vi "newlane2.vi"(11 "predict":bool=TRUE) -> ()   [LabVIEW 2012]
uses:
  G_NAV.vi
  G_VEH.vi
  G_PATH.vi
  G_SEN.vi
  <vilib>/Analysis/Matrix/Numeric/Conversions/Array To Matrix - RA2.vi
  <vilib>/Analysis/7linalg.llb/Real SVD Decomposition.vi
  <vilib>/Analysis/NI_AALPro.lvlib
  <vilib>/Analysis/Matrix/NI_Matrix.lvlib
panel:
  out "M6006":T1={"GPSTime"=22892800.0, "attitude[2]"=-0.6123908162117004, "lcc[0]"=-970.4720458984375, "lcc[1]"=200.52362060546875, "heading_GPS"=-0.610690712928772} {"GPSTime" format="%#_6f"}
  out "x-y":dbl[](array[numeric])
  out "min value 2":dbl
  out "min value":dbl
  out "Waveform Chart":dbl(graph)
  out "cost":dbl
  out "output array":dbl[][](array[numeric])
  out "rd0 2":dbl
  out "RXY":dbl[](array[numeric])=[73.97207949000635, 12.402968176654849, 69.25942811748455]
  out "map_track":dbl[][](array[numeric])=[[-0.6687401515638595, -3.551350516814976], [-1.1601880006125764, -3.4580278333550782], [-1.6512488590649952, -3.3629580799680854], [-2.1418835557610314, -3.265964418362822], [-2.6320529195405924, -3.1668700102479344], [-3.12171777924361, -3.0654980173321356], [-3.6108389637099756, -2.961671601324125], [-4.250355012057505, -2.8217269001890974], [-4.733554194697693, -2.693195492254268]]
  out "k 2":i32
  out "j 2":i32
  out "i 2":i32
  out "mapidx":i32[](array[numeric])
  out "ymin":dbl=-6.0
  out "ymax":dbl=12.0
  out "reverse":bool
  out "track":dbl[][](array[numeric])=[[-0.6687401515638595, -3.551350516814976], [-1.1601880006125764, -3.4580278333550782], [-1.6512488590649952, -3.3629580799680854], [-2.1418835557610314, -3.265964418362822], [-2.6320529195405924, -3.1668700102479344], [-3.12171777924361, -3.0654980173321356], [-3.6108389637099756, -2.961671601324125], [-4.250355012057505, -2.8217269001890974], [-4.733554194697693, -2.693195492254268], [-5.215089885143842, -2.558342659026822], [-5.693483406062963, -2.4115492889016945], [-6.167256080122039, -2.24719627027381], [-6.634929229988109, -2.059664491538052], [-7.095024178328142, -1.8433348410893422], [-7.546062247809149, -1.5925882073226139], [-7.98656476109811, -1.301805478632852], [-8.415053040862054, -0.9653675434148765], [-8.830048409767974, -0.5776552900636165], [-9.230072190482858, -0.133049606974057], [-9.61364570567371, 0.3740686174589265], [-9.97929027800753, 0.949318494840405], [-10.386059580111024, 1.7242186788508236], [-10.53357405922493, 2.2019628347040774], [-10.66851200140239, 2.6835902739278463], [-10.772007434080049, 3.1749262819640283], [-10.825194384694537, 3.6817961442544633], [-10.809206880682517, 4.210025146240928], [-10.705178949480636, 4.765438573365376], [-10.494244618525542, 5.353861711069529], [-10.157537915253862, 5.981119844795286], [-9.676192867102248, 6.653038259984428], [-8.946295802610212, 7.461572105302583], [-8.539313408094966, 7.752602995705581], [-8.110420661696207, 8.015244834208291], [-7.660232732059987, 8.25029468946181], [-7.189364787832295, 8.458549630117131], [-6.698431997659123, 8.640806724825243], [-6.188049530186491, 8.797863042237132], [-5.658832554060375, 8.930515651003796], [-5.11139623792681, 9.039561619776274], [-4.546355750431802, 9.12579801720561], [-3.9643262602213256, 9.190021911942688], [-3.3659229359414162, 9.233030372638604], [-2.7517609462380523, 9.25562046794435], [-2.122455459757251, 9.258589266510917], [-1.4786216451450183, 9.242733836989292], [-0.8208746710473604, 9.208851248030518], [-0.1498297061102689, 9.157738568285591], [0.5338980810202378, 9.090192866405497], [1.229693521698167, 9.007011211041284], [1.9369414472775146, 8.908990670843883], [2.6550266891122614, 8.796928314464337], [3.383334078556428, 8.671621210553642], [4.121248446963983, 8.53386642776284], [4.868154625688948, 8.384461034742866], [5.623437446085289, 8.224202100144819], [6.386481739507029, 8.053886692619635], [7.156672337308164, 7.874311880818305], [7.838146127104554, 7.70968069378327], [8.321781606815595, 7.582803343212244], [8.805290536895978, 7.45544776805299], [9.287663918083021, 7.323801011645703], [9.76789275111402, 7.18405011733063], [10.244968036726283, 7.032382128447967], [10.717880775657084, 6.864984088337955], [11.18562196864372, 6.678043040340844], [11.647182616423507, 6.4677460277968315], [12.101553719733744, 6.230280094046104], [12.547726279311707, 5.961832282428966], [12.984691295894704, 5.658589636285609], [13.411439770220039, 5.3167391989562285], [13.939637565704926, 4.818324597988705], [14.177469695018669, 4.377621822306417], [14.370305638929839, 3.9092831916317614], [14.522185803389362, 3.415790251277338], [14.637150594348116, 2.8996245465557346], [14.719240417757044, 2.363267622779441], [14.77249567956704, 1.8092010252611073], [14.800956785728996, 1.2399062993133256], [14.808664142193827, 0.6578649902486369], [14.799658154912459, 0.06555864337958095], [14.777979229835777, -0.5345311959811911]]
  out "xyhc":T2={"c_idx"=71, "xc"=-91.48037348905598, "yc"=-434.27857700428615, "hc"=-0.4484199308552679, "xc_path"=12.43286899562552}
  in  "usewpt":bool=TRUE
  out "left":dbl
  out "right":dbl
  out "lane left":dbl
  out "lane right":dbl
  out "maxradius":dbl=0.125
  out "Numeric":i32
  out "abrd0":dbl[][](array[numeric])
  out "center":dbl
  out "lane shift":dbl
  out "mylane":i16
  out "min lane length":dbl=0.125
  out "lineseed2":dbl[][](array[numeric])
  out "lineseed1":dbl[][](array[numeric])
  out "lineseed0":dbl[][](array[numeric])
  out "lineseedorigin":dbl[](array[numeric])
  out "den":dbl
  out "xx":dbl[](array[numeric])
  out "t2x":dbl
  out "xt":dbl[](array[numeric])
  out "rdi":dbl[](array[numeric])
  out "cta":dbl
  out "fitting?":bool
  out "mode":dbl
  out "rd0":dbl
  out "b":dbl
  out "a":dbl
  out "y":dbl[](array[numeric])
  out "x":dbl[](array[numeric])
  out "i":i32
  out "j":i32
  out "k":i32
  out "line":dbl[][](array[numeric])
  out "time[sec]":dbl
  out "count":cluster{dbl[][]}[](array[cluster])
  out "idxall":cluster{i32[]}[](array[cluster])
  out "yseed":dbl[](array[numeric])
  out "min lane width":dbl=0.125
  out "lane_resol":dbl=0.125
  out "T_threshold":dbl=0.125
  out "T_threshold 2":dbl=0.125
  out "xseed":dbl[](array[numeric])=[5.0, 10.0, 15.0, 20.0, 25.0, 30.0, 35.0]
  out "D_threshold":dbl=0.125
  out "data":dbl[][](array[numeric])
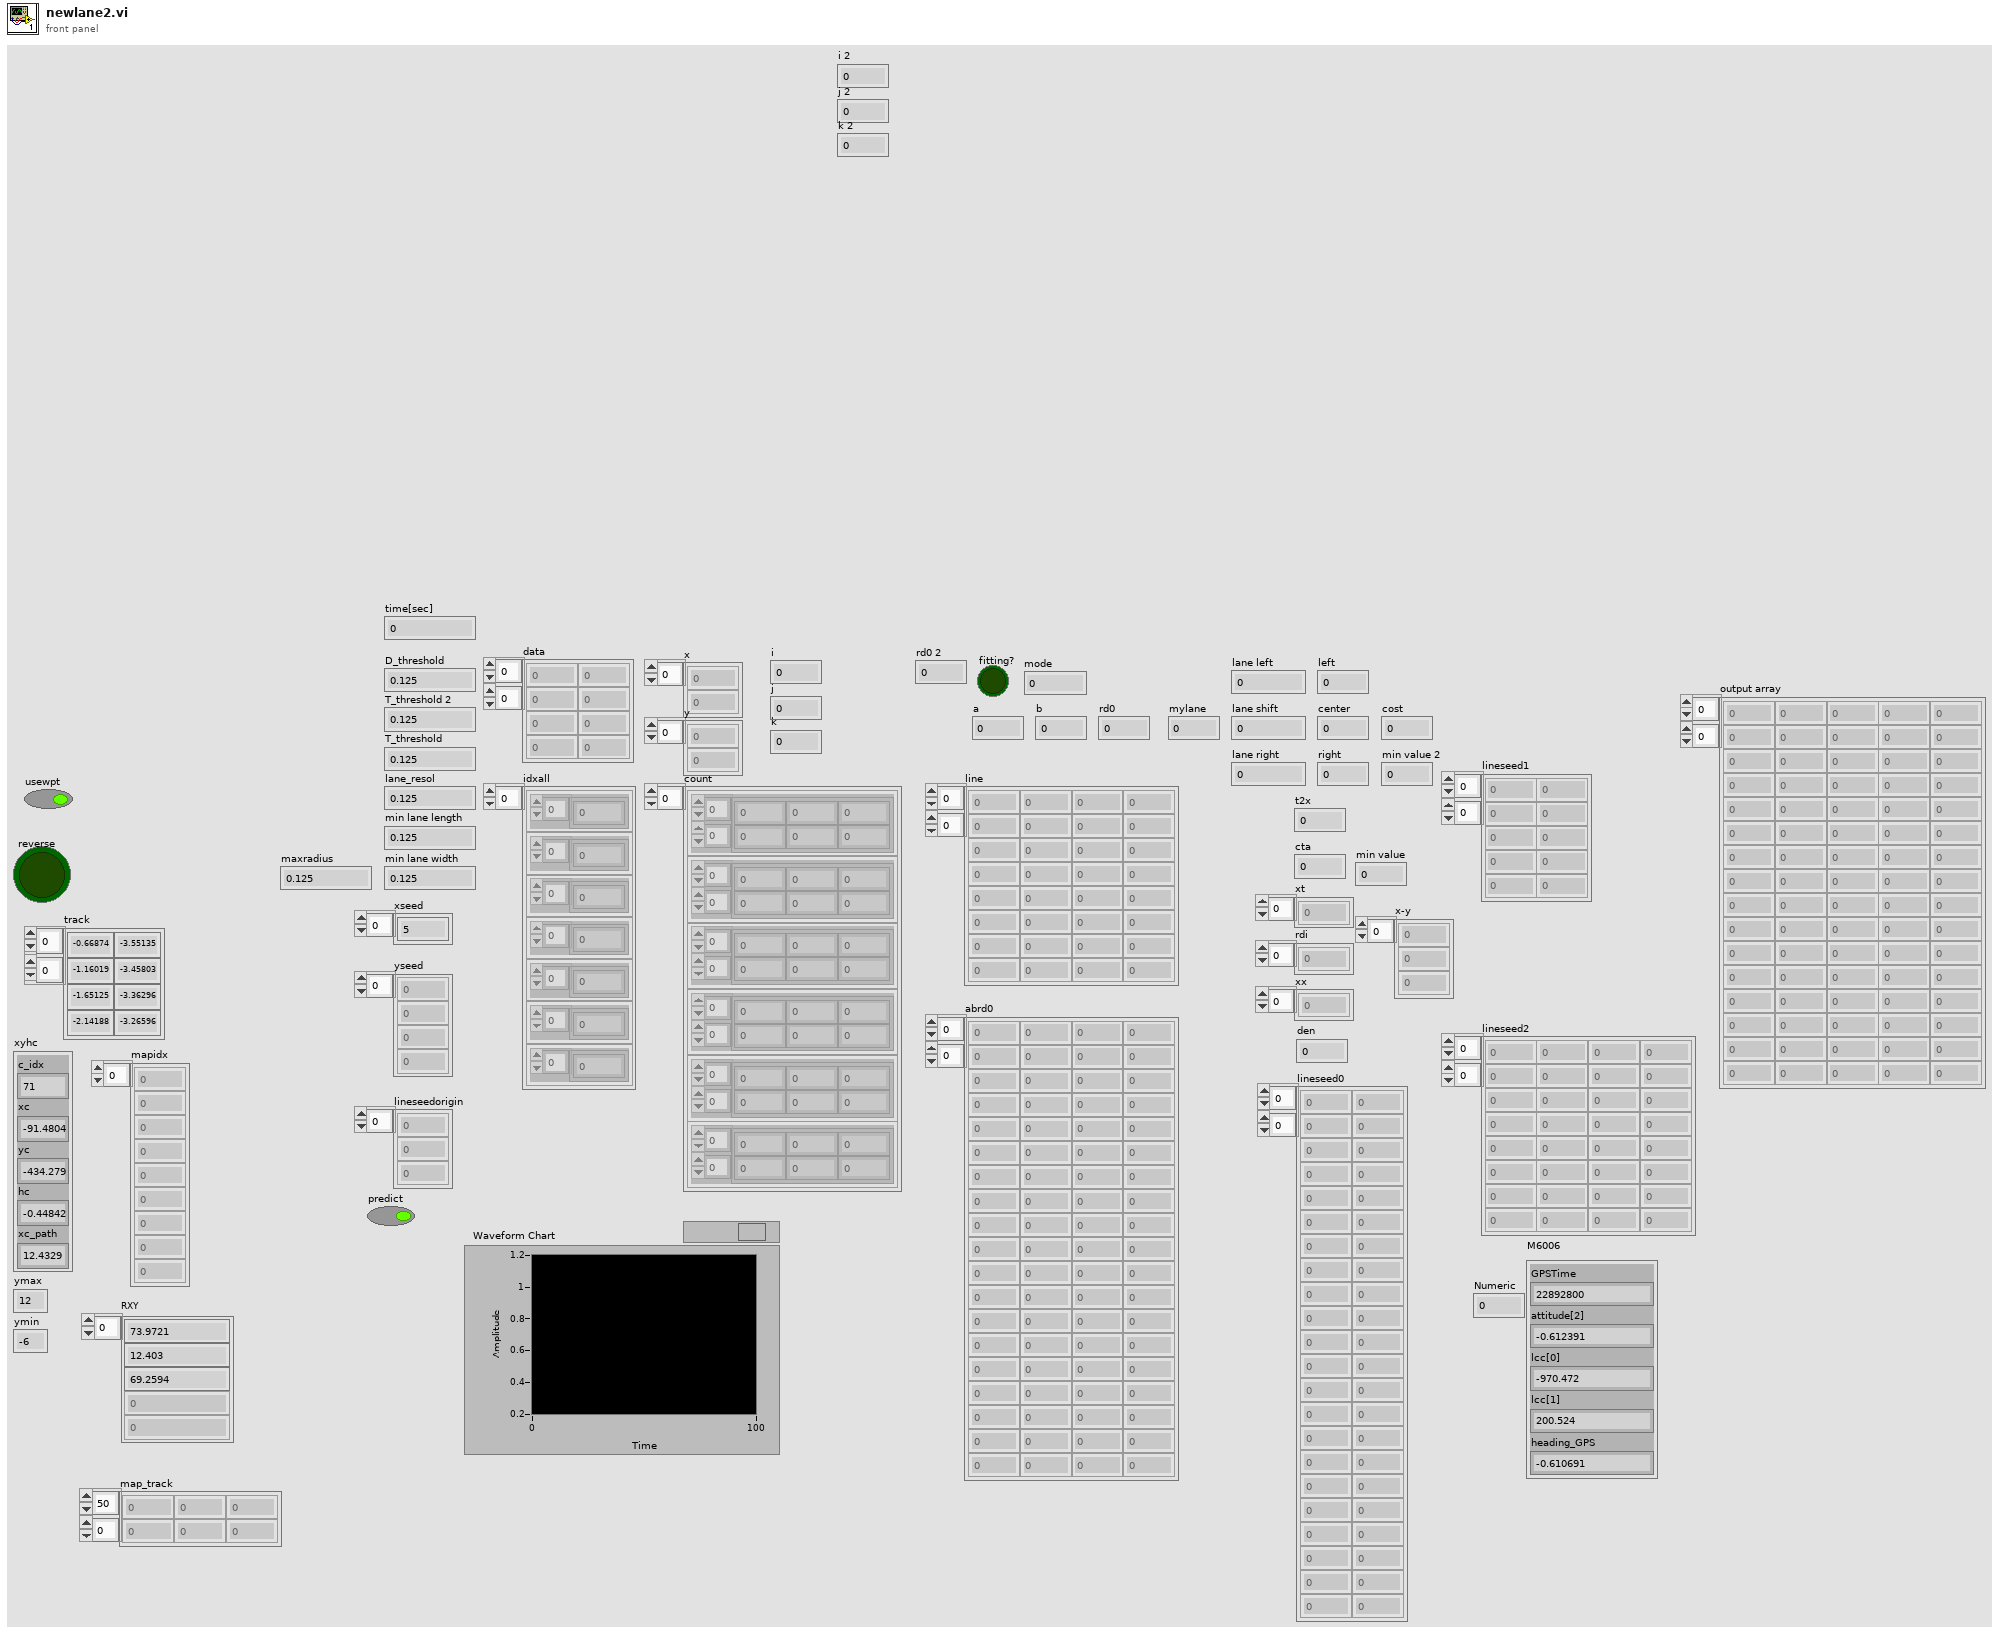
[diagram p1: front panel]
types:
  T1 = cluster{"GPSTime":dbl, "attitude[2]":dbl, "lcc[0]":dbl, "lcc[1]":dbl, "heading_GPS":dbl}
  T2 = cluster{"c_idx":i32, "xc":dbl, "yc":dbl, "hc":dbl, "xc_path":dbl}
  T3 = cluster{"idx":i32, "x":dbl, "y":dbl, "h":dbl, "x_path":dbl}
  T4 = cluster{"Steer_input":dbl, "Steer_output":dbl, "VS_des":dbl, "VS_can":dbl, "heading":dbl, "auto":bool, "run":bool, "x":dbl, "y":dbl}
  T5 = typedef "NI_Matrix.lvlib/RealMatrix.ctl" = dbl[][]
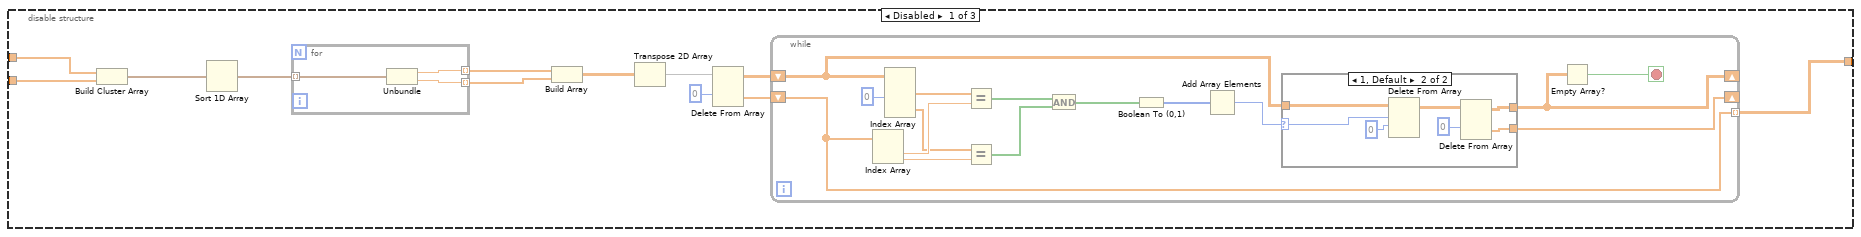
[diagram p5: hidden frame]
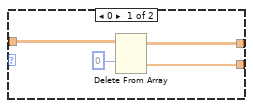
[diagram p6: hidden frame]
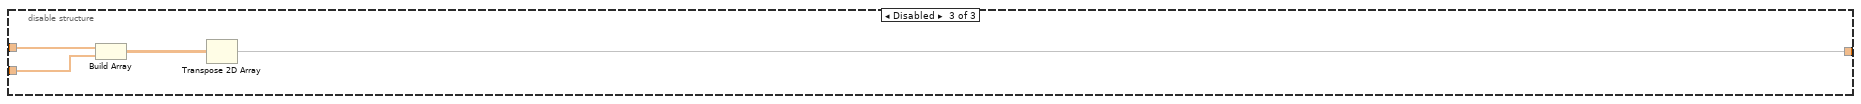
[diagram p8: hidden frame]
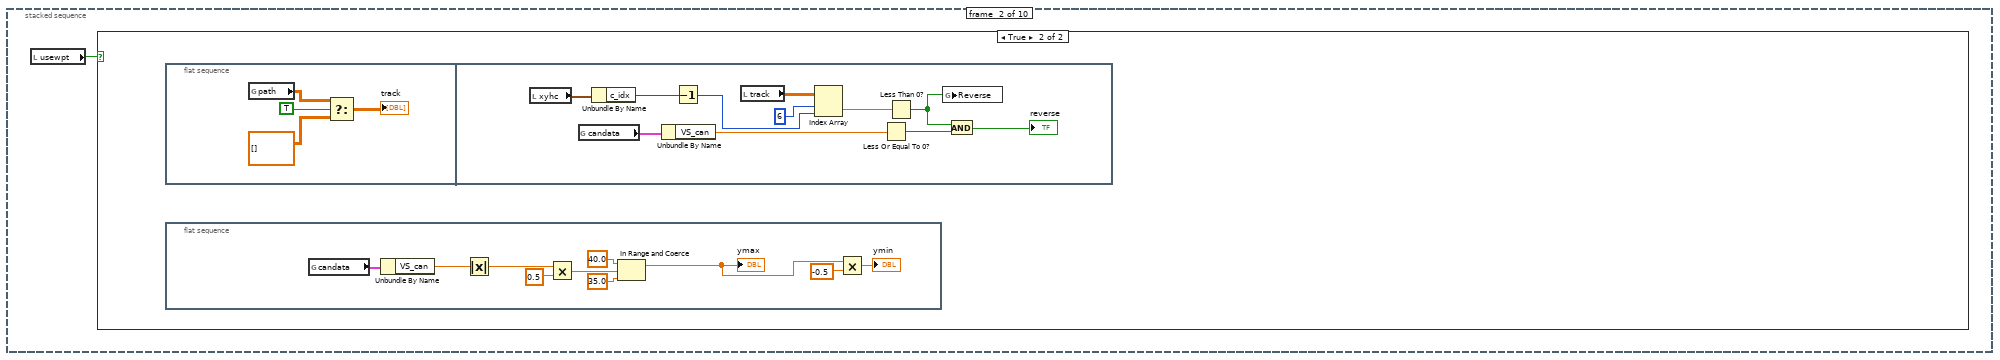
[diagram p11: hidden frame]
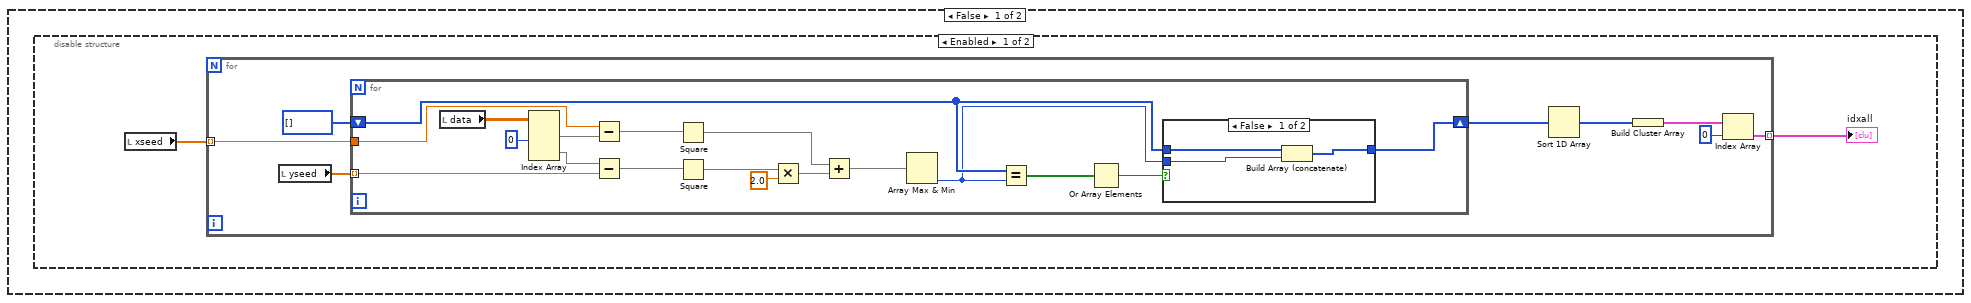
[diagram p12: hidden frame]
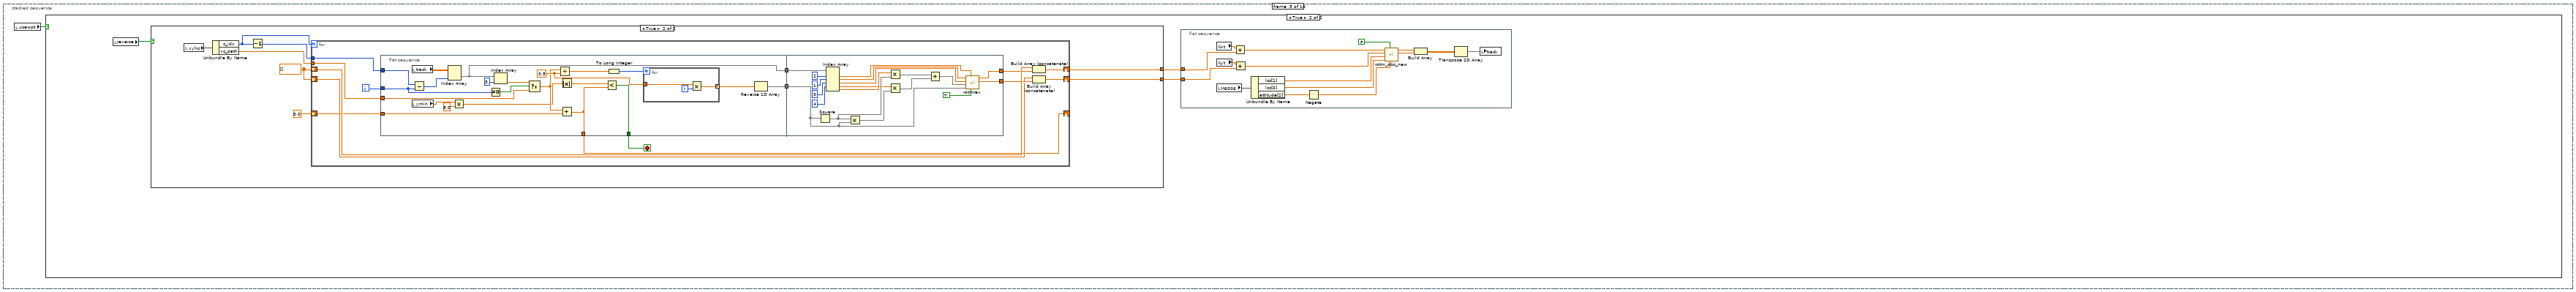
[diagram p15: hidden frame]
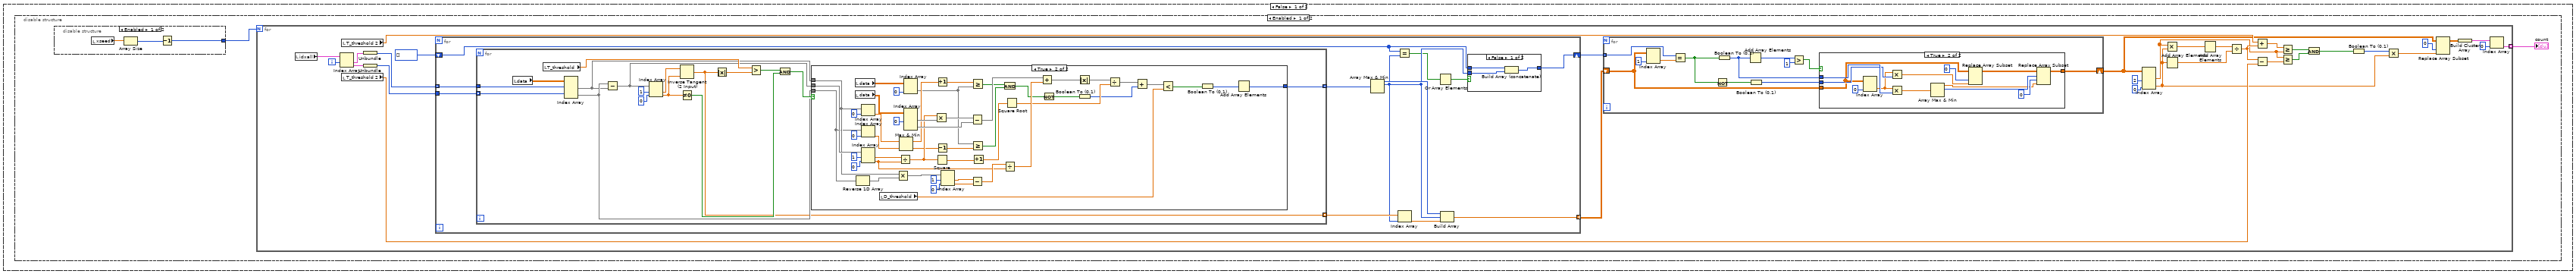
[diagram p16: hidden frame]
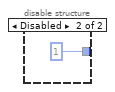
[diagram p20: hidden frame]
diagram:
  n1 = flat-sequence {
    tunnel: [w4] -> w2
    tunnel: [w11] -> w3
    tunnel: w2 -> [w11]
    tunnel: w3 -> [w57]
    tunnel: [w58] -> w1
    tunnel: w1 -> [w2451]
    frame #0 {
      n2 = Tick Count (ms)() -> (millisecond timer value=w4:u32)
    }
    frame #1 {
      n3 = global read "G_VEH.vi" "xyhc"() -> (w7:T3)
      n4 = global read "G_PATH.vi" "lane_init"() -> (w6:bool)
      n5 = global read "G_NAV.vi" "M6006"() -> (→"M6006":T1)
      n6 = Select(t=w7, s=TRUE ("B_track"), f=T2 {"c_idx"=0, "xc"=0.0, "yc"=0.0, "hc"=0.0, "xc_path"=0.0}) -> (s? t:f=→"xyhc":T2)
      n7 = case shown="False" w6 {
        frame False {
          n8 = flat-sequence {
            frame #0 {
              n9 = Multiply(x=5.0 ("D_threshold"), y=3.141592653589793) -> (x*y=w23:dbl)
              n10 = Multiply(x=15.0 ("D_threshold"), y=3.141592653589793) -> (x*y=w17:dbl)
              n11 = Divide(x=w17, y=180.0) -> (x/y=→"T_threshold":dbl)
              n12 = Divide(x=w23, y=180.0) -> (x/y=→"T_threshold 2":dbl)
              "D_threshold" <- 0.125 ("D_threshold")
              "lane_resol" <- 0.25 ("D_threshold")
              "min lane width" <- 2.5 ("D_threshold")
              "min lane length" <- 3.5 ("min lane length")
              "maxradius" <- 75.0 ("maxradius")
            }
            frame #1 {
              w31 = dbl[] [5.0, 10.0, 15.0, 20.0, 25.0, 30.0, 35.0]  # xseed
              w36 = 10.0
              w39 = 10.0
              n13 = local read "D_threshold"() -> (w33:dbl)
              n14 = Negate(x=w39) -> (-x=w38:dbl)
              n15 = Negate(x=w36) -> (-x=w37:dbl)
              n16 = Multiply(x=w33, y=4.0) -> (x*y=w41:dbl)
              n17 = Multiply(x=w33, y=1.0) -> (x*y=w35:dbl)
              n18 = Array Subset(array=w31, index=0, length=5) -> (→"xseed":dbl[])
              n19 = while {
                tunnel: w41 -> [w56]
                tunnel: [w50] -> w40 mode=indexing
                tunnel: w39 -> [w51]
                tunnel: w38 -> [w52]
                i -> [w55]
                stop <- w53 stop-if-true
                n20 = Multiply(x=w56, y=w55) -> (x*y=w54:dbl)
                n21 = Add(x=w52, y=w54) -> (x+y=w50:dbl)
                n22 = Less Or Equal?(x=w51, y=w50) -> (x <= y?=w53:bool)
              }
              "yseed" <- w40
              n23 = while {
                tunnel: w35 -> [w49]
                tunnel: [w43] -> w32 mode=indexing
                tunnel: w36 -> [w44]
                tunnel: w37 -> [w45]
                i -> [w48]
                stop <- w46 stop-if-true
                n24 = Multiply(x=w49, y=w48) -> (x*y=w47:dbl)
                n25 = Add(x=w45, y=w47) -> (x+y=w43:dbl)
                n26 = Less Or Equal?(x=w44, y=w43) -> (x <= y?=w46:bool)
              }
              "lineseedorigin" <- w32
            }
          }
          n27 = global write "G_PATH.vi" "lane_init"(TRUE ("lane_init")) -> ()
        }
        frame True {
        }
      }
    }
    frame #2 {
      n28 = stacked-sequence {
        tunnel: [w60 _ _ _ _ _ _ _ _ _] -> w58
        tunnel: w57 -> [w59 _ _ _ _ _ _ _ _ _]
        frame #0 {
          n29 = flat-sequence {
            tunnel: [w164] -> w60
            tunnel: w59 -> [w163]
            frame #0 {
              n30 = disable-structure shown="Enabled" {
                frame Enabled {
                  n31 = local read "M6006"() -> (w66:T1)
                  n32 = Unbundle By Name(w66) -> ("lcc[1]"=w83:dbl, "lcc[0]"=w82:dbl, "attitude[2]"=w81:dbl)
                  n33 = global read "G_SEN.vi" "sensor_lane_log"() -> (w77:dbl[][])
                  n34 = Negate(x=w81) -> (-x=w80:dbl)
                  n35 = Index Array(array=w77, index (col) #1=0 ("disabled index (col)")) -> (element #1=w79:dbl[], element #2=w78:dbl[])  [unwired: 3 in]
                  n36 = call "rotm_obs_new.vi"("angle[rad]"=w80, "y0"=w82, "x0"=w83, "y"=w78, "x"=w79) -> ("rot*(y-y0) 2"=w63:dbl[], "rot*(x-x0)"=w65:dbl[])  [unwired: 3 in, 2 out]
                  n37 = disable-structure shown="Enabled" {
                    disable-tunnel: w65 -> [w90 w94]
                    disable-tunnel: [w88 w94] -> w64
                    disable-tunnel: w63 -> [w87 w93]
                    disable-tunnel: [w85 w93] -> w62
                    frame Enabled {
                      n38 = global read "G_SEN.vi" "sensor_obs"() -> (w92:dbl[][])
                      n39 = Index Array(array=w92, index (col) #1=0 ("disabled index (col)")) -> (element #1=w89:dbl[], element #2=w86:dbl[])  [unwired: 3 in]
                      n40 = Build Array (concatenate)(w90, w89) -> (w88:dbl[])
                      n41 = Build Array (concatenate)(w87, w86) -> (w85:dbl[])
                    }
                    frame Disabled {
                    }
                  }
                  n42 = Multiply(x=w64, y=10.0) -> (x*y=w75:dbl[])
                  n43 = Multiply(x=w62, y=10.0) -> (x*y=w70:dbl[])
                  n44 = Round To Nearest(number=w75) -> (nearest integer value=w74:dbl[])
                  n45 = Round To Nearest(number=w70) -> (nearest integer value=w71:dbl[])
                  n46 = Multiply(x=w71, y=0.1) -> (x*y=w68:dbl[])
                  n47 = Multiply(x=w74, y=-0.1) -> (x*y=w67:dbl[])
                  n48 = disable-structure shown="Enabled" {
                    disable-tunnel: [w95 w138 w159] -> w61
                    disable-tunnel: w68 -> [w105 w137 w162]
                    disable-tunnel: w67 -> [w104 w136 w161]
                    frame Disabled {
                      n49 = Build Cluster Array(w105, w104) -> (w106:cluster{dbl, dbl}[])
                      n50 = Sort 1D Array(array=w106) -> (sorted array=w103:cluster{dbl, dbl}[])
                      n51 = for {
                        tunnel: w103 -> [w135] mode=indexing
                        tunnel: [w134] -> w102 mode=indexing
                        tunnel: [w133] -> w101 mode=indexing
                        n52 = Unbundle(w135) -> (w134:dbl, w133:dbl)
                      }
                      n53 = Build Array(w102, w101) -> (w100:dbl[][])
                      n54 = Transpose 2D Array(2D array=w100) -> (transposed array=w99:dbl[][])
                      n55 = Delete From Array(array=w99, index (row)=0) -> (deleted portion=w98:dbl[], array with subset deleted=w97:dbl[][])  [unwired: 2 in]
                      n56 = while {
                        shift-right: [w109] -> _
                        shift-left: w98 -> [w108]
                        shift-right: [w111] -> _
                        shift-left: w97 -> [w112]
                        tunnel: [w108] -> w95 mode=indexing
                        stop <- w110 stop-if-true
                        n57 = Index Array(array=w108) -> (element #1=w119:dbl, element #2=w117:dbl)  [unwired: 2 in]
                        n58 = Index Array(array=w112, index (col) #1=0 ("disabled index (col)")) -> (element #1=w120:dbl[], element #2=w118:dbl[])  [unwired: 3 in]
                        n59 = Equal?(x=w120, y=w119) -> (x = y?=w116:bool[])
                        n60 = Equal?(x=w118, y=w117) -> (x = y?=w115:bool[])
                        n61 = And(x=w116, y=w115) -> (x .and. y?=w114:bool[])
                        n62 = Boolean To (0,1)(Boolean=w114) -> (0, 1=w113:i16[])
                        n63 = Add Array Elements(numeric array=w113) -> (sum=w107:i16)
                        n64 = case shown="1, Default" w107 {
                          selector: w107 -> [_ w131]
                          tunnel: w112 -> [w125 w132]
                          tunnel: [w124 w129] -> w111
                          tunnel: [w123 w128] -> w109
                          frame 0 {
                            n65 = Delete From Array(array=w125, index (row)=0) -> (deleted portion=w123:dbl[], array with subset deleted=w124:dbl[][])  [unwired: 2 in]
                          }
                          frame 1, Default {
                            n66 = Delete From Array(array=w132, length=w131, index (row)=0) -> (array with subset deleted=w130:dbl[][])  [unwired: 1 in, 1 out]
                            n67 = Delete From Array(array=w130, index (row)=0) -> (deleted portion=w128:dbl[], array with subset deleted=w129:dbl[][])  [unwired: 2 in]
                          }
                        }
                        n68 = Empty Array?(array=w111) -> (empty?=w110:bool)
                      }
                    }
                    frame Enabled {
                      n69 = Build Cluster Array(w137, w136) -> (w142:cluster{dbl, dbl}[])
                      n70 = Sort 1D Array(array=w142) -> (sorted array=w141:cluster{dbl, dbl}[])
                      n71 = for {
                        tunnel: w141 -> [w154] mode=indexing
                        shift-right: [w150] -> _
                        shift-left: dbl[] [-1e+18, -1e+18] -> [w149]
                        shift-right: [w152] -> w138
                        shift-left: dbl[][] [] -> [w153]
                        stop <- w143 stop-if-true
                        n72 = Unbundle(w154) -> (w147:dbl, w148:dbl)
                        n73 = Build Array(w147, w148) -> (w150:dbl[])
                        n74 = Greater?(x=w147, y=40.0) -> (0:w143:bool)
                        n75 = Equal?(x=w150, y=w149) -> (x = y?=w151:bool[])
                        n76 = And Array Elements(Boolean array=w151) -> (logical AND=w144:bool)
                        n77 = Or(x=w143, y=w144) -> (x .or. y?=w145:bool)
                        n78 = case shown="False" w145 {
                          tunnel: w153 -> [w157 w158]
                          tunnel: w150 -> [w156 _]
                          tunnel: [w155 w158] -> w152
                          frame False {
                            n79 = Build Array (concatenate)(w157, w156) -> (w155:dbl[][])
                          }
                          frame True {
                          }
                        }
                      }
                    }
                    frame Disabled {
                      n80 = Build Array(w162, w161) -> (w160:dbl[][])
                      n81 = Transpose 2D Array(2D array=w160) -> (transposed array=w159:dbl[][])
                    }
                  }
                  "data" <- w61
                }
                frame Disabled {
                }
              }
            }
            frame #1 {
              n82 = disable-structure shown="Enabled" {
                disable-tunnel: [w165 w166] -> w164
                disable-tunnel: w163 -> [_ w166]
                frame Enabled {
                  n83 = Tick Count (ms)() -> (millisecond timer value=w165:u32)
                }
                frame Disabled {
                }
              }
            }
          }
        }
        frame #1 {
          n84 = local read "usewpt"() -> (w167:bool)
          n85 = case shown="True" w167 {
            frame False {
              n86 = disable-structure shown="Enabled" {
                frame Enabled {
                  n87 = local read "xseed"() -> (w169:dbl[])
                  n88 = for {
                    tunnel: w169 -> [w176] mode=indexing
                    tunnel: [w170] -> w168 mode=indexing
                    n89 = local read "yseed"() -> (w177:dbl[])
                    n90 = for {
                      tunnel: w177 -> [w192] mode=indexing
                      tunnel: w176 -> [w179]
                      shift-right: [w184] -> w174
                      shift-left: i32[] [] -> [w185]
                      n91 = local read "data"() -> (w195:dbl[][])
                      n92 = Index Array(array=w195, index (col) #1=0 ("disabled index (col)")) -> (element #1=w178:dbl[], element #2=w193:dbl[])  [unwired: 3 in]
                      n93 = Subtract(x=w179, y=w178) -> (x-y=w191:dbl[])
                      n94 = Subtract(x=w193, y=w192) -> (x-y=w190:dbl[])
                      n95 = Square(x=w191) -> (x^2=w189:dbl[])
                      n96 = Square(x=w190) -> (x^2=w182:dbl[])
                      n97 = Multiply(x=w182, y=2.0) -> (x*y=w180:dbl[])
                      n98 = Add(x=w189, y=w180) -> (x+y=w188:dbl[])
                      n99 = Array Max & Min(array=w188) -> (min index (indices)=w183:i32)  [unwired: 3 out]
                      n100 = Equal?(x=w185, y=w183) -> (x = y?=w187:bool[])
                      n101 = Or Array Elements(Boolean array=w187) -> (logical OR=w186:bool)
                      n102 = case shown="False" w186 {
                        tunnel: w185 -> [w198 w199]
                        tunnel: w183 -> [w197 _]
                        tunnel: [w196 w199] -> w184
                        frame False {
                          n103 = Build Array (concatenate)(w198, w197) -> (w196:i32[])
                        }
                        frame True {
                        }
                      }
                    }
                    n104 = Sort 1D Array(array=w174) -> (sorted array=w173:i32[])
                    n105 = Build Cluster Array(w173) -> (w172:cluster{i32[]}[])
                    n106 = Index Array(array=w172, index=0) -> (element=w170:cluster{i32[]})
                  }
                  "idxall" <- w168
                }
                frame Disabled {
                }
              }
            }
            frame True {
              n107 = flat-sequence {
                frame #0 {
                  n108 = global read "G_PATH.vi" "path"() -> (w210:dbl[][])
                  n109 = Select(t=w210, s=TRUE ("B_track"), f=dbl[][] []) -> (s? t:f=→"track":dbl[][])
                }
                frame #1 {
                  n110 = local read "xyhc"() -> (w223:T2)
                  n111 = global read "G_VEH.vi" "candata"() -> (w217:T4)
                  n112 = Unbundle By Name(w223) -> ("c_idx"=w221:i32)
                  n113 = Unbundle By Name(w217) -> ("VS_can"=w218:dbl)
                  n114 = Decrement(x=w221) -> (x-1=w222:i32)
                  n115 = local read "track"() -> (w224:dbl[][])
                  n116 = Index Array(array=w224, index (row)=6, index (col)=w222) -> (element=w219:dbl)
                  n117 = Less Or Equal To 0?(x=w218) -> (x <= 0?=w215:bool)
                  n118 = Less Than 0?(x=w219) -> (x < 0?=w216:bool)
                  n119 = global write "G_VEH.vi" "Reverse"(w216) -> ()
                  n120 = And(x=w216, y=w215) -> (x .and. y?=→"reverse":bool)
                }
              }
              n121 = flat-sequence {
                frame #0 {
                  n122 = global read "G_VEH.vi" "candata"() -> (w203:T4)
                  n123 = Unbundle By Name(w203) -> ("VS_can"=w206:dbl)
                  n124 = Absolute Value(x=w206) -> (abs(x)=w207:dbl)
                  n125 = Multiply(x=w207, y=0.5 ("vgain")) -> (x*y=w208:dbl)
                  n126 = In Range and Coerce(upper limit=40.0, x=w208, lower limit=35.0 ("y")) -> (coerced(x)=w200:dbl)  [unwired: 1 out]
                  "ymax" <- w200
                  n127 = Multiply(x=w200, y=-0.5) -> (x*y=→"ymin":dbl)
                }
              }
            }
          }
        }
        frame #2 {
          n128 = local read "usewpt"() -> (w225:bool)
          n129 = case shown="True" w225 {
            frame False {
              n130 = disable-structure shown="Enabled" {
                frame Enabled {
                  n131 = disable-structure shown="Enabled" {
                    disable-tunnel: [w368 1] -> w227
                    frame Enabled {
                      n132 = local read "xseed"() -> (w370:dbl[])
                      n133 = Array Size(array=w370) -> (size(s)=w369:i32)
                      n134 = Decrement(x=w369) -> (x-1=w368:i32)
                    }
                    frame Disabled {
                    }
                  }
                  n135 = for {
                    N: w227 -> [_]
                    tunnel: [w234] -> w226 mode=indexing
                    i -> [w258]
                    n136 = local read "idxall"() -> (w259:cluster{i32[]}[])
                    n137 = Index Array(array=w259, index #1=w258) -> (element #1=w257:cluster{i32[]}, element #2=w255:cluster{i32[]})  [unwired: 1 in]
                    n138 = local read "T_threshold 2"() -> (w245:dbl)
                    n139 = local read "T_threshold 2"() -> (w243:dbl)
                    n140 = Unbundle(w257) -> (w256:i32[])
                    n141 = Unbundle(w255) -> (w254:i32[])
                    n142 = for {
                      tunnel: w256 -> [w296] mode=indexing
                      tunnel: w254 -> [w297]
                      shift-right: [w291] -> w252
                      shift-left: i32[] [] -> [w290]
                      tunnel: [w286] -> w251 mode=indexing
                      n143 = for {
                        tunnel: w297 -> [w316] mode=indexing
                        tunnel: w296 -> [w317]
                        tunnel: [w303] -> w295 mode=indexing
                        tunnel: [w302] -> w294 mode=indexing
                        n144 = local read "data"() -> (w318:dbl[][])
                        n145 = local read "T_threshold"() -> (w312:dbl)
                        n146 = Index Array(array=w318, index (row) #1=w317, index (row) #2=w316) -> (element #1=w304:dbl[], element #2=w305:dbl[])  [unwired: 2 in]
                        n147 = Subtract(x=w305, y=w304) -> (x-y=w306:dbl[])
                        n148 = Index Array(array=w306, index #1=1 ("index"), index #2=0 ("index")) -> (element #1=w313:dbl, element #2=w310:dbl)
                        n149 = Inverse Tangent (2 Input)(1:w310, 2:w313) -> (0:w302:dbl)
                        n150 = Not Equal To 0?(x=w310) -> (x != 0?=w308:bool)
                        n151 = Absolute Value(x=w302) -> (abs(x)=w311:dbl)
                        n152 = Greater?(x=w312, y=w311) -> (0:w309:bool)
                        n153 = And(x=w309, y=w308) -> (x .and. y?=w307:bool)
                        n154 = case shown="True" w307 {
                          tunnel: w306 -> [_ w365]
                          tunnel: w305 -> [_ w339]
                          tunnel: w304 -> [_ w342]
                          tunnel: [_ w325] -> w303
                          frame False {
                          }
                          frame True {
                            n155 = local read "data"() -> (w333:dbl[][])
                            n156 = local read "data"() -> (w355:dbl[][])
                            n157 = Reverse 1D Array(array=w339) -> (reversed array=w363:dbl[])
                            n158 = Index Array(array=w342, index=0) -> (element=w338:dbl)
                            n159 = Index Array(array=w339, index=0) -> (element=w337:dbl)
                            n160 = Index Array(array=w365, index #1=1 ("index"), index #2=0 ("index")) -> (element #1=w364:dbl, element #2=w356:dbl)
                            n161 = local read "D_threshold"() -> (w329:dbl)
                            n162 = Multiply(x=w342, y=w363) -> (x*y=w361:dbl[])
                            n163 = Divide(x=w364, y=w356) -> (x/y=w347:dbl)
                            n164 = Max & Min(x=w338, y=w337) -> (max(x,y)=w336:dbl, min(x,y)=w335:dbl)
                            n165 = Index Array(array=w333, index (col)=0 ("disabled index (col)")) -> (element=w323:dbl[])  [unwired: 1 in]
                            n166 = Index Array(array=w355, index (col) #1=0 ("disabled index (col)")) -> (element #1=w353:dbl[], element #2=w351:dbl[])  [unwired: 3 in]
                            n167 = Multiply(x=w347, y=w353) -> (x*y=w352:dbl[])
                            n168 = Square(x=w347) -> (x^2=w346:dbl)
                            n169 = Increment(x=w336) -> (x+1=w324:dbl)
                            n170 = Decrement(x=w335) -> (x-1=w322:dbl)
                            n171 = Index Array(array=w361, index #1=1 ("index"), index #2=0 ("index")) -> (element #1=w360:dbl, element #2=w359:dbl)
                            n172 = Subtract(x=w352, y=w351) -> (x-y=w350:dbl[])
                            n173 = Subtract(x=w360, y=w359) -> (x-y=w357:dbl)
                            n174 = Greater Or Equal?(x=w324, y=w323) -> (x >= y?=w320:bool[])
                            n175 = Greater Or Equal?(x=w323, y=w322) -> (x >= y?=w321:bool[])
                            n176 = Increment(x=w346) -> (x+1=w345:dbl)
                            n177 = And(x=w320, y=w321) -> (x .and. y?=w319:bool[])
                            n178 = Divide(x=w357, y=w356) -> (x/y=w349:dbl)
                            n179 = Square Root(x=w345) -> (sqrt(x)=w343:dbl)
                            n180 = Add(x=w350, y=w349) -> (x+y=w348:dbl[])
                            n181 = Not(x=w319) -> (.not. x?=w332:bool[])
                            n182 = Absolute Value(x=w348) -> (abs(x)=w344:dbl[])
                            n183 = Boolean To (0,1)(Boolean=w332) -> (0, 1=w330:i16[])
                            n184 = Divide(x=w344, y=w343) -> (x/y=w331:dbl[])
                            n185 = Add(x=w331, y=w330) -> (x+y=w328:dbl[])
                            n186 = Less?(x=w328, y=w329) -> (x < y?=w327:bool[])
                            n187 = Boolean To (0,1)(Boolean=w327) -> (0, 1=w326:i16[])
                            n188 = Add Array Elements(numeric array=w326) -> (sum=w325:i16)
                          }
                        }
                      }
                      n189 = Array Max & Min(array=w295) -> (max value=w293:i16, max index (indices)=w289:i32)  [unwired: 2 out]
                      n190 = Equal?(x=w290, y=w289) -> (x = y?=w288:bool[])
                      n191 = Index Array(array=w294, index=w289) -> (element=w292:dbl)
                      n192 = Or Array Elements(Boolean array=w288) -> (logical OR=w287:bool)
                      n193 = Build Array(w293, w289, w292) -> (w286:dbl[])
                      n194 = case shown="False" w287 {
                        tunnel: w289 -> [w300 _]
                        tunnel: [w299 w301] -> w291
                        tunnel: w290 -> [w298 w301]
                        frame False {
                          n195 = Build Array (concatenate)(w298, w300) -> (w299:i32[])
                        }
                        frame True {
                        }
                      }
                    }
                    n196 = for {
                      tunnel: w252 -> [w270] mode=indexing
                      shift-right: [w260] -> w242
                      shift-left: w251 -> [w265]
                      n197 = Index Array(array=w265, index (col)=1 ("disabled index (col)")) -> (element=w269:dbl[])  [unwired: 1 in]
                      n198 = Equal?(x=w270, y=w269) -> (x = y?=w263:bool[])
                      n199 = Not(x=w263) -> (.not. x?=w262:bool[])
                      n200 = Boolean To (0,1)(Boolean=w263) -> (0, 1=w264:i16[])
                      n201 = Add Array Elements(numeric array=w264) -> (sum=w268:i16)
                      n202 = Boolean To (0,1)(Boolean=w262) -> (0, 1=w261:i16[])
                      n203 = Greater?(x=w268, y=i16 1) -> (0:w266:bool)
                      n204 = case shown="True" w266 {
                        tunnel: w265 -> [w272 w280]
                        tunnel: w264 -> [_ w284]
                        tunnel: w261 -> [_ w282]
                        tunnel: [w272 w273] -> w260
                        frame False {
                        }
                        frame True {
                          n205 = Index Array(array=w280, index (col)=0 ("disabled index (col)")) -> (element=w281:dbl[])  [unwired: 1 in]
                          n206 = Multiply(x=w281, y=w282) -> (x*y=w278:dbl[])
                          n207 = Multiply(x=w281, y=w284) -> (x*y=w283:dbl[])
                          n208 = Array Max & Min(array=w283) -> (max value=w274:dbl, max index (indices)=w275:i32)  [unwired: 2 out]
                          n209 = Replace Array Subset(array=w280, new element=w278, index (col)=0 ("disabled index (col)")) -> (w277:dbl[][])  [unwired: 1 in]
                          n210 = Replace Array Subset(array=w277, new element=w274, index (row)=w275, index (col)=0 ("disabled index (col)")) -> (w273:dbl[][])
                        }
                      }
                    }
                    n211 = Index Array(array=w242, index (col) #1=2 ("disabled index (col)"), index (col) #2=0 ("disabled index (col)")) -> (element #1=w232:dbl[], element #2=w240:dbl[])  [unwired: 2 in]
                    n212 = Multiply(x=w232, y=w240) -> (x*y=w248:dbl[])
                    n213 = Add Array Elements(numeric array=w240) -> (sum=w246:dbl)
                    n214 = Add Array Elements(numeric array=w248) -> (sum=w247:dbl)
                    n215 = Divide(x=w247, y=w246) -> (x/y=w244:dbl)
                    n216 = Add(x=w245, y=w244) -> (x+y=w233:dbl)
                    n217 = Subtract(x=w244, y=w243) -> (x-y=w231:dbl)
                    n218 = Greater Or Equal?(x=w233, y=w232) -> (x >= y?=w230:bool[])
                    n219 = Greater Or Equal?(x=w232, y=w231) -> (x >= y?=w229:bool[])
                    n220 = And(x=w230, y=w229) -> (x .and. y?=w228:bool[])
                    n221 = Boolean To (0,1)(Boolean=w228) -> (0, 1=w239:i16[])
                    n222 = Multiply(x=w239, y=w240) -> (x*y=w238:dbl[])
                    n223 = Replace Array Subset(array=w242, new element=w238, index (col)=0 ("disabled index (col)")) -> (w235:dbl[][])  [unwired: 1 in]
                    n224 = Build Cluster Array(w235) -> (w237:cluster{dbl[][]}[])
                    n225 = Index Array(array=w237, index=0) -> (element=w234:cluster{dbl[][]})
                  }
                  "count" <- w226
                }
                frame Disabled {
                }
              }
            }
            frame True {
              n226 = local read "reverse"() -> (w374:bool)
              n227 = case shown="True" w374 {
                tunnel: [w395 w471] -> w372
                tunnel: [w394 w470] -> w373
                frame False {
                  w397 = dbl[] [] ("x")
                  n228 = local read "track"() -> (w392:dbl[][])
                  n229 = local read "xyhc"() -> (w391:T2)
                  n230 = Unbundle By Name(w391) -> ("c_idx"=w403:i32, "xc_path"=w398:dbl)
                  n231 = Array Size(array=w392) -> (size(s)=w402:i32[])
                  n232 = Decrement(x=w403) -> (x-1=w399:i32)
                  n233 = Index Array(array=w402, index=1) -> (element=w400:i32)
                  n234 = Subtract(x=w400, y=w399) -> (x-y=w396:i32)
                  n235 = for {
                    N: w396 -> [_]
                    tunnel: w399 -> [w417]
                    shift-right: [0.0 ("xc_path")] -> _
                    shift-left: w398 -> [w415]
                    shift-right: [w410] -> w395
                    shift-left: w397 -> [w411]
                    shift-right: [w407] -> w394
                    shift-left: w397 -> [w408]
                    shift-right: [w405] -> _
                    shift-left: 0.0 -> [w406]
                    i -> [w418]
                    stop <- w404 stop-if-true
                    n236 = flat-sequence {
                      tunnel: w418 -> [w442]
                      tunnel: w417 -> [w441]
                      tunnel: w415 -> [w435]
                      tunnel: [w433] -> w414
                      tunnel: [w432] -> w413
                      tunnel: w406 -> [w430]
                      tunnel: [w429] -> w405
                      tunnel: [w428] -> w404
                      tunnel: w414 -> [w458]
                      tunnel: w413 -> [w459]
                      tunnel: [w450] -> w412
                      tunnel: [w449] -> w409
                      frame #0 {
                        w434 = 0.5 ("y")
                        n237 = local read "ymax"() -> (w426:dbl)
                        n238 = local read "track"() -> (w427:dbl[][])
                        n239 = Add(x=w441, y=w442) -> (x+y=w440:i32)
                        n240 = global read "G_PATH.vi" "Mission"() -> (w419:i32)
                        n241 = Index Array(array=w427, index (col)=w440) -> (element=w432:dbl[])  [unwired: 1 in]
                        n242 = Multiply(x=5.0 ("f"), y=w426) -> (x*y=w421:dbl)
                        n243 = Equal?(x=w419, y=3) -> (x = y?=w424:bool)
                        n244 = Index Array(array=w432, index=3) -> (element=w438:dbl)
                        n245 = Subtract(x=w438, y=w435) -> (x-y=w431:dbl)
                        n246 = Select(t=100.0 ("x"), s=w424, f=w421) -> (s? t:f=w420:dbl)
                        n247 = Divide(x=w431, y=w434) -> (x/y=w437:dbl)
                        n248 = Add(x=w431, y=w430) -> (x+y=w429:dbl)
                        n249 = Less?(x=w420, y=w429) -> (x < y?=w428:bool)
                        n250 = To Long Integer(number=w437) -> (32bit integer=w436:i32)
                        n251 = for {
                          N: w436 -> [_]
                          tunnel: w435 -> [w443]
                          tunnel: w434 -> [w446]
                          tunnel: [w445] -> w433 mode=indexing
                          i -> [w447]
                          n252 = Multiply(x=w446, y=w447) -> (x*y=w444:dbl)
                          n253 = Add(x=w444, y=w443) -> (x+y=w445:dbl)
                        }
                      }
                      frame #1 {
                        n254 = Square(x=w458) -> (x^2=w464:dbl[])
                        n255 = Index Array(array=w459, index #1=2 ("index"), index #2=1 ("index"), index #3=0 ("index"), index #4=4 ("index")) -> (element #1=w453:dbl, element #2=w452:dbl, element #3=w451:dbl, element #4=w463:dbl, element #5=w465:dbl)  [unwired: 1 in]
                        n256 = Multiply(x=w464, y=w458) -> (x*y=w462:dbl[])
                        n257 = Multiply(x=w465, y=w464) -> (x*y=w461:dbl[])
                        n258 = Multiply(x=w463, y=w462) -> (x*y=w460:dbl[])
                        n259 = Add(x=w461, y=w460) -> (x+y=w457:dbl[])
                        n260 = call "rotmrev.vi"("reverse"=TRUE, "angle[rad]"=w453, "x"=w458, "y"=w457, "x0"=w451, "y0"=w452) -> ("y"=w449:dbl[], "x"=w450:dbl[])  [unwired: 4 in]
                      }
                    }
                    n261 = Build Array (concatenate)(w408, w409) -> (w407:dbl[])
                    n262 = Build Array (concatenate)(w411, w412) -> (w410:dbl[])
                  }
                }
                frame True {
                  w472 = dbl[] [] ("x")
                  n263 = local read "xyhc"() -> (w467:T2)
                  n264 = Unbundle By Name(w467) -> ("c_idx"=w469:i32, "xc_path"=w473:dbl)
                  n265 = Decrement(x=w469) -> (x-1=w474:i32)
                  n266 = for {
                    N: w469 -> [_]
                    tunnel: w474 -> [w487]
                    shift-right: [w481] -> w471
                    shift-left: w472 -> [w482]
                    shift-right: [w478] -> w470
                    shift-left: w472 -> [w479]
                    tunnel: w473 -> [w486]
                    shift-right: [w476] -> _
                    shift-left: 0.0 -> [w477]
                    i -> [w488]
                    stop <- w475 stop-if-true
                    n267 = flat-sequence {
                      tunnel: w488 -> [w503]
                      tunnel: w487 -> [w510]
                      tunnel: w486 -> [w500]
                      tunnel: [w498] -> w485
                      tunnel: [w504] -> w484
                      tunnel: w477 -> [w496]
                      tunnel: [w495] -> w476
                      tunnel: [w494] -> w475
                      tunnel: w485 -> [w524]
                      tunnel: w484 -> [w525]
                      tunnel: [w516] -> w483
                      tunnel: [w515] -> w480
                      frame #0 {
                        w505 = 0.5 ("y")
                        n268 = local read "track"() -> (w493:dbl[][])
                        n269 = local read "ymin"() -> (w491:dbl)
                        n270 = Subtract(x=w510, y=w503) -> (x-y=w509:i32)
                        n271 = Index Array(array=w493, index (col)=w509) -> (element=w504:dbl[])  [unwired: 1 in]
                        n272 = Multiply(x=w491, y=5.0) -> (x*y=w490:dbl)
                        n273 = Not Equal To 0?(x=w503) -> (x != 0?=w502:bool)
                        n274 = Index Array(array=w504, index=3) -> (element=w501:dbl)
                        n275 = Select(t=w501, s=w502, f=w500) -> (s? t:f=w497:dbl)
                        n276 = Divide(x=w497, y=w505) -> (x/y=w507:dbl)
                        n277 = Absolute Value(x=w490) -> (abs(x)=w492:dbl)
                        n278 = Add(x=w497, y=w496) -> (x+y=w495:dbl)
                        n279 = Less?(x=w492, y=w495) -> (x < y?=w494:bool)
                        n280 = To Long Integer(number=w507) -> (32bit integer=w506:i32)
                        n281 = for {
                          N: w506 -> [_]
                          tunnel: w505 -> [w512]
                          tunnel: [w511] -> w499 mode=indexing
                          i -> [w513]
                          n282 = Multiply(x=w512, y=w513) -> (x*y=w511:dbl)
                        }
                        n283 = Reverse 1D Array(array=w499) -> (reversed array=w498:dbl[])
                      }
                      frame #1 {
                        n284 = Square(x=w524) -> (x^2=w530:dbl[])
                        n285 = Index Array(array=w525, index #1=2 ("index"), index #2=1 ("index"), index #3=0 ("index"), index #4=4 ("index")) -> (element #1=w519:dbl, element #2=w518:dbl, element #3=w517:dbl, element #4=w529:dbl, element #5=w531:dbl)  [unwired: 1 in]
                        n286 = Multiply(x=w530, y=w524) -> (x*y=w528:dbl[])
                        n287 = Multiply(x=w531, y=w530) -> (x*y=w527:dbl[])
                        n288 = Multiply(x=w529, y=w528) -> (x*y=w526:dbl[])
                        n289 = Add(x=w527, y=w526) -> (x+y=w523:dbl[])
                        n290 = call "rotmrev.vi"("reverse"=TRUE, "angle[rad]"=w519, "x"=w524, "y"=w523, "x0"=w517, "y0"=w518) -> ("y"=w515:dbl[], "x"=w516:dbl[])  [unwired: 4 in]
                      }
                    }
                    n291 = Build Array (concatenate)(w482, w483) -> (w481:dbl[])
                    n292 = Build Array (concatenate)(w479, w480) -> (w478:dbl[])
                  }
                }
              }
              n293 = flat-sequence {
                tunnel: w372 -> [w379]
                tunnel: w373 -> [w376]
                frame #0 {
                  n294 = global read "G_PATH.vi" "xt"() -> (w380:dbl)
                  n295 = global read "G_PATH.vi" "yt"() -> (w377:dbl)
                  n296 = local read "M6006"() -> (w382:T1)
                  n297 = Add(x=w380, y=w379) -> (x+y=w378:dbl[])
                  n298 = Add(x=w377, y=w376) -> (x+y=w375:dbl[])
                  n299 = Unbundle By Name(w382) -> ("lcc[1]"=w386:dbl, "lcc[0]"=w385:dbl, "attitude[2]"=w381:dbl)
                  n300 = Negate(x=w381) -> (-x=w383:dbl)
                  n301 = call "rotm_obs_new.vi"("angle[rad]"=w383, "reverse"=FALSE, "y0"=w385, "x0"=w386, "y"=w375, "x"=w378) -> ("rot*(y-y0) 2"=w389:dbl[], "rot*(x-x0)"=w388:dbl[])  [unwired: 2 in, 2 out]
                  n302 = Build Array(w388, w389) -> (w387:dbl[][])
                  n303 = Transpose 2D Array(2D array=w387) -> (transposed array=w390:dbl[][])
                  n304 = local write "track"(w390) -> ()
                }
              }
            }
          }
        }
        frame #3 {
          n305 = local read "usewpt"() -> (w533:bool)
          n306 = case shown="True" w533 {
            frame False {
              n307 = disable-structure shown="Enabled" {
                frame Enabled {
                  n308 = flat-sequence {
                    frame #0 {
                      "line" <- dbl[][] []
                    }
                    frame #1 {
                      n309 = local read "count"() -> (w541:cluster{dbl[][]}[])
                      n310 = for {
                        tunnel: w541 -> [w607] mode=indexing
                        shift-right: [w604] -> w539
                        shift-left: dbl[][] [] -> [w603]
                        i -> [w605]
                        n311 = Unbundle(w607) -> (w606:dbl[][])
                        n312 = for {
                          tunnel: w606 -> [w617] mode=indexing
                          tunnel: w605 -> [w613]
                          shift-right: [w609] -> w604
                          shift-left: w603 -> [w608]
                          i -> [w612]
                          n313 = Index Array(array=w617, index #1=0 ("index")) -> (element #1=w614:dbl, element #2=w611:dbl)  [unwired: 1 in]
                          n314 = Not Equal To 0?(x=w614) -> (x != 0?=w615:bool)
                          n315 = To Long Integer(number=w611) -> (32bit integer=w610:i32)
                          n316 = case shown="True" w615 {
                            tunnel: w614 -> [_ w633]
                            tunnel: w613 -> [_ w630]
                            tunnel: w612 -> [_ w627]
                            tunnel: w610 -> [_ w623]
                            tunnel: [w618 w620] -> w609
                            tunnel: w608 -> [w618 w619]
                            frame False {
                            }
                            frame True {
                              n317 = local read "idxall"() -> (w631:cluster{i32[]}[])
                              n318 = Index Array(array=w631, index #1=w630) -> (element #1=w629:cluster{i32[]}, element #2=w625:cluster{i32[]})  [unwired: 1 in]
                              n319 = Unbundle(w629) -> (w628:i32[])
                              n320 = Unbundle(w625) -> (w624:i32[])
                              n321 = Index Array(array=w628, index=w627) -> (element=w626:i32)
                              n322 = Index Array(array=w624, index=w623) -> (element=w622:i32)
                              n323 = Build Array(w633, 0.0 ("element"), w626, w622) -> (w621:dbl[])
                              n324 = Build Array (concatenate)(w619, w621) -> (w620:dbl[][])
                            }
                          }
                        }
                      }
                      n325 = Array Size(array=w539) -> (size(s)=w538:i32[])
                      n326 = Index Array(array=w538, index=0) -> (element=w536:i32)
                      n327 = for {
                        N: w536 -> [_]
                        shift-right: [w546] -> w535
                        shift-left: w539 -> [w545]
                        i -> [w544]
                        n328 = Index Array(array=w545, index (row)=w544, index (col)=0) -> (element=w542:dbl)
                        n329 = Greater Than 0?(x=w542) -> (x > 0?=w547:bool)
                        n330 = case shown="True" w547 {
                          tunnel: w545 -> [w548 w552]
                          tunnel: w544 -> [_ w550]
                          tunnel: [w548 w549] -> w546
                          frame False {
                          }
                          frame True {
                            n331 = while {
                              shift-right: [w556] -> w549
                              shift-left: w552 -> [w555]
                              shift-right: [w559] -> _
                              shift-left: 3 -> [w560]
                              tunnel: w550 -> [w554]
                              stop <- w562 continue-if-true
                              n332 = Index Array(array=w555, index (row)=w554) -> (element=w553:dbl[])  [unwired: 1 in]
                              n333 = Index Array(array=w555, index (col)=2 ("disabled index (col)")) -> (element=w564:dbl[])  [unwired: 1 in]
                              n334 = Index Array(array=w553, index #1=w560, index #2=0 ("index")) -> (element #1=w565:dbl, element #2=w557:dbl)
                              n335 = Equal?(x=w565, y=w564) -> (x = y?=w561:bool[])
                              n336 = Or Array Elements(Boolean array=w561) -> (logical OR=w563:bool)
                              n337 = case shown="True" w563 {
                                tunnel: [_ TRUE] -> w562
                                tunnel: w561 -> [_ w593]
                                tunnel: w560 -> [w568 w591]
                                tunnel: [3 w573] -> w559
                                tunnel: w555 -> [w571 w577]
                                tunnel: w554 -> [w570 w588]
                                tunnel: w557 -> [_ w584]
                                tunnel: [w567 w579] -> w556
                                frame False {
                                n338 = Replace Array Subset(array=w571, new element=w568, index (row)=w570, index (col)=1 ("disabled index (col)")) -> (w567:dbl[][])
                                }
                                frame True {
                                n339 = Boolean To (0,1)(Boolean=w593) -> (0, 1=w592:i16[])
                                n340 = Increment(x=w591) -> (x+1=w573:i32)
                                n341 = Array Max & Min(array=w592) -> (max index (indices)=w582:i32)  [unwired: 3 out]
                                n342 = Index Array(array=w577, index (row)=w582) -> (element=w578:dbl[])  [unwired: 1 in]
                                n343 = Array Size(array=w578) -> (size(s)=w575:i32)
                                n344 = Index Array(array=w578, index #1=3 ("index"), index #2=0 ("index")) -> (element #1=w589:dbl, element #2=w585:dbl)
                                n345 = Less Or Equal?(x=w575, y=w573) -> (x <= y?=w574:bool)
                                n346 = Add(x=w585, y=w584) -> (x+y=w583:dbl)
                                n347 = case shown="True" w574 {
                                tunnel: w577 -> [w595 w600]
                                tunnel: [w595 w601] -> w576
                                tunnel: w573 -> [_ w602]
                                frame False {
                                }
                                frame True {
                                n348 = Index Array(array=w600, index (col)=1 ("disabled index (col)")) -> (element=w598:dbl[])  [unwired: 1 in]
                                n349 = Multiply(x=w598, y=0) -> (x*y=w596:dbl[])
                                n350 = Insert Into Array(array=w600, index (col)=w602, new element=w596) -> (w601:dbl[][])  [unwired: 1 in]
                                }
                                }
                                n351 = Replace Array Subset(array=w576, new element #1=w589, index (row) #1=w588, index (col) #1=w573, new element #2=w583, index (row) #2=w588, index (col) #2=0 ("disabled index (col)"), new element #3=0.0 ("new element/subarray"), index (row) #3=w582, index (col) #3=0 ("disabled index (col)")) -> (w579:dbl[][])
                                }
                              }
                            }
                          }
                        }
                      }
                      n352 = local write "line"(w535) -> ()
                    }
                  }
                }
                frame Disabled {
                }
              }
            }
            frame True {
              n353 = flat-sequence {
                frame #0 {
                  n354 = local read "track"() -> (w658:dbl[][])
                  n355 = Index Array(array=w658, index (col)=0 ("disabled index (col)")) -> (element=w681:dbl[])  [unwired: 1 in]
                  n356 = Index Array(array=w658, index (col)=1 ("disabled index (col)")) -> (element=w670:dbl[])  [unwired: 1 in]
                  n357 = Rotate 1D Array(1:w681, 2:1 ("n")) -> (0:w680:dbl[])
                  n358 = Rotate 1D Array(1:w670, 2:1 ("n")) -> (0:w671:dbl[])
                  n359 = Subtract(x=w681, y=w680) -> (x-y=w679:dbl[])
                  n360 = Subtract(x=w670, y=w671) -> (x-y=w672:dbl[])
                  n361 = Replace Array Subset(array=w679, new element=0.0 ("new element/subarray"), index=0) -> (w676:dbl[])
                  n362 = Replace Array Subset(array=w672, new element=0.0 ("new element/subarray"), index=0) -> (w675:dbl[])
                  n363 = Square(x=w676) -> (x^2=w667:dbl[])
                  n364 = Square(x=w675) -> (x^2=w666:dbl[])
                  n365 = Add(x=w667, y=w666) -> (x+y=w665:dbl[])
                  n366 = Square Root(x=w665) -> (sqrt(x)=w664:dbl[])
                  n367 = for {
                    tunnel: w664 -> [w688] mode=indexing
                    shift-right: [w686] -> _
                    shift-left: 0.0 -> [w687]
                    tunnel: [w686] -> w662 mode=indexing
                    n368 = Add(x=w687, y=w688) -> (x+y=w686:dbl)
                  }
                  n369 = local read "ymax"() -> (w657:dbl)
                  n370 = Threshold 1D Array(2:w657, 3:w662) -> (0:w661:dbl)  [unwired: 1 in]
                  n371 = Round Toward +Infinity(x=w661) -> (ceil(x): smallest int >= x=w660:dbl)
                  n372 = To Long Integer(number=w660) -> (32bit integer=w684:i32)
                  n373 = Array Subset(array=w658, index (row)=0 ("index"), length (row)=w684) -> (→"map_track":dbl[][])  [unwired: 2 in]
                }
                frame #1 {
                  w704 = 3 ("disabled index (col)")
                  n374 = local read "map_track"() -> (w696:dbl[][])
                  n375 = Array Size(array=w696) -> (size(s)=w694:i32[])
                  n376 = Index Array(array=w694) -> (element=w693:i32)  [unwired: 1 in]
                  n377 = Multiply(x=w693, y=0.8) -> (x*y=w691:dbl)
                  n378 = Round Toward +Infinity(x=w691) -> (ceil(x): smallest int >= x=w690:dbl)
                  n379 = Array Subset(array=w696, length (row)=w690) -> (w695:dbl[][])  [unwired: 3 in]
                  n380 = Empty Array?(array=w695) -> (empty?=w698:bool)
                  n381 = Index Array(array=w695, index (col) #1=0 ("disabled index (col)")) -> (element #1=w713:dbl[], element #2=w712:dbl[])  [unwired: 3 in]
                  n382 = Square(x=w713) -> (x^2=w711:dbl[])
                  n383 = Square(x=w712) -> (x^2=w710:dbl[])
                  n384 = Multiply(x=w712, y=0.0) -> (x*y=w715:dbl[])
                  n385 = Multiply(x=-2.0, y=w713) -> (x*y=w718:dbl[])
                  n386 = Add(x=w711, y=w710) -> (x+y=w709:dbl[])
                  n387 = Increment(x=w715) -> (x+1=w714:dbl[])
                  n388 = Multiply(x=w712, y=-2.0) -> (x*y=w717:dbl[])
                  n389 = Build Array(w718, w717, w714, w709) -> (w708:dbl[][])
                  n390 = Transpose 2D Array(2D array=w708) -> (transposed array=w707:dbl[][])
                  n391 = call-poly <vilib>:"Array To Matrix.vi"("Real 2D Array"=w707) -> ("Real Matrix"=w706:T5)
                  n392 = call-poly <vilib>:"SVD Decomposition.vi"("A"=w706) -> ("Matrix V"=w705:T5)  [unwired: 6 in, 4 out]
                  n393 = Index Array(array=w705, index (col) #1=w704, index (row) #2=w704, index (col) #2=w704) -> (element #1=w703:dbl[], element #2=w702:dbl)  [unwired: 1 in]
                  n394 = Divide(x=w703, y=w702) -> (x/y=w701:dbl[])
                  n395 = Not A Number/Path/Refnum?(number/path/refnum=w701) -> (NaN/Path/Refnum?=w700:bool[])
                  n396 = Or Array Elements(Boolean array=w700) -> (logical OR=w699:bool)
                  n397 = Or(x=w698, y=w699) -> (x .or. y?=w697:bool)
                  n398 = case shown="False" w697 {
                    tunnel: [w731 w742] -> w722
                    tunnel: w701 -> [w727 _]
                    frame False {
                      n399 = Index Array(array=w727, index #1=0 ("index"), index #4=0 ("index")) -> (element #1=w740:dbl, element #2=w739:dbl, element #3=w732:dbl, element #4=w729:dbl, element #5=w728:dbl)  [unwired: 3 in]
                      n400 = Square(x=w740) -> (x^2=w738:dbl)
                      n401 = Square(x=w739) -> (x^2=w737:dbl)
                      n402 = Add(x=w738, y=w737) -> (x+y=w733:dbl)
                      n403 = Subtract(x=w733, y=w732) -> (x-y=w735:dbl)
                      n404 = Absolute Value(x=w735) -> (abs(x)=w736:dbl)
                      n405 = Square Root(x=w736) -> (sqrt(x)=w734:dbl)
                      n406 = Build Array(w734, w729, w728) -> (w731:dbl[])
                    }
                    frame True {
                      w744 = 0.0 ("element")
                      n407 = Build Array(inf, w744, w744) -> (w742:dbl[])
                    }
                  }
                  n408 = Index Array(array=w722, index=0) -> (element=w725:dbl)
                  n409 = Greater?(x=w725, y=10000.0) -> (0:w723:bool)
                  n410 = case shown="True" w723 {
                    tunnel: [w745 w751] -> w689
                    tunnel: w722 -> [w745 w754]
                    frame False {
                    }
                    frame True {
                      w746 = 0.0 ("element")
                      n411 = Index Array(array=w754, index=0) -> (element=w752:dbl)
                      n412 = local read "map_track"() -> (w758:dbl[][])
                      n413 = Index Array(array=w758, index (col)=0 ("disabled index (col)")) -> (element=w756:dbl[])  [unwired: 1 in]
                      n414 = Add Array Elements(numeric array=w756) -> (sum=w755:dbl)
                      n415 = Array Size(array=w756) -> (size(s)=w750:i32)
                      n416 = Divide(x=w755, y=w750) -> (x/y=w748:dbl)
                      n417 = Not Equal To 0?(x=w750) -> (x != 0?=w749:bool)
                      n418 = Select(t=w748, s=w749, f=w746) -> (s? t:f=w747:dbl)
                      n419 = Build Array(w752, w747, w746) -> (w751:dbl[])
                    }
                  }
                  "RXY" <- w689
                  n420 = global write "G_PATH.vi" "RXY"(w689) -> ()
                }
              }
              n421 = local read "track"() -> (w647:dbl[][])
              n422 = Array Size(array=w647) -> (size(s)=w652:i32[])
              n423 = Index Array(array=w652, index=0) -> (element=w650:i32)
              n424 = Decrement(x=w650) -> (x-1=w649:i32)
              n425 = Array Subset(array=w647, index (row)=0 ("index"), length (row)=w649) -> (w645:dbl[][])  [unwired: 2 in]
              n426 = Array Subset(array=w647, index (row)=1 ("index")) -> (w646:dbl[][])  [unwired: 3 in]
              n427 = Subtract(x=w646, y=w645) -> (x-y=w644:dbl[][])
              n428 = Square(x=w644) -> (x^2=w643:dbl[][])
              n429 = Index Array(array=w643, index (col) #1=0 ("disabled index (col)")) -> (element #1=w641:dbl[], element #2=w640:dbl[])  [unwired: 3 in]
              n430 = Add(x=w641, y=w640) -> (x+y=w639:dbl[])
              n431 = Square Root(x=w639) -> (sqrt(x)=w638:dbl[])
              n432 = Build Array (concatenate)(0.0, w638) -> (w636:dbl[])
              n433 = for {
                tunnel: w636 -> [w761] mode=indexing
                shift-right: [w759] -> _
                shift-left: 0.0 -> [w760]
                tunnel: [w759] -> w634 mode=indexing
                n434 = Add(x=w761, y=w760) -> (x+y=w759:dbl)
              }
              n435 = local read "xseed"() -> (w656:dbl[])
              n436 = for {
                tunnel: w656 -> [w771] mode=indexing
                shift-right: [w765] -> w654
                shift-left: i32[] [] -> [w764]
                tunnel: w634 -> [w763]
                n437 = Subtract(x=w771, y=w763) -> (x-y=w770:dbl[])
                n438 = Absolute Value(x=w770) -> (abs(x)=w762:dbl[])
                n439 = Array Max & Min(array=w762) -> (min value=w769:dbl, min index (indices)=w766:i32)  [unwired: 2 out]
                n440 = Less?(x=w769, y=1.0) -> (x < y?=w767:bool)
                n441 = case shown="False" w767 {
                  tunnel: w766 -> [_ w775]
                  tunnel: [w772 w774] -> w765
                  tunnel: w764 -> [w772 w773]
                  frame False {
                  }
                  frame True {
                    n442 = Build Array (concatenate)(w773, w775) -> (w774:i32[])
                  }
                }
              }
              "mapidx" <- w654
            }
          }
        }
        frame #4 {
          n443 = flat-sequence {
            frame #0 {
              w777 = dbl[] [] ("x")
              w779 = 0.0
              "mode" <- w779
              "a" <- w779
              "b" <- w779
              "rd0" <- w779
              "fitting?" <- FALSE ("fitting?")
              "x" <- w777
              "y" <- w777
              "abrd0" <- dbl[][] []
            }
            frame #1 {
              n444 = local read "usewpt"() -> (w780:bool)
              n445 = case shown="False" w780 {
                frame False {
                  n446 = disable-structure shown="Enabled" {
                    frame Enabled {
                      n447 = flat-sequence {
                        tunnel: [w784] -> w782
                        tunnel: [w783] -> w781
                        tunnel: w782 -> [w793]
                        tunnel: w781 -> [w792]
                        frame #0 {
                          n448 = local read "line"() -> (w784:dbl[][])
                          n449 = disable-structure shown="Enabled" {
                            disable-tunnel: w784 -> [w786 _]
                            disable-tunnel: [w785 i16 1 ("element")] -> w783
                            frame Enabled {
                              n450 = Index Array(array=w786, index (col)=0 ("disabled index (col)")) -> (element=w789:dbl[])  [unwired: 1 in]
                              n451 = Not Equal To 0?(x=w789) -> (x != 0?=w788:bool[])
                              n452 = Boolean To (0,1)(Boolean=w788) -> (0, 1=w787:i16[])
                              n453 = Add Array Elements(numeric array=w787) -> (sum=w785:i16)
                            }
                            frame Disabled {
                            }
                          }
                        }
                        frame #1 {
                          n454 = for {
                            N: w792 -> [_]
                            shift-right: [w794] -> _
                            shift-left: w793 -> [w796]
                            n455 = Index Array(array=w796, index (col)=0 ("disabled index (col)")) -> (element=w811:dbl[])  [unwired: 1 in]
                            n456 = Array Max & Min(array=w811) -> (max value=w804:dbl, max index (indices)=w795:i32)  [unwired: 2 out]
                            n457 = Index Array(array=w796, index (row)=w795) -> (element=w809:dbl[])  [unwired: 1 in]
                            n458 = Not Equal To 0?(x=w804) -> (x != 0?=w802:bool)
                            n459 = Replace Array Subset(array=w796, new element=0.0 ("new element/subarray"), index (row)=w795, index (col)=0 ("disabled index (col)")) -> (w794:dbl[][])
                            n460 = Index Array(array=w809, index=1) -> (element=w800:dbl)
                            n461 = Decrement(x=w800) -> (x-1=w799:dbl)
                            n462 = Array Subset(array=w809, index=2, length=w799) -> (w807:dbl[])
                            n463 = Array Size(array=w807) -> (size(s)=w806:i32)
                            n464 = Greater Or Equal?(x=w806, y=3) -> (x >= y?=w803:bool)
                            n465 = And(x=w803, y=w802) -> (x .and. y?=w801:bool)
                            n466 = case shown="True" w801 {
                              tunnel: w807 -> [_ w815]
                              frame False {
                              }
                              frame True {
                                n467 = To Long Integer(number=w815) -> (32bit integer=w814:i32[])
                                n468 = flat-sequence {
                                tunnel: w814 -> [w819]
                                tunnel: [w819] -> w813
                                tunnel: w813 -> [w830]
                                frame #0 {
                                w818 = 0.0
                                n469 = for {
                                tunnel: w819 -> [w824] mode=indexing
                                tunnel: [w821] -> w817 mode=indexing
                                tunnel: [w820] -> w816 mode=indexing
                                n470 = local read "data"() -> (w825:dbl[][])
                                n471 = Index Array(array=w825, index (row)=w824) -> (element=w823:dbl[])  [unwired: 1 in]
                                n472 = Index Array(array=w823, index #1=0 ("index")) -> (element #1=w821:dbl, element #2=w820:dbl)  [unwired: 1 in]
                                }
                                n473 = local write "a"(w818) -> ()
                                n474 = local write "b"(w818) -> ()
                                n475 = local write "rd0"(w818) -> ()
                                n476 = local write "x"(w817) -> ()
                                n477 = local write "y"(w816) -> ()
                                }
                                frame #1 {
                                n478 = Array Size(array=w830) -> (size(s)=w827:i32)
                                n479 = Subtract(x=w827, y=2) -> (x-y=w828:i32)
                                n480 = for {
                                N: w828 -> [_]
                                tunnel: w827 -> [w916]
                                tunnel: [w915] -> w826
                                i -> [w917]
                                stop <- w915 stop-if-true
                                n481 = Decrement(x=w916) -> (x-1=w920:i32)
                                n482 = Increment(x=w917) -> (x+1=w919:i32)
                                n483 = Subtract(x=w920, y=w919) -> (x-y=w918:i32)
                                n484 = for {
                                N: w918 -> [_]
                                tunnel: w919 -> [w927]
                                tunnel: w917 -> [w923]
                                tunnel: w916 -> [w922]
                                tunnel: [w921] -> w915
                                i -> [w928]
                                stop <- w921 stop-if-true
                                n485 = Add(x=w927, y=w928) -> (x+y=w924:i32)
                                n486 = Increment(x=w924) -> (x+1=w925:i32)
                                n487 = Subtract(x=w922, y=w925) -> (x-y=w926:i32)
                                n488 = for {
                                N: w926 -> [_]
                                tunnel: w925 -> [w937]
                                tunnel: w924 -> [w934]
                                tunnel: w923 -> [w933]
                                tunnel: [w929] -> w921
                                i -> [w936]
                                stop <- w929 stop-if-true
                                n489 = Add(x=w937, y=w936) -> (x+y=w935:i32)
                                n490 = flat-sequence {
                                tunnel: w935 -> [w940]
                                tunnel: w934 -> [w939]
                                tunnel: w933 -> [w938]
                                tunnel: [w941] -> w931
                                tunnel: [w982] -> w932
                                tunnel: w931 -> [w981]
                                tunnel: [w981] -> w930
                                tunnel: w932 -> [w1034]
                                tunnel: w930 -> [w1030]
                                tunnel: [w1022] -> w929
                                frame #0 {
                                "k" <- w940
                                "j" <- w939
                                "i" <- w938
                                }
                                frame #1 {
                                n491 = local read "y"() -> (w977:dbl[])
                                n492 = local read "j"() -> (w978:i32)
                                n493 = local read "k"() -> (w976:i32)
                                n494 = local read "y"() -> (w970:dbl[])
                                n495 = local read "k"() -> (w969:i32)
                                n496 = local read "i"() -> (w971:i32)
                                n497 = local read "x"() -> (w966:dbl[])
                                n498 = local read "k"() -> (w965:i32)
                                n499 = local read "y"() -> (w963:dbl[])
                                n500 = local read "i"() -> (w964:i32)
                                n501 = local read "j"() -> (w962:i32)
                                n502 = local read "x"() -> (w980:dbl[])
                                n503 = local read "i"() -> (w979:i32)
                                n504 = local read "x"() -> (w967:dbl[])
                                n505 = local read "j"() -> (w968:i32)
                                n506 = Index Array(array=w977, index #1=w978, index #2=w976) -> (element #1=w975:dbl, element #2=w974:dbl)
                                n507 = Index Array(array=w970, index #1=w969, index #2=w971) -> (element #1=w972:dbl, element #2=w973:dbl)
                                n508 = Index Array(array=w966, index=w965) -> (element=w949:dbl)
                                n509 = Index Array(array=w963, index #1=w964, index #2=w962) -> (element #1=w961:dbl, element #2=w960:dbl)
                                n510 = Index Array(array=w980, index=w979) -> (element=w955:dbl)
                                n511 = Index Array(array=w967, index=w968) -> (element=w952:dbl)
                                n512 = Subtract(x=w975, y=w974) -> (x-y=w959:dbl)
                                n513 = Subtract(x=w972, y=w973) -> (x-y=w958:dbl)
                                n514 = Subtract(x=w961, y=w960) -> (x-y=w957:dbl)
                                n515 = Multiply(x=w955, y=w959) -> (x*y=w956:dbl)
                                n516 = Multiply(x=w952, y=w958) -> (x*y=w953:dbl)
                                n517 = Multiply(x=w949, y=w957) -> (x*y=w950:dbl)
                                n518 = Compound Arithmetic op=MULTIPLY(w959, w958, w957) -> (w945:dbl)
                                n519 = Multiply(x=w955, y=w956) -> (x*y=w954:dbl)
                                n520 = Multiply(x=w952, y=w953) -> (x*y=w951:dbl)
                                n521 = Multiply(x=w949, y=w950) -> (x*y=w948:dbl)
                                n522 = Compound Arithmetic op=ADD(w956, w953, w950) -> (w941:dbl)
                                n523 = Compound Arithmetic op=ADD(w954, w951, w948) -> (w946:dbl)
                                n524 = Subtract(x=w946, y=w945) -> (x-y=w944:dbl)
                                n525 = Divide(x=w944, y=w941) -> (x/y=w943:dbl)
                                n526 = local read "a"() -> (w947:dbl)
                                n527 = Add(x=w947, y=w943) -> (x+y=w942:dbl)
                                n528 = local write "a"(w942) -> ()
                                }
                                frame #2 {
                                n529 = local read "x"() -> (w1000:dbl[])
                                n530 = local read "i"() -> (w999:i32)
                                n531 = local read "j"() -> (w1001:i32)
                                n532 = local read "y"() -> (w983:dbl[])
                                n533 = local read "i"() -> (w984:i32)
                                n534 = local read "x"() -> (w986:dbl[])
                                n535 = local read "j"() -> (w985:i32)
                                n536 = local read "k"() -> (w987:i32)
                                n537 = local read "y"() -> (w996:dbl[])
                                n538 = local read "j"() -> (w995:i32)
                                n539 = local read "x"() -> (w993:dbl[])
                                n540 = local read "k"() -> (w994:i32)
                                n541 = local read "i"() -> (w992:i32)
                                n542 = local read "y"() -> (w997:dbl[])
                                n543 = local read "k"() -> (w998:i32)
                                n544 = Index Array(array=w1000, index #1=w999, index #2=w1001) -> (element #1=w1002:dbl, element #2=w1003:dbl)
                                n545 = Index Array(array=w983, index=w984) -> (element=w1008:dbl)
                                n546 = Index Array(array=w986, index #1=w985, index #2=w987) -> (element #1=w988:dbl, element #2=w989:dbl)
                                n547 = Index Array(array=w996, index=w995) -> (element=w1011:dbl)
                                n548 = Index Array(array=w993, index #1=w994, index #2=w992) -> (element #1=w991:dbl, element #2=w990:dbl)
                                n549 = Index Array(array=w997, index=w998) -> (element=w1014:dbl)
                                n550 = Subtract(x=w1002, y=w1003) -> (x-y=w1006:dbl)
                                n551 = Subtract(x=w988, y=w989) -> (x-y=w1004:dbl)
                                n552 = Subtract(x=w991, y=w990) -> (x-y=w1005:dbl)
                                n553 = Compound Arithmetic op=MULTIPLY(w1004, w1005, w1006) -> (w1018:dbl)
                                n554 = Multiply(x=w1008, y=w1004) -> (x*y=w1007:dbl)
                                n555 = Multiply(x=w1014, y=w1006) -> (x*y=w1013:dbl)
                                n556 = Multiply(x=w1011, y=w1005) -> (x*y=w1010:dbl)
                                n557 = Multiply(x=w1008, y=w1007) -> (x*y=w1009:dbl)
                                n558 = Multiply(x=w1011, y=w1010) -> (x*y=w1012:dbl)
                                n559 = Multiply(x=w1014, y=w1013) -> (x*y=w1015:dbl)
                                n560 = Compound Arithmetic op=ADD(w1007, w1010, w1013) -> (w982:dbl)
                                n561 = Compound Arithmetic op=ADD(w1009, w1012, w1015) -> (w1017:dbl)
                                n562 = Subtract(x=w1017, y=w1018) -> (x-y=w1019:dbl)
                                n563 = Divide(x=w1019, y=w982) -> (x/y=w1020:dbl)
                                n564 = local read "b"() -> (w1016:dbl)
                                n565 = Add(x=w1016, y=w1020) -> (x+y=w1021:dbl)
                                n566 = local write "b"(w1021) -> ()
                                }
                                frame #3 {
                                n567 = Multiply(x=w1034, y=w1030) -> (x*y=w1038:dbl)
                                n568 = Absolute Value(x=w1030) -> (abs(x)=w1032:dbl)
                                n569 = Absolute Value(x=w1034) -> (abs(x)=w1036:dbl)
                                n570 = Sign(1:w1038) -> (0:w1037:dbl)
                                n571 = Greater?(x=w1032, y=1e-12) -> (0:w1029:bool)
                                n572 = Greater?(x=w1036, y=1e-12) -> (0:w1033:bool)
                                n573 = Absolute Value(x=w1037) -> (abs(x)=w1028:dbl)
                                n574 = Boolean To (0,1)(Boolean=w1029) -> (0, 1=w1025:i16)
                                n575 = Boolean To (0,1)(Boolean=w1033) -> (0, 1=w1027:i16)
                                n576 = To Double Precision Float(number=w1027) -> (double precision float=w1026:dbl)
                                n577 = To Double Precision Float(number=w1025) -> (double precision float=w1024:dbl)
                                n578 = Compound Arithmetic op=MULTIPLY(w1026, w1028, w1024) -> (w1023:dbl)
                                n579 = Equal To 0?(x=w1023) -> (x = 0?=w1022:bool)
                                }
                                }
                                }
                                }
                                }
                                n580 = case shown="False" w826 {
                                frame False {
                                n581 = flat-sequence {
                                frame #0 {
                                n582 = local read "x"() -> (w853:dbl[])
                                n583 = Array Size(array=w853) -> (size(s)=w850:i32)
                                n584 = Subtract(x=w850, y=3) -> (x-y=w848:i32)
                                n585 = for {
                                N: w850 -> [_]
                                shift-right: [w859] -> w845
                                shift-left: 1 -> [w858]
                                i -> [w861]
                                n586 = Increment(x=w861) -> (x+1=w860:i32)
                                n587 = Multiply(x=w858, y=w860) -> (x*y=w859:i32)
                                }
                                n588 = for {
                                N: w848 -> [_]
                                shift-right: [w855] -> w847
                                shift-left: 1 -> [w854]
                                i -> [w857]
                                n589 = Increment(x=w857) -> (x+1=w856:i32)
                                n590 = Multiply(x=w854, y=w856) -> (x*y=w855:i32)
                                }
                                n591 = To Double Precision Float(number=w845) -> (double precision float=w842:dbl)
                                n592 = Multiply(x=w847, y=6) -> (x*y=w844:i32)
                                n593 = To Double Precision Float(number=w844) -> (double precision float=w843:dbl)
                                n594 = Divide(x=w842, y=w843) -> (x/y=w841:dbl)
                                n595 = Multiply(x=2.0, y=w841) -> (x*y=w837:dbl)
                                n596 = local read "a"() -> (w839:dbl)
                                n597 = local read "b"() -> (w838:dbl)
                                n598 = Divide(x=w839, y=w837) -> (x/y=w836:dbl)
                                n599 = Divide(x=w838, y=w837) -> (x/y=w835:dbl)
                                n600 = local write "a"(w836) -> ()
                                n601 = local write "b"(w835) -> ()
                                n602 = Square(x=w836) -> (x^2=w833:dbl)
                                n603 = Square(x=w835) -> (x^2=w834:dbl)
                                n604 = Add(x=w833, y=w834) -> (x+y=w832:dbl)
                                n605 = Square Root(x=w832) -> (sqrt(x)=w831:dbl)
                                n606 = local write "rd0"(w831) -> ()
                                }
                                frame #1 {
                                n607 = local read "y"() -> (w867:dbl[])
                                n608 = local read "x"() -> (w876:dbl[])
                                n609 = local read "a"() -> (w875:dbl)
                                n610 = local read "b"() -> (w874:dbl)
                                n611 = Array Size(array=w867) -> (size(s)=w865:i32)
                                n612 = Subtract(x=w876, y=w875) -> (x-y=w873:dbl[])
                                n613 = Subtract(x=w867, y=w874) -> (x-y=w872:dbl[])
                                n614 = Square(x=w873) -> (x^2=w871:dbl[])
                                n615 = Square(x=w872) -> (x^2=w870:dbl[])
                                n616 = Add(x=w871, y=w870) -> (x+y=w869:dbl[])
                                n617 = Square Root(x=w869) -> (sqrt(x)=w868:dbl[])
                                n618 = Add Array Elements(numeric array=w868) -> (sum=w866:dbl)
                                n619 = Divide(x=w866, y=w865) -> (x/y=w864:dbl)
                                n620 = Greater?(x=w864, y=300.0) -> (0:w862:bool)
                                n621 = case shown="True" w862 {
                                frame False {
                                }
                                frame True {
                                w877 = 0.0 ("rd0")
                                n622 = local read "x"() -> (w886:dbl[])
                                n623 = local read "y"() -> (w890:dbl[])
                                n624 = local write "b"(w877) -> ()
                                n625 = local write "rd0"(w877) -> ()
                                n626 = local write "mode"(w877) -> ()
                                n627 = local read "y"() -> (w887:dbl[])
                                n628 = Array Size(array=w886) -> (size(s)=w894:i32)
                                n629 = Square(x=w886) -> (x^2=w895:dbl[])
                                n630 = Add Array Elements(numeric array=w886) -> (sum=w888:dbl)
                                n631 = Add Array Elements(numeric array=w890) -> (sum=w889:dbl)
                                n632 = Multiply(x=w886, y=w887) -> (x*y=w884:dbl[])
                                n633 = Multiply(x=w889, y=w888) -> (x*y=w882:dbl)
                                n634 = Add Array Elements(numeric array=w895) -> (sum=w893:dbl)
                                n635 = To Double Precision Float(number=w894) -> (double precision float=w885:dbl)
                                n636 = Square(x=w888) -> (x^2=w891:dbl)
                                n637 = Add Array Elements(numeric array=w884) -> (sum=w883:dbl)
                                n638 = Multiply(x=w893, y=w885) -> (x*y=w892:dbl)
                                n639 = Multiply(x=w885, y=w883) -> (x*y=w881:dbl)
                                n640 = Subtract(x=w891, y=w892) -> (x-y=w879:dbl)
                                n641 = Subtract(x=w882, y=w881) -> (x-y=w880:dbl)
                                n642 = Divide(x=w880, y=w879) -> (x/y=w878:dbl)
                                n643 = local write "a"(w878) -> ()
                                }
                                }
                                }
                                }
                                }
                                frame True {
                                w896 = 0.0 ("rd0")
                                n644 = local read "x"() -> (w905:dbl[])
                                n645 = local read "y"() -> (w909:dbl[])
                                n646 = local write "b"(w896) -> ()
                                n647 = local write "rd0"(w896) -> ()
                                n648 = local read "y"() -> (w906:dbl[])
                                n649 = Array Size(array=w905) -> (size(s)=w913:i32)
                                n650 = Square(x=w905) -> (x^2=w914:dbl[])
                                n651 = Add Array Elements(numeric array=w905) -> (sum=w907:dbl)
                                n652 = Add Array Elements(numeric array=w909) -> (sum=w908:dbl)
                                n653 = Multiply(x=w905, y=w906) -> (x*y=w903:dbl[])
                                n654 = Multiply(x=w908, y=w907) -> (x*y=w901:dbl)
                                n655 = Add Array Elements(numeric array=w914) -> (sum=w912:dbl)
                                n656 = To Double Precision Float(number=w913) -> (double precision float=w904:dbl)
                                n657 = Add Array Elements(numeric array=w903) -> (sum=w902:dbl)
                                n658 = Multiply(x=w912, y=w904) -> (x*y=w911:dbl)
                                n659 = Square(x=w907) -> (x^2=w910:dbl)
                                n660 = Multiply(x=w904, y=w902) -> (x*y=w900:dbl)
                                n661 = Subtract(x=w910, y=w911) -> (x-y=w898:dbl)
                                n662 = Subtract(x=w901, y=w900) -> (x-y=w899:dbl)
                                n663 = Divide(x=w899, y=w898) -> (x/y=w897:dbl)
                                n664 = local write "a"(w897) -> ()
                                }
                                }
                                }
                                frame #2 {
                                n665 = local read "rd0"() -> (w1042:dbl)
                                n666 = local read "a"() -> (w1044:dbl)
                                n667 = local read "b"() -> (w1043:dbl)
                                n668 = Build Array(w1044, w1043, w1042) -> (w1040:dbl[])
                                n669 = local read "abrd0"() -> (w1041:dbl[][])
                                n670 = Build Array (concatenate)(w1041, w1040) -> (w1039:dbl[][])
                                n671 = local write "abrd0"(w1039) -> ()
                                }
                                }
                              }
                            }
                          }
                        }
                        frame #2 {
                          n672 = local read "abrd0"() -> (w1047:dbl[][])
                          n673 = Empty Array?(array=w1047) -> (empty?=w1046:bool)
                          n674 = Not(x=w1046) -> (.not. x?=w1045:bool)
                          n675 = local write "fitting?"(w1045) -> ()
                          n676 = case shown="True" w1045 {
                            tunnel: w1047 -> [_ w1048]
                            frame False {
                            }
                            frame True {
                              n677 = Index Array(array=w1048, index (col)=2 ("disabled index (col)")) -> (element=w1056:dbl[])  [unwired: 1 in]
                              n678 = Equal To 0?(x=w1056) -> (x = 0?=w1055:bool[])
                              n679 = Index Array(array=w1056, index=0) -> (element=w1057:dbl)
                              n680 = Boolean To (0,1)(Boolean=w1055) -> (0, 1=w1054:i16[])
                              n681 = Equal To 0?(x=w1057) -> (x = 0?=w1050:bool)
                              n682 = Add Array Elements(numeric array=w1054) -> (sum=w1053:i16)
                              n683 = Greater?(x=w1053, y=i16 2) -> (0:w1051:bool)
                              n684 = Or(x=w1051, y=w1050) -> (x .or. y?=w1049:bool)
                              n685 = case shown="False" w1049 {
                                frame False {
                                n686 = local read "abrd0"() -> (w1096:dbl[][])
                                n687 = local write "mode"(1.0 ("mode")) -> ()
                                n688 = local read "maxradius"() -> (w1061:dbl)
                                n689 = Index Array(array=w1096, index (col) #1=0 ("disabled index (col)"), index (col) #4=0 ("disabled index (col)")) -> (element #1=w1076:dbl[], element #2=w1071:dbl[], element #3=w1081:dbl[], element #4=w1092:dbl[], element #5=w1087:dbl[])  [unwired: 8 in]
                                n690 = Not Equal To 0?(x=w1081) -> (x != 0?=w1079:bool[])
                                n691 = Index Array(array=w1092, index=0) -> (element=w1093:dbl)
                                n692 = Index Array(array=w1087, index=0) -> (element=w1089:dbl)
                                n693 = Subtract(x=w1092, y=w1093) -> (x-y=w1091:dbl[])
                                n694 = Subtract(x=w1087, y=w1089) -> (x-y=w1090:dbl[])
                                n695 = Square(x=w1091) -> (x^2=w1086:dbl[])
                                n696 = Square(x=w1090) -> (x^2=w1085:dbl[])
                                n697 = Add(x=w1086, y=w1085) -> (x+y=w1084:dbl[])
                                n698 = Square Root(x=w1084) -> (sqrt(x)=w1083:dbl[])
                                n699 = Less?(x=w1083, y=25.0) -> (x < y?=w1080:bool[])
                                n700 = And(x=w1079, y=w1080) -> (x .and. y?=w1078:bool[])
                                n701 = Boolean To (0,1)(Boolean=w1078) -> (0, 1=w1070:i16[])
                                n702 = Multiply(x=w1076, y=w1070) -> (x*y=w1075:dbl[])
                                n703 = Multiply(x=w1071, y=w1070) -> (x*y=w1072:dbl[])
                                n704 = Add Array Elements(numeric array=w1070) -> (sum=w1069:i16)
                                n705 = Add Array Elements(numeric array=w1075) -> (sum=w1074:dbl)
                                n706 = Add Array Elements(numeric array=w1072) -> (sum=w1073:dbl)
                                n707 = Divide(x=w1074, y=w1069) -> (x/y=w1068:dbl)
                                n708 = Divide(x=w1073, y=w1069) -> (x/y=w1067:dbl)
                                n709 = local write "a"(w1068) -> ()
                                n710 = local write "b"(w1067) -> ()
                                n711 = Square(x=w1068) -> (x^2=w1066:dbl)
                                n712 = Square(x=w1067) -> (x^2=w1065:dbl)
                                n713 = Add(x=w1066, y=w1065) -> (x+y=w1064:dbl)
                                n714 = Square Root(x=w1064) -> (sqrt(x)=w1062:dbl)
                                n715 = local write "rd0"(w1062) -> ()
                                n716 = Greater?(x=w1062, y=w1061) -> (0:w1060:bool)
                                n717 = local write "fitting?"(w1060) -> ()
                                }
                                frame True {
                                w1097 = 0.0 ("rd0")
                                n718 = local read "abrd0"() -> (w1107:dbl[][])
                                n719 = local write "b"(w1097) -> ()
                                n720 = local write "rd0"(w1097) -> ()
                                n721 = local write "mode"(w1097) -> ()
                                n722 = Index Array(array=w1107, index (col) #1=0 ("disabled index (col)"), index (col) #2=2 ("index (col)")) -> (element #1=w1105:dbl[], element #2=w1103:dbl[])  [unwired: 2 in]
                                n723 = Equal To 0?(x=w1103) -> (x = 0?=w1104:bool[])
                                n724 = Boolean To (0,1)(Boolean=w1104) -> (0, 1=w1102:i16[])
                                n725 = Multiply(x=w1105, y=w1102) -> (x*y=w1101:dbl[])
                                n726 = Add Array Elements(numeric array=w1102) -> (sum=w1099:i16)
                                n727 = Add Array Elements(numeric array=w1101) -> (sum=w1100:dbl)
                                n728 = Divide(x=w1100, y=w1099) -> (x/y=w1098:dbl)
                                n729 = local write "a"(w1098) -> ()
                                }
                              }
                            }
                          }
                        }
                      }
                    }
                    frame Disabled {
                    }
                  }
                }
                frame True {
                  n730 = disable-structure shown="Enabled" {
                    frame Enabled {
                      n731 = flat-sequence {
                        frame #0 {
                          n732 = local read "mapidx"() -> (w1112:i32[])
                          n733 = for {
                            tunnel: w1112 -> [w1117] mode=indexing
                            tunnel: [w1114] -> w1110 mode=indexing
                            tunnel: [w1113] -> w1111 mode=indexing
                            n734 = local read "track"() -> (w1118:dbl[][])
                            n735 = Index Array(array=w1118, index (row)=w1117) -> (element=w1116:dbl[])  [unwired: 1 in]
                            n736 = Index Array(array=w1116, index #1=0 ("index")) -> (element #1=w1114:dbl, element #2=w1113:dbl)  [unwired: 1 in]
                          }
                          n737 = local write "x"(w1111) -> ()
                          n738 = Negate(x=w1110) -> (-x=w1109:dbl[])
                          n739 = local write "y"(w1109) -> ()
                        }
                        frame #1 {
                          n740 = local read "RXY"() -> (w1125:dbl[])
                          n741 = Index Array(array=w1125, index #1=0 ("index")) -> (element #1=w1121:dbl, element #2=w1120:dbl, element #3=w1119:dbl)  [unwired: 2 in]
                          n742 = Greater?(x=w1121, y=1000.0) -> (0:w1122:bool)
                          n743 = case shown="False" w1122 {
                            tunnel: w1120 -> [w1134 _]
                            tunnel: w1119 -> [w1132 _]
                            frame False {
                              n744 = local write "a"(w1132) -> ()
                              n745 = local write "mode"(1.0 ("mode")) -> ()
                              n746 = local write "fitting?"(TRUE ("fitting?")) -> ()
                              n747 = Square(x=w1132) -> (x^2=w1130:dbl)
                              n748 = Negate(x=w1134) -> (-x=w1133:dbl)
                              n749 = local write "b"(w1133) -> ()
                              n750 = Square(x=w1133) -> (x^2=w1131:dbl)
                              n751 = Add(x=w1131, y=w1130) -> (x+y=w1129:dbl)
                              n752 = Square Root(x=w1129) -> (sqrt(x)=w1128:dbl)
                              n753 = local write "rd0"(w1128) -> ()
                            }
                            frame True {
                              w1136 = 0.0 ("rd0")
                              n754 = local read "x"() -> (w1145:dbl[])
                              n755 = local write "fitting?"(TRUE ("fitting?")) -> ()
                              n756 = local read "y"() -> (w1149:dbl[])
                              n757 = local read "y"() -> (w1146:dbl[])
                              n758 = local write "b"(w1136) -> ()
                              n759 = local write "rd0"(w1136) -> ()
                              n760 = local write "mode"(w1136) -> ()
                              n761 = Array Size(array=w1145) -> (size(s)=w1153:i32)
                              n762 = Square(x=w1145) -> (x^2=w1154:dbl[])
                              n763 = Add Array Elements(numeric array=w1145) -> (sum=w1147:dbl)
                              n764 = Add Array Elements(numeric array=w1149) -> (sum=w1148:dbl)
                              n765 = Multiply(x=w1145, y=w1146) -> (x*y=w1143:dbl[])
                              n766 = Multiply(x=w1148, y=w1147) -> (x*y=w1141:dbl)
                              n767 = Add Array Elements(numeric array=w1154) -> (sum=w1152:dbl)
                              n768 = To Double Precision Float(number=w1153) -> (double precision float=w1144:dbl)
                              n769 = Add Array Elements(numeric array=w1143) -> (sum=w1142:dbl)
                              n770 = Multiply(x=w1152, y=w1144) -> (x*y=w1151:dbl)
                              n771 = Square(x=w1147) -> (x^2=w1150:dbl)
                              n772 = Multiply(x=w1144, y=w1142) -> (x*y=w1140:dbl)
                              n773 = Subtract(x=w1150, y=w1151) -> (x-y=w1138:dbl)
                              n774 = Subtract(x=w1141, y=w1140) -> (x-y=w1139:dbl)
                              n775 = Divide(x=w1139, y=w1138) -> (x/y=w1137:dbl)
                              n776 = local write "a"(w1137) -> ()
                            }
                          }
                        }
                      }
                    }
                    frame Disabled {
                      n777 = flat-sequence {
                        tunnel: [w1159] -> w1155
                        tunnel: w1155 -> [w1171]
                        frame #0 {
                          w1160 = 0.0
                          n778 = local read "mapidx"() -> (w1159:i32[])
                          n779 = local write "a"(w1160) -> ()
                          n780 = local write "b"(w1160) -> ()
                          n781 = local write "rd0"(w1160) -> ()
                          n782 = for {
                            tunnel: w1159 -> [w1165] mode=indexing
                            tunnel: [w1162] -> w1157 mode=indexing
                            tunnel: [w1161] -> w1158 mode=indexing
                            n783 = local read "track"() -> (w1166:dbl[][])
                            n784 = Index Array(array=w1166, index (row)=w1165) -> (element=w1164:dbl[])  [unwired: 1 in]
                            n785 = Index Array(array=w1164, index #1=0 ("index")) -> (element #1=w1162:dbl, element #2=w1161:dbl)  [unwired: 1 in]
                          }
                          n786 = local write "x"(w1158) -> ()
                          n787 = Negate(x=w1157) -> (-x=w1156:dbl[])
                          n788 = local write "y"(w1156) -> ()
                        }
                        frame #1 {
                          n789 = Array Size(array=w1171) -> (size(s)=w1168:i32)
                          n790 = Subtract(x=w1168, y=2) -> (x-y=w1169:i32)
                          n791 = for {
                            N: w1169 -> [_]
                            tunnel: w1168 -> [w1261]
                            tunnel: [w1260] -> w1167
                            i -> [w1262]
                            stop <- w1260 stop-if-true
                            n792 = Decrement(x=w1261) -> (x-1=w1265:i32)
                            n793 = Increment(x=w1262) -> (x+1=w1264:i32)
                            n794 = Subtract(x=w1265, y=w1264) -> (x-y=w1263:i32)
                            n795 = for {
                              N: w1263 -> [_]
                              tunnel: w1264 -> [w1272]
                              tunnel: w1262 -> [w1268]
                              tunnel: w1261 -> [w1267]
                              tunnel: [w1266] -> w1260
                              i -> [w1273]
                              stop <- w1266 stop-if-true
                              n796 = Add(x=w1272, y=w1273) -> (x+y=w1269:i32)
                              n797 = Increment(x=w1269) -> (x+1=w1270:i32)
                              n798 = Subtract(x=w1267, y=w1270) -> (x-y=w1271:i32)
                              n799 = for {
                                N: w1271 -> [_]
                                tunnel: w1270 -> [w1282]
                                tunnel: w1269 -> [w1279]
                                tunnel: w1268 -> [w1278]
                                tunnel: [w1274] -> w1266
                                i -> [w1281]
                                stop <- w1274 stop-if-true
                                n800 = Add(x=w1282, y=w1281) -> (x+y=w1280:i32)
                                n801 = flat-sequence {
                                tunnel: w1280 -> [w1285]
                                tunnel: w1279 -> [w1284]
                                tunnel: w1278 -> [w1283]
                                tunnel: [w1286] -> w1276
                                tunnel: [w1327] -> w1277
                                tunnel: w1276 -> [w1326]
                                tunnel: [w1326] -> w1275
                                tunnel: w1277 -> [w1379]
                                tunnel: w1275 -> [w1375]
                                tunnel: [w1367] -> w1274
                                frame #0 {
                                "k 2" <- w1285
                                "j 2" <- w1284
                                "i 2" <- w1283
                                }
                                frame #1 {
                                n802 = local read "y"() -> (w1322:dbl[])
                                n803 = local read "j 2"() -> (w1323:i32)
                                n804 = local read "k 2"() -> (w1321:i32)
                                n805 = local read "y"() -> (w1315:dbl[])
                                n806 = local read "k 2"() -> (w1314:i32)
                                n807 = local read "i 2"() -> (w1316:i32)
                                n808 = local read "x"() -> (w1311:dbl[])
                                n809 = local read "k 2"() -> (w1310:i32)
                                n810 = local read "x"() -> (w1325:dbl[])
                                n811 = local read "i 2"() -> (w1324:i32)
                                n812 = local read "x"() -> (w1312:dbl[])
                                n813 = local read "j 2"() -> (w1313:i32)
                                n814 = local read "y"() -> (w1308:dbl[])
                                n815 = local read "i 2"() -> (w1309:i32)
                                n816 = local read "j 2"() -> (w1307:i32)
                                n817 = Index Array(array=w1325, index=w1324) -> (element=w1300:dbl)
                                n818 = Index Array(array=w1312, index=w1313) -> (element=w1297:dbl)
                                n819 = Index Array(array=w1308, index #1=w1309, index #2=w1307) -> (element #1=w1306:dbl, element #2=w1305:dbl)
                                n820 = Index Array(array=w1322, index #1=w1323, index #2=w1321) -> (element #1=w1320:dbl, element #2=w1319:dbl)
                                n821 = Index Array(array=w1315, index #1=w1314, index #2=w1316) -> (element #1=w1317:dbl, element #2=w1318:dbl)
                                n822 = Index Array(array=w1311, index=w1310) -> (element=w1294:dbl)
                                n823 = Subtract(x=w1320, y=w1319) -> (x-y=w1304:dbl)
                                n824 = Subtract(x=w1317, y=w1318) -> (x-y=w1303:dbl)
                                n825 = Subtract(x=w1306, y=w1305) -> (x-y=w1302:dbl)
                                n826 = Compound Arithmetic op=MULTIPLY(w1304, w1303, w1302) -> (w1290:dbl)
                                n827 = Multiply(x=w1300, y=w1304) -> (x*y=w1301:dbl)
                                n828 = Multiply(x=w1297, y=w1303) -> (x*y=w1298:dbl)
                                n829 = Multiply(x=w1294, y=w1302) -> (x*y=w1295:dbl)
                                n830 = Multiply(x=w1300, y=w1301) -> (x*y=w1299:dbl)
                                n831 = Multiply(x=w1297, y=w1298) -> (x*y=w1296:dbl)
                                n832 = Multiply(x=w1294, y=w1295) -> (x*y=w1293:dbl)
                                n833 = Compound Arithmetic op=ADD(w1301, w1298, w1295) -> (w1286:dbl)
                                n834 = Compound Arithmetic op=ADD(w1299, w1296, w1293) -> (w1291:dbl)
                                n835 = Subtract(x=w1291, y=w1290) -> (x-y=w1289:dbl)
                                n836 = Divide(x=w1289, y=w1286) -> (x/y=w1288:dbl)
                                n837 = local read "a"() -> (w1292:dbl)
                                n838 = Add(x=w1292, y=w1288) -> (x+y=w1287:dbl)
                                n839 = local write "a"(w1287) -> ()
                                }
                                frame #2 {
                                n840 = local read "x"() -> (w1331:dbl[])
                                n841 = local read "j 2"() -> (w1330:i32)
                                n842 = local read "k 2"() -> (w1332:i32)
                                n843 = local read "x"() -> (w1338:dbl[])
                                n844 = local read "k 2"() -> (w1339:i32)
                                n845 = local read "i 2"() -> (w1337:i32)
                                n846 = local read "y"() -> (w1342:dbl[])
                                n847 = local read "k 2"() -> (w1343:i32)
                                n848 = local read "x"() -> (w1345:dbl[])
                                n849 = local read "i 2"() -> (w1344:i32)
                                n850 = local read "j 2"() -> (w1346:i32)
                                n851 = local read "y"() -> (w1328:dbl[])
                                n852 = local read "i 2"() -> (w1329:i32)
                                n853 = local read "y"() -> (w1341:dbl[])
                                n854 = local read "j 2"() -> (w1340:i32)
                                n855 = Index Array(array=w1345, index #1=w1344, index #2=w1346) -> (element #1=w1347:dbl, element #2=w1348:dbl)
                                n856 = Index Array(array=w1328, index=w1329) -> (element=w1353:dbl)
                                n857 = Index Array(array=w1341, index=w1340) -> (element=w1356:dbl)
                                n858 = Index Array(array=w1331, index #1=w1330, index #2=w1332) -> (element #1=w1333:dbl, element #2=w1334:dbl)
                                n859 = Index Array(array=w1338, index #1=w1339, index #2=w1337) -> (element #1=w1336:dbl, element #2=w1335:dbl)
                                n860 = Index Array(array=w1342, index=w1343) -> (element=w1359:dbl)
                                n861 = Subtract(x=w1347, y=w1348) -> (x-y=w1351:dbl)
                                n862 = Subtract(x=w1333, y=w1334) -> (x-y=w1349:dbl)
                                n863 = Subtract(x=w1336, y=w1335) -> (x-y=w1350:dbl)
                                n864 = Compound Arithmetic op=MULTIPLY(w1349, w1350, w1351) -> (w1363:dbl)
                                n865 = Multiply(x=w1353, y=w1349) -> (x*y=w1352:dbl)
                                n866 = Multiply(x=w1359, y=w1351) -> (x*y=w1358:dbl)
                                n867 = Multiply(x=w1356, y=w1350) -> (x*y=w1355:dbl)
                                n868 = Multiply(x=w1353, y=w1352) -> (x*y=w1354:dbl)
                                n869 = Multiply(x=w1356, y=w1355) -> (x*y=w1357:dbl)
                                n870 = Multiply(x=w1359, y=w1358) -> (x*y=w1360:dbl)
                                n871 = Compound Arithmetic op=ADD(w1352, w1355, w1358) -> (w1327:dbl)
                                n872 = Compound Arithmetic op=ADD(w1354, w1357, w1360) -> (w1362:dbl)
                                n873 = Subtract(x=w1362, y=w1363) -> (x-y=w1364:dbl)
                                n874 = Divide(x=w1364, y=w1327) -> (x/y=w1365:dbl)
                                n875 = local read "b"() -> (w1361:dbl)
                                n876 = Add(x=w1361, y=w1365) -> (x+y=w1366:dbl)
                                n877 = local write "b"(w1366) -> ()
                                }
                                frame #3 {
                                n878 = Multiply(x=w1379, y=w1375) -> (x*y=w1383:dbl)
                                n879 = Absolute Value(x=w1375) -> (abs(x)=w1377:dbl)
                                n880 = Absolute Value(x=w1379) -> (abs(x)=w1381:dbl)
                                n881 = Sign(1:w1383) -> (0:w1382:dbl)
                                n882 = Greater?(x=w1377, y=1e-12) -> (0:w1374:bool)
                                n883 = Greater?(x=w1381, y=1e-12) -> (0:w1378:bool)
                                n884 = Absolute Value(x=w1382) -> (abs(x)=w1373:dbl)
                                n885 = Boolean To (0,1)(Boolean=w1374) -> (0, 1=w1370:i16)
                                n886 = Boolean To (0,1)(Boolean=w1378) -> (0, 1=w1372:i16)
                                n887 = To Double Precision Float(number=w1370) -> (double precision float=w1369:dbl)
                                n888 = To Double Precision Float(number=w1372) -> (double precision float=w1371:dbl)
                                n889 = Compound Arithmetic op=MULTIPLY(w1371, w1373, w1369) -> (w1368:dbl)
                                n890 = Equal To 0?(x=w1368) -> (x = 0?=w1367:bool)
                                }
                                }
                              }
                            }
                          }
                          n891 = case shown="False" w1167 {
                            frame False {
                              n892 = flat-sequence {
                                frame #0 {
                                n893 = local read "x"() -> (w1195:dbl[])
                                n894 = local write "mode"(1.0 ("mode")) -> ()
                                n895 = Array Size(array=w1195) -> (size(s)=w1192:i32)
                                n896 = Subtract(x=w1192, y=3) -> (x-y=w1190:i32)
                                n897 = for {
                                N: w1192 -> [_]
                                shift-right: [w1201] -> w1187
                                shift-left: 1 -> [w1200]
                                i -> [w1203]
                                n898 = Increment(x=w1203) -> (x+1=w1202:i32)
                                n899 = Multiply(x=w1200, y=w1202) -> (x*y=w1201:i32)
                                }
                                n900 = for {
                                N: w1190 -> [_]
                                shift-right: [w1197] -> w1189
                                shift-left: 1 -> [w1196]
                                i -> [w1199]
                                n901 = Increment(x=w1199) -> (x+1=w1198:i32)
                                n902 = Multiply(x=w1196, y=w1198) -> (x*y=w1197:i32)
                                }
                                n903 = To Double Precision Float(number=w1187) -> (double precision float=w1184:dbl)
                                n904 = Multiply(x=w1189, y=6) -> (x*y=w1186:i32)
                                n905 = To Double Precision Float(number=w1186) -> (double precision float=w1185:dbl)
                                n906 = Divide(x=w1184, y=w1185) -> (x/y=w1183:dbl)
                                n907 = Multiply(x=2.0, y=w1183) -> (x*y=w1179:dbl)
                                n908 = local read "a"() -> (w1181:dbl)
                                n909 = local read "b"() -> (w1180:dbl)
                                n910 = Divide(x=w1181, y=w1179) -> (x/y=w1178:dbl)
                                n911 = Divide(x=w1180, y=w1179) -> (x/y=w1177:dbl)
                                n912 = local write "a"(w1178) -> ()
                                n913 = local write "b"(w1177) -> ()
                                n914 = Square(x=w1178) -> (x^2=w1175:dbl)
                                n915 = Square(x=w1177) -> (x^2=w1176:dbl)
                                n916 = Add(x=w1175, y=w1176) -> (x+y=w1174:dbl)
                                n917 = Square Root(x=w1174) -> (sqrt(x)=w1173:dbl)
                                n918 = local write "rd0"(w1173) -> ()
                                }
                                frame #1 {
                                n919 = local read "y"() -> (w1209:dbl[])
                                n920 = local read "x"() -> (w1218:dbl[])
                                n921 = local read "a"() -> (w1217:dbl)
                                n922 = local read "b"() -> (w1216:dbl)
                                n923 = Array Size(array=w1209) -> (size(s)=w1207:i32)
                                n924 = Subtract(x=w1218, y=w1217) -> (x-y=w1215:dbl[])
                                n925 = Subtract(x=w1209, y=w1216) -> (x-y=w1214:dbl[])
                                n926 = Square(x=w1215) -> (x^2=w1213:dbl[])
                                n927 = Square(x=w1214) -> (x^2=w1212:dbl[])
                                n928 = Add(x=w1213, y=w1212) -> (x+y=w1211:dbl[])
                                n929 = Square Root(x=w1211) -> (sqrt(x)=w1210:dbl[])
                                n930 = Add Array Elements(numeric array=w1210) -> (sum=w1208:dbl)
                                n931 = Divide(x=w1208, y=w1207) -> (x/y=w1206:dbl)
                                n932 = Greater?(x=w1206, y=1000.0) -> (0:w1204:bool)
                                n933 = case shown="True" w1204 {
                                frame False {
                                }
                                frame True {
                                w1220 = 0.0 ("rd0")
                                n934 = local read "x"() -> (w1229:dbl[])
                                n935 = local write "fitting?"(TRUE ("fitting?")) -> ()
                                n936 = local read "y"() -> (w1233:dbl[])
                                n937 = local write "b"(w1220) -> ()
                                n938 = local write "rd0"(w1220) -> ()
                                n939 = local write "mode"(w1220) -> ()
                                n940 = local read "y"() -> (w1230:dbl[])
                                n941 = Array Size(array=w1229) -> (size(s)=w1237:i32)
                                n942 = Square(x=w1229) -> (x^2=w1238:dbl[])
                                n943 = Add Array Elements(numeric array=w1229) -> (sum=w1231:dbl)
                                n944 = Add Array Elements(numeric array=w1233) -> (sum=w1232:dbl)
                                n945 = Multiply(x=w1229, y=w1230) -> (x*y=w1227:dbl[])
                                n946 = Multiply(x=w1232, y=w1231) -> (x*y=w1225:dbl)
                                n947 = Add Array Elements(numeric array=w1238) -> (sum=w1236:dbl)
                                n948 = To Double Precision Float(number=w1237) -> (double precision float=w1228:dbl)
                                n949 = Multiply(x=w1236, y=w1228) -> (x*y=w1235:dbl)
                                n950 = Add Array Elements(numeric array=w1227) -> (sum=w1226:dbl)
                                n951 = Square(x=w1231) -> (x^2=w1234:dbl)
                                n952 = Multiply(x=w1228, y=w1226) -> (x*y=w1224:dbl)
                                n953 = Subtract(x=w1234, y=w1235) -> (x-y=w1222:dbl)
                                n954 = Subtract(x=w1225, y=w1224) -> (x-y=w1223:dbl)
                                n955 = Divide(x=w1223, y=w1222) -> (x/y=w1221:dbl)
                                n956 = local write "a"(w1221) -> ()
                                }
                                }
                                }
                              }
                            }
                            frame True {
                              w1241 = 0.0 ("rd0")
                              n957 = local read "x"() -> (w1250:dbl[])
                              n958 = local write "mode"(0.0 ("mode")) -> ()
                              n959 = local write "fitting?"(TRUE ("fitting?")) -> ()
                              n960 = local read "y"() -> (w1254:dbl[])
                              n961 = local read "y"() -> (w1251:dbl[])
                              n962 = local write "b"(w1241) -> ()
                              n963 = local write "rd0"(w1241) -> ()
                              n964 = Array Size(array=w1250) -> (size(s)=w1258:i32)
                              n965 = Square(x=w1250) -> (x^2=w1259:dbl[])
                              n966 = Add Array Elements(numeric array=w1250) -> (sum=w1252:dbl)
                              n967 = Add Array Elements(numeric array=w1254) -> (sum=w1253:dbl)
                              n968 = Multiply(x=w1250, y=w1251) -> (x*y=w1248:dbl[])
                              n969 = Multiply(x=w1253, y=w1252) -> (x*y=w1246:dbl)
                              n970 = Add Array Elements(numeric array=w1259) -> (sum=w1257:dbl)
                              n971 = To Double Precision Float(number=w1258) -> (double precision float=w1249:dbl)
                              n972 = Add Array Elements(numeric array=w1248) -> (sum=w1247:dbl)
                              n973 = Multiply(x=w1257, y=w1249) -> (x*y=w1256:dbl)
                              n974 = Square(x=w1252) -> (x^2=w1255:dbl)
                              n975 = Multiply(x=w1249, y=w1247) -> (x*y=w1245:dbl)
                              n976 = Subtract(x=w1255, y=w1256) -> (x-y=w1243:dbl)
                              n977 = Subtract(x=w1246, y=w1245) -> (x-y=w1244:dbl)
                              n978 = Divide(x=w1244, y=w1243) -> (x/y=w1242:dbl)
                              n979 = local write "a"(w1242) -> ()
                            }
                          }
                        }
                        frame #2 {
                          n980 = local read "rd0"() -> (w1387:dbl)
                          n981 = local read "a"() -> (w1389:dbl)
                          n982 = local read "b"() -> (w1388:dbl)
                          n983 = Build Array(w1389, w1388, w1387) -> (w1385:dbl[])
                          n984 = local read "abrd0"() -> (w1386:dbl[][])
                          n985 = Build Array (concatenate)(w1386, w1385) -> (w1384:dbl[][])
                          n986 = local write "abrd0"(w1384) -> ()
                        }
                      }
                    }
                  }
                }
              }
            }
          }
        }
        frame #5 {
          n987 = disable-structure shown="Enabled" {
            frame Enabled {
              n988 = local read "fitting?"() -> (w1393:bool)
              n989 = case shown="True" w1393 {
                tunnel: [_ w1419] -> w1390
                frame False {
                }
                frame True {
                  n990 = flat-sequence {
                    tunnel: [w1501] -> w1419
                    frame #0 {
                      n991 = local read "mode"() -> (w1425:dbl)
                      n992 = Equal To 0?(x=w1425) -> (x = 0?=w1424:bool)
                      n993 = case shown="True" w1424 {
                        tunnel: [1.0 w1476] -> w1423
                        tunnel: [w1434 w1477] -> w1422
                        tunnel: [w1427 w1474] -> w1421
                        tunnel: [w1426 1.0] -> w1420
                        frame False {
                          n994 = local read "data"() -> (w1447:dbl[][])
                          n995 = local read "b"() -> (w1433:dbl)
                          n996 = local read "a"() -> (w1432:dbl)
                          n997 = Index Array(array=w1447, index (col) #1=1 ("disabled index (col)"), index (col) #2=0 ("index (col)")) -> (element #1=w1442:dbl[], element #2=w1444:dbl[])  [unwired: 2 in]
                          n998 = Negate(x=w1433) -> (-x=w1431:dbl)
                          n999 = Negate(x=w1432) -> (-x=w1430:dbl)
                          n1000 = local read "b"() -> (w1441:dbl)
                          n1001 = local read "a"() -> (w1443:dbl)
                          n1002 = Inverse Tangent (2 Input)(1:w1430, 2:w1431) -> (0:w1428:dbl)
                          n1003 = Subtract(x=w1444, y=w1443) -> (x-y=w1439:dbl[])
                          n1004 = Subtract(x=w1441, y=w1442) -> (x-y=w1440:dbl[])
                          n1005 = Less Than 0?(x=w1428) -> (x < 0?=w1429:bool)
                          n1006 = case shown="True" w1429 {
                            tunnel: w1428 -> [w1450 w1462]
                            tunnel: [w1449 w1461] -> w1427
                            frame True {
                              n1007 = local read "data"() -> (w1458:dbl[][])
                              n1008 = Index Array(array=w1458, index (col) #1=1 ("disabled index (col)"), index (col) #2=0 ("index (col)")) -> (element #1=w1456:dbl[], element #2=w1454:dbl[])  [unwired: 2 in]
                              n1009 = local read "b"() -> (w1457:dbl)
                              n1010 = local read "a"() -> (w1455:dbl)
                              n1011 = Subtract(x=w1454, y=w1455) -> (x-y=w1452:dbl[])
                              n1012 = Subtract(x=w1456, y=w1457) -> (x-y=w1453:dbl[])
                              n1013 = Inverse Tangent (2 Input)(1:w1452, 2:w1453) -> (0:w1451:dbl[])
                              n1014 = Subtract(x=w1451, y=w1450) -> (x-y=w1449:dbl[])
                            }
                            frame False {
                              n1015 = local read "data"() -> (w1470:dbl[][])
                              n1016 = Index Array(array=w1470, index (col) #1=1 ("disabled index (col)"), index (col) #2=0 ("index (col)")) -> (element #1=w1468:dbl[], element #2=w1466:dbl[])  [unwired: 2 in]
                              n1017 = local read "b"() -> (w1469:dbl)
                              n1018 = local read "a"() -> (w1467:dbl)
                              n1019 = Subtract(x=w1466, y=w1467) -> (x-y=w1464:dbl[])
                              n1020 = Subtract(x=w1468, y=w1469) -> (x-y=w1465:dbl[])
                              n1021 = Inverse Tangent (2 Input)(1:w1464, 2:w1465) -> (0:w1463:dbl[])
                              n1022 = Subtract(x=w1462, y=w1463) -> (x-y=w1461:dbl[])
                            }
                          }
                          n1023 = Square(x=w1440) -> (x^2=w1438:dbl[])
                          n1024 = Square(x=w1439) -> (x^2=w1437:dbl[])
                          n1025 = Add(x=w1438, y=w1437) -> (x+y=w1436:dbl[])
                          n1026 = Square Root(x=w1436) -> (sqrt(x)=w1435:dbl[])
                          n1027 = local read "rd0"() -> (w1426:dbl)
                          n1028 = Subtract(x=w1435, y=w1426) -> (x-y=w1434:dbl[])
                        }
                        frame True {
                          n1029 = local read "data"() -> (w1483:dbl[][])
                          n1030 = local read "a"() -> (w1480:dbl)
                          n1031 = Inverse Tangent(1:w1480) -> (0:w1484:dbl)
                          n1032 = Index Array(array=w1483, index (col) #1=1 ("disabled index (col)"), index (col) #2=0 ("index (col)")) -> (element #1=w1478:dbl[], element #2=w1475:dbl[])  [unwired: 2 in]
                          n1033 = Multiply(x=w1475, y=w1480) -> (x*y=w1479:dbl[])
                          n1034 = Cosine(x=w1484) -> (cos(x)=w1476:dbl)
                          n1035 = Subtract(x=w1478, y=w1479) -> (x-y=w1477:dbl[])
                          n1036 = Divide(x=w1475, y=w1476) -> (x/y=w1474:dbl[])
                        }
                      }
                      "cta" <- w1423
                      "rdi" <- w1422
                      "xt" <- w1421
                      "t2x" <- w1420
                    }
                    frame #1 {
                      n1037 = local read "xt"() -> (w1494:dbl[])
                      n1038 = local read "t2x"() -> (w1493:dbl)
                      n1039 = Compound Arithmetic op=MULTIPLY(5.0, w1494, w1493) -> (w1491:dbl[])
                      n1040 = Round To Nearest(number=w1491) -> (nearest integer value=w1490:dbl[])
                      "xx" <- w1490
                      n1041 = Sort 1D Array(array=w1490) -> (sorted array=w1488:dbl[])
                      n1042 = for {
                        shift-right: [w1495] -> _
                        shift-left: -inf -> [w1500]
                        shift-right: [w1496] -> w1486
                        shift-left: i16 0 -> [w1497]
                        tunnel: w1488 -> [w1495] mode=indexing
                        n1043 = Not Equal?(x=w1500, y=w1495) -> (x != y?=w1499:bool)
                        n1044 = Boolean To (0,1)(Boolean=w1499) -> (0, 1=w1498:i16)
                        n1045 = Add(x=w1498, y=w1497) -> (x+y=w1496:i16)
                      }
                      n1046 = To Double Precision Float(number=w1486) -> (double precision float=→"den":dbl)
                    }
                    frame #2 {
                      w1518 = 0.0
                      n1047 = local read "lineseedorigin"() -> (w1507:dbl[])
                      n1048 = for {
                        tunnel: w1507 -> [w1524] mode=indexing
                        tunnel: [w1523] -> w1519 mode=indexing
                        n1049 = local read "rdi"() -> (w1538:dbl[])
                        n1050 = local read "D_threshold"() -> (w1533:dbl)
                        n1051 = Subtract(x=w1538, y=w1524) -> (x-y=w1537:dbl[])
                        n1052 = Absolute Value(x=w1537) -> (abs(x)=w1536:dbl[])
                        n1053 = local read "cta"() -> (w1535:dbl)
                        n1054 = Multiply(x=w1535, y=w1536) -> (x*y=w1534:dbl[])
                        n1055 = Less?(x=w1534, y=w1533) -> (x < y?=w1532:bool[])
                        n1056 = Boolean To (0,1)(Boolean=w1532) -> (0, 1=w1531:i16[])
                        n1057 = To Double Precision Float(number=w1531) -> (double precision float=w1530:dbl[])
                        n1058 = local read "xx"() -> (w1529:dbl[])
                        n1059 = Multiply(x=w1530, y=w1529) -> (x*y=w1527:dbl[])
                        n1060 = disable-structure shown="Enabled" {
                          disable-tunnel: [w1543 _] -> w1528
                          disable-tunnel: w1527 -> [w1539 _]
                          frame Enabled {
                            n1061 = Sort 1D Array(array=w1539) -> (sorted array=w1541:dbl[])
                            n1062 = for {
                              shift-right: [w1544] -> _
                              shift-left: -inf -> [w1549]
                              shift-right: [w1545] -> w1543
                              shift-left: i16 0 -> [w1546]
                              tunnel: w1541 -> [w1544] mode=indexing
                              n1063 = Not Equal?(x=w1549, y=w1544) -> (x != y?=w1548:bool)
                              n1064 = Boolean To (0,1)(Boolean=w1548) -> (0, 1=w1547:i16)
                              n1065 = Add(x=w1547, y=w1546) -> (x+y=w1545:i16)
                            }
                          }
                          frame Disabled {
                          }
                        }
                        n1066 = To Double Precision Float(number=w1528) -> (double precision float=w1526:dbl)
                        n1067 = local read "den"() -> (w1525:dbl)
                        n1068 = Divide(x=w1526, y=w1525) -> (x/y=w1523:dbl)
                      }
                      n1069 = Array Size(array=w1519) -> (size(s)=w1520:i32)
                      n1070 = Subtract(x=w1520, y=2) -> (x-y=w1521:i32)
                      n1071 = for {
                        N: w1521 -> [_]
                        tunnel: [w1574] -> w1517 mode=indexing
                        tunnel: w1519 -> [w1573]
                        i -> [w1576]
                        n1072 = Array Subset(array=w1573, index=w1576, length=3) -> (w1575:dbl[])
                        n1073 = Index Array(array=w1575, index #1=1 ("index"), index #3=0 ("disabled index (col)"), index #6=0 ("index")) -> (element #1=w1554:dbl, element #2=w1563:dbl, element #3=w1572:dbl, element #4=w1571:dbl, element #5=w1570:dbl, element #6=w1568:dbl, element #7=w1567:dbl)  [unwired: 4 in]
                        n1074 = Greater Or Equal?(x=w1554, y=w1563) -> (x >= y?=w1562:bool)
                        n1075 = Less Or Equal?(x=w1568, y=w1567) -> (x <= y?=w1565:bool)
                        n1076 = Less?(x=w1572, y=w1571) -> (x < y?=w1561:bool)
                        n1077 = Greater?(x=w1571, y=w1570) -> (0:w1566:bool)
                        n1078 = And(x=w1562, y=w1561) -> (x .and. y?=w1560:bool)
                        n1079 = And(x=w1561, y=w1566) -> (x .and. y?=w1559:bool)
                        n1080 = And(x=w1566, y=w1565) -> (x .and. y?=w1558:bool)
                        n1081 = Compound Arithmetic op=OR(w1560, w1559, w1558) -> (w1557:bool)
                        n1082 = Boolean To (0,1)(Boolean=w1557) -> (0, 1=w1556:i16)
                        n1083 = To Double Precision Float(number=w1556) -> (double precision float=w1555:dbl)
                        n1084 = Multiply(x=w1554, y=w1555) -> (x*y=w1574:dbl)
                      }
                      n1085 = Build Array (concatenate)(w1518, w1517, w1518) -> (w1516:dbl[])
                      n1086 = Build Cluster Array(w1516, w1507) -> (w1515:cluster{dbl, dbl}[])
                      n1087 = Sort 1D Array(array=w1515) -> (sorted array=w1514:cluster{dbl, dbl}[])
                      n1088 = Reverse 1D Array(array=w1514) -> (reversed array=w1513:cluster{dbl, dbl}[])
                      n1089 = for {
                        tunnel: w1513 -> [w1553] mode=indexing
                        tunnel: [w1550] -> w1511 mode=indexing
                        n1090 = Unbundle(w1553) -> (w1551:dbl, w1552:dbl)
                        n1091 = Build Array(w1552, w1551) -> (w1550:dbl[])
                      }
                      n1092 = Index Array(array=w1511, index (col)=1 ("disabled index (col)")) -> (element=w1506:dbl[])  [unwired: 1 in]
                      n1093 = Greater?(x=w1506, y=0.05) -> (0:w1505:bool[])
                      n1094 = Boolean To (0,1)(Boolean=w1505) -> (0, 1=w1510:i16[])
                      n1095 = Add Array Elements(numeric array=w1510) -> (sum=w1509:i16)
                      n1096 = Array Subset(array=w1511, index (row)=0 ("index"), length (row)=w1509) -> (w1501:dbl[][])  [unwired: 2 in]
                      n1097 = Empty Array?(array=w1501) -> (empty?=w1503:bool)
                      n1098 = Not(x=w1503) -> (.not. x?=w1502:bool)
                      n1099 = local write "fitting?"(w1502) -> ()
                    }
                  }
                }
              }
              n1100 = disable-structure shown="Enabled" {
                disable-tunnel: [w1395 TRUE w1402] -> w1392
                disable-tunnel: w1390 -> [w1394 _ w1416]
                frame Disabled {
                  n1101 = Array Size(array=w1394) -> (size(s)=w1399:i32[])
                  n1102 = Index Array(array=w1399, index=0) -> (element=w1397:i32)
                  n1103 = Less Or Equal?(x=w1397, y=28) -> (x <= y?=w1395:bool)
                }
                frame Enabled {
                }
                frame Disabled {
                  n1104 = Index Array(array=w1416, index (col)=0 ("disabled index (col)")) -> (element=w1414:dbl[])  [unwired: 1 in]
                  n1105 = Sort 1D Array(array=w1414) -> (sorted array=w1411:dbl[])
                  n1106 = local read "min lane width"() -> (w1405:dbl)
                  n1107 = Array Size(array=w1411) -> (size(s)=w1413:i32)
                  n1108 = Decrement(x=w1413) -> (x-1=w1412:i32)
                  n1109 = Multiply(x=0.5, y=w1405) -> (x*y=w1403:dbl)
                  n1110 = Array Subset(array=w1411, length=w1412) -> (w1408:dbl[])  [unwired: 1 in]
                  n1111 = Array Subset(array=w1411, index=1) -> (w1409:dbl[])  [unwired: 1 in]
                  n1112 = Subtract(x=w1409, y=w1408) -> (x-y=w1407:dbl[])
                  "x-y" <- w1407
                  n1113 = Array Max & Min(array=w1407) -> (max value=w1406:dbl, min value=→"min value 2":dbl)  [unwired: 2 out]
                  n1114 = Greater?(x=w1406, y=w1403) -> (0:w1402:bool)
                }
              }
              n1115 = case shown="True" w1392 {
                tunnel: [_ w1418] -> w1391
                tunnel: w1390 -> [_ w1418]
                frame False {
                  n1116 = local write "fitting?"(FALSE ("fitting?")) -> ()
                }
                frame True {
                }
              }
              "lineseed0" <- w1391
            }
            frame Disabled {
            }
          }
        }
        frame #6 {
          n1117 = disable-structure shown="Enabled" {
            frame Enabled {
              n1118 = local read "fitting?"() -> (w1580:bool)
              n1119 = case shown="False" w1580 {
                tunnel: [_ w1581] -> w1579
                frame False {
                }
                frame True {
                  n1120 = flat-sequence {
                    tunnel: [w1612] -> w1581
                    frame #0 {
                      n1121 = local read "lineseed0"() -> (w1582:dbl[][])
                      n1122 = Index Array(array=w1582, index (row)=0) -> (element=w1583:dbl[])  [unwired: 1 in]
                      n1123 = for {
                        tunnel: w1583 -> [w1588]
                        tunnel: w1582 -> [w1587] mode=indexing
                        stop <- w1585 stop-if-true
                        n1124 = Multiply(x=w1587, y=w1588) -> (x*y=w1593:dbl[])
                        n1125 = Index Array(array=w1593, index=0) -> (element=w1591:dbl)
                        n1126 = Sign(1:w1591) -> (0:w1590:dbl)
                        n1127 = Less Than 0?(x=w1590) -> (x < 0?=w1589:bool)
                        n1128 = case shown="True" w1589 {
                          tunnel: w1588 -> [_ w1597]
                          tunnel: w1587 -> [_ w1596]
                          tunnel: [_ w1595] -> w1586
                          tunnel: [_ TRUE] -> w1585
                          frame False {
                          }
                          frame True {
                            n1129 = Build Array(w1596, w1597) -> (w1595:dbl[][])
                          }
                        }
                        "lineseed1" <- w1586
                      }
                    }
                    frame #1 {
                      n1130 = disable-structure shown="Enabled" {
                        disable-tunnel: [w1599 _] -> w1598
                        frame Enabled {
                          n1131 = local read "lineseed1"() -> (w1605:dbl[][])
                          n1132 = Index Array(array=w1605, index (col)=0 ("disabled index (col)")) -> (element=w1603:dbl[])  [unwired: 1 in]
                          n1133 = Index Array(array=w1603, index #1=0 ("index")) -> (element #1=w1601:dbl, element #2=w1600:dbl)  [unwired: 1 in]
                          n1134 = Greater?(x=w1601, y=w1600) -> (0:w1599:bool)
                        }
                        frame Disabled {
                        }
                      }
                      n1135 = case shown="False" w1598 {
                        frame False {
                          n1136 = local read "lineseed1"() -> (w1611:dbl[][])
                          n1137 = Index Array(array=w1611, index (row) #1=1 ("index (row)"), index (row) #2=0 ("index (row)")) -> (element #1=w1608:dbl[], element #2=w1607:dbl[])  [unwired: 2 in]
                          n1138 = Build Array(w1608, w1607) -> (w1606:dbl[][])
                          n1139 = local write "lineseed1"(w1606) -> ()
                        }
                        frame True {
                        }
                      }
                    }
                    frame #2 {
                      w1615 = 0
                      n1140 = local read "lineseed1"() -> (w1614:dbl[][])
                      n1141 = while {
                        shift-right: [w1628] -> w1613
                        shift-left: w1615 -> [w1633]
                        shift-right: [w1632] -> w1612
                        shift-left: w1614 -> [w1634]
                        stop <- w1627 continue-if-true
                        n1142 = Index Array(array=w1634, index (col)=0 ("disabled index (col)")) -> (element=w1645:dbl[])  [unwired: 1 in]
                        n1143 = local read "min lane width"() -> (w1641:dbl)
                        n1144 = Index Array(array=w1645, index #1=w1633) -> (element #1=w1626:dbl, element #2=w1624:dbl)  [unwired: 1 in]
                        n1145 = Add(x=w1626, y=w1624) -> (x+y=w1637:dbl)
                        n1146 = Subtract(x=w1626, y=w1624) -> (x-y=w1644:dbl)
                        n1147 = Divide(x=w1626, y=3.0) -> (x/y=w1618:dbl)
                        n1148 = Divide(x=w1624, y=3.0) -> (x/y=w1622:dbl)
                        n1149 = local read "cta"() -> (w1643:dbl)
                        n1150 = Multiply(x=w1618, y=2.0) -> (x*y=w1617:dbl)
                        n1151 = Multiply(x=w1622, y=1.0) -> (x*y=w1620:dbl)
                        n1152 = Multiply(x=w1641, y=2.0) -> (x*y=w1639:dbl)
                        n1153 = Multiply(x=0.5, y=w1637) -> (x*y=w1635:dbl)
                        n1154 = Multiply(x=w1644, y=w1643) -> (x*y=w1642:dbl)
                        n1155 = Add(x=w1617, y=w1620) -> (x+y=w1619:dbl)
                        n1156 = Greater Or Equal?(x=w1642, y=w1639) -> (x >= y?=w1638:bool)
                        n1157 = case shown="True" w1638 {
                          tunnel: w1635 -> [_ w1663]
                          tunnel: w1634 -> [w1647 w1655]
                          tunnel: w1633 -> [w1649 w1654]
                          tunnel: [w1647 w1652] -> w1632
                          tunnel: [w1648 w1651] -> w1628
                          tunnel: w1619 -> [_ w1650]
                          frame False {
                            n1158 = Increment(x=w1649) -> (x+1=w1648:i32)
                          }
                          frame True {
                            n1159 = local read "D_threshold"() -> (w1658:dbl)
                            n1160 = local read "lineseed0"() -> (w1666:dbl[][])
                            n1161 = Multiply(x=w1658, y=4.0) -> (x*y=w1657:dbl)
                            n1162 = Index Array(array=w1666, index (col)=0 ("disabled index (col)")) -> (element=w1664:dbl[])  [unwired: 1 in]
                            n1163 = Subtract(x=w1663, y=w1664) -> (x-y=w1662:dbl[])
                            n1164 = Absolute Value(x=w1662) -> (abs(x)=w1661:dbl[])
                            n1165 = Array Max & Min(array=w1661) -> (min value=w1660:dbl, min index (indices)=w1653:i32)  [unwired: 2 out]
                            n1166 = Less Or Equal?(x=w1660, y=w1657) -> (x <= y?=w1656:bool)
                            n1167 = case shown="False" w1656 {
                              tunnel: w1655 -> [w1682 w1704]
                              tunnel: w1654 -> [w1679 w1696]
                              tunnel: w1653 -> [_ w1699]
                              tunnel: [w1667 w1697] -> w1652
                              tunnel: [w1680 w1696] -> w1651
                              tunnel: w1650 -> [w1681 _]
                              frame False {
                                n1168 = local read "D_threshold"() -> (w1671:dbl)
                                n1169 = local read "lineseed0"() -> (w1678:dbl[][])
                                n1170 = Multiply(x=w1671, y=5.0) -> (x*y=w1670:dbl)
                                n1171 = Index Array(array=w1678, index (col)=0 ("disabled index (col)")) -> (element=w1676:dbl[])  [unwired: 1 in]
                                n1172 = Subtract(x=w1681, y=w1676) -> (x-y=w1675:dbl[])
                                n1173 = Absolute Value(x=w1675) -> (abs(x)=w1674:dbl[])
                                n1174 = Array Max & Min(array=w1674) -> (min value=w1673:dbl, min index (indices)=w1668:i32)  [unwired: 2 out]
                                n1175 = Less Or Equal?(x=w1673, y=w1670) -> (x <= y?=w1669:bool)
                                n1176 = case shown="False" w1669 {
                                tunnel: w1682 -> [w1685 w1694]
                                tunnel: w1679 -> [w1684 w1686]
                                tunnel: w1668 -> [_ w1689]
                                tunnel: [w1685 w1687] -> w1667
                                tunnel: [w1683 w1686] -> w1680
                                frame False {
                                n1177 = Increment(x=w1684) -> (x+1=w1683:i32)
                                }
                                frame True {
                                n1178 = Increment(x=w1686) -> (x+1=w1693:i32)
                                n1179 = local read "lineseed0"() -> (w1690:dbl[][])
                                n1180 = Array Subset(array=w1694, index (row)=w1693) -> (w1691:dbl[][])  [unwired: 3 in]
                                n1181 = Array Subset(array=w1694, index (row)=0 ("index"), length (row)=w1693) -> (w1692:dbl[][])  [unwired: 2 in]
                                n1182 = Index Array(array=w1690, index (row)=w1689) -> (element=w1688:dbl[])  [unwired: 1 in]
                                n1183 = Build Array (concatenate)(w1692, w1688, w1691) -> (w1687:dbl[][])
                                }
                                }
                              }
                              frame True {
                                n1184 = Increment(x=w1696) -> (x+1=w1703:i32)
                                n1185 = local read "lineseed0"() -> (w1700:dbl[][])
                                n1186 = Array Subset(array=w1704, index (row)=w1703) -> (w1701:dbl[][])  [unwired: 3 in]
                                n1187 = Index Array(array=w1700, index (row)=w1699) -> (element=w1698:dbl[])  [unwired: 1 in]
                                n1188 = Array Subset(array=w1704, index (row)=0 ("index"), length (row)=w1703) -> (w1702:dbl[][])  [unwired: 2 in]
                                n1189 = Build Array (concatenate)(w1702, w1698, w1701) -> (w1697:dbl[][])
                              }
                            }
                          }
                        }
                        n1190 = Array Size(array=w1632) -> (size(s)=w1631:i32[])
                        n1191 = Index Array(array=w1631, index=0) -> (element=w1629:i32)
                        n1192 = Greater?(x=w1629, y=w1628) -> (0:w1627:bool)
                      }
                      n1193 = local write "Numeric"(w1613) -> ()
                      "Numeric" <- w1615
                    }
                  }
                }
              }
              n1194 = local write "lineseed1"(w1579) -> ()
            }
            frame Disabled {
            }
          }
        }
        frame #7 {
          n1195 = disable-structure shown="Enabled" {
            frame Enabled {
              n1196 = local read "fitting?"() -> (w1707:bool)
              n1197 = case shown="False" w1707 {
                tunnel: [_ w1714] -> w1706
                frame False {
                }
                frame True {
                  n1198 = local read "lineseed0"() -> (w1771:dbl[][])
                  n1199 = local read "lineseed1"() -> (w1778:dbl[][])
                  n1200 = local read "lineseed1"() -> (w1762:dbl[][])
                  n1201 = Index Array(array=w1778, index (col)=1 ("disabled index (col)")) -> (element=w1776:dbl[])  [unwired: 1 in]
                  n1202 = Index Array(array=w1762, index (col)=0 ("disabled index (col)")) -> (element=w1760:dbl[])  [unwired: 1 in]
                  n1203 = Array Max & Min(array=w1776) -> (min value=w1711:dbl)  [unwired: 3 out]
                  n1204 = Max & Min(x=w1711, y=0.15) -> (min(x,y)=w1708:dbl)  [unwired: 1 out]
                  n1205 = Subtract(x=w1711, y=0.075) -> (x-y=w1709:dbl)
                  n1206 = Max & Min(x=w1708, y=w1709) -> (max(x,y)=w1713:dbl)  [unwired: 1 out]
                  n1207 = Index Array(array=w1771, index (col)=1 ("disabled index (col)")) -> (element=w1774:dbl[])  [unwired: 1 in]
                  n1208 = Greater Or Equal?(x=w1774, y=w1713) -> (x >= y?=w1773:bool[])
                  n1209 = Boolean To (0,1)(Boolean=w1773) -> (0, 1=w1772:i16[])
                  n1210 = Add Array Elements(numeric array=w1772) -> (sum=w1770:i16)
                  n1211 = Array Subset(array=w1771, index (row)=0 ("index"), length (row)=w1770) -> (w1768:dbl[][])  [unwired: 2 in]
                  n1212 = Index Array(array=w1768, index (col) #1=0 ("disabled index (col)")) -> (element #1=w1765:dbl[], element #2=w1766:dbl[])  [unwired: 3 in]
                  n1213 = Build Cluster Array(w1765, w1766) -> (w1764:cluster{dbl, dbl}[])
                  n1214 = Sort 1D Array(array=w1764) -> (sorted array=w1763:cluster{dbl, dbl}[])
                  n1215 = for {
                    tunnel: w1763 -> [w1832] mode=indexing
                    tunnel: [w1830] -> w1759 mode=indexing
                    tunnel: [w1829] -> w1753 mode=indexing
                    n1216 = Unbundle(w1832) -> (w1829:dbl, w1831:dbl)
                    n1217 = Build Array(w1829, w1831) -> (w1830:dbl[])
                  }
                  n1218 = Array Max & Min(array=w1760) -> (max value=w1755:dbl, min value=w1754:dbl)  [unwired: 2 out]
                  n1219 = Greater Or Equal?(x=w1755, y=w1753) -> (x >= y?=w1752:bool[])
                  n1220 = Greater Or Equal?(x=w1753, y=w1754) -> (x >= y?=w1751:bool[])
                  n1221 = And(x=w1752, y=w1751) -> (x .and. y?=w1750:bool[])
                  n1222 = Boolean To (0,1)(Boolean=w1750) -> (0, 1=w1756:i16[])
                  n1223 = Add Array Elements(numeric array=w1756) -> (sum=w1757:i16)
                  n1224 = Array Max & Min(array=w1756) -> (max index (indices)=w1758:i32)  [unwired: 3 out]
                  n1225 = Array Subset(array=w1759, index (row)=w1758, length (row)=w1757) -> (w1746:dbl[][])  [unwired: 2 in]
                  n1226 = Index Array(array=w1746, index (col)=1 ("disabled index (col)")) -> (element=w1748:dbl[])  [unwired: 1 in]
                  n1227 = Multiply(x=w1748, y=0.0) -> (x*y=w1739:dbl[])
                  n1228 = Array Size(array=w1739) -> (size(s)=w1738:i32)
                  n1229 = Insert Into Array(array=w1746, index (col)=2 ("disabled index (col)"), new element #1=w1739, new element #2=w1739) -> (w1744:dbl[][])  [unwired: 1 in]
                  n1230 = Decrement(x=w1738) -> (x-1=w1734:i32)
                  n1231 = Replace Array Subset(array=w1744, new element #1=1.0 ("new element/subarray"), index (row) #1=0 ("index (row)"), index (col) #1=2 ("disabled index (col)"), new element #2=1.0 ("new element/subarray"), index (row) #2=w1734, index (col) #2=3 ("index (col)")) -> (w1736:dbl[][])
                  n1232 = for {
                    N: w1734 -> [w1793]
                    shift-right: [w1794] -> w1730
                    shift-left: w1736 -> [w1806]
                    shift-right: [w1804] -> _
                    shift-left: 0 -> [w1812]
                    shift-right: [w1795] -> _
                    shift-left: w1734 -> [w1803]
                    i -> [w1791]
                    n1233 = Decrement(x=w1793) -> (x-1=w1792:i32)
                    n1234 = Index Array(array=w1806, index (col)=0 ("disabled index (col)")) -> (element=w1813:dbl[])  [unwired: 1 in]
                    n1235 = Subtract(x=w1792, y=w1791) -> (x-y=w1790:i32)
                    n1236 = Increment(x=w1791) -> (x+1=w1805:i32)
                    n1237 = local read "min lane width"() -> (w1798:dbl)
                    n1238 = Index Array(array=w1813, index #1=w1812, index #2=w1805, index #3=w1803, index #4=w1790) -> (element #1=w1811:dbl, element #2=w1810:dbl, element #3=w1802:dbl, element #4=w1801:dbl)
                    n1239 = Subtract(x=w1811, y=w1810) -> (x-y=w1809:dbl)
                    n1240 = Subtract(x=w1802, y=w1801) -> (x-y=w1800:dbl)
                    n1241 = Absolute Value(x=w1809) -> (abs(x)=w1808:dbl)
                    n1242 = Absolute Value(x=w1800) -> (abs(x)=w1799:dbl)
                    n1243 = Greater Or Equal?(x=w1808, y=w1798) -> (x >= y?=w1807:bool)
                    n1244 = Greater Or Equal?(x=w1799, y=w1798) -> (x >= y?=w1796:bool)
                    n1245 = case shown="True" w1807 {
                      tunnel: w1806 -> [w1822 w1828]
                      tunnel: w1805 -> [w1823 w1824]
                      tunnel: [w1822 w1825] -> w1797
                      tunnel: [w1823 w1824] -> w1804
                      frame False {
                      }
                      frame True {
                        n1246 = Replace Array Subset(array=w1828, new element=2.0 ("new element/subarray"), index (row)=w1824, index (col)=2 ("disabled index (col)")) -> (w1825:dbl[][])
                      }
                    }
                    n1247 = case shown="True" w1796 {
                      tunnel: w1797 -> [w1815 w1821]
                      tunnel: w1790 -> [w1816 w1817]
                      tunnel: [w1815 w1818] -> w1794
                      tunnel: [w1816 w1817] -> w1795
                      frame False {
                      }
                      frame True {
                        n1248 = Replace Array Subset(array=w1821, new element=2.0 ("new element/subarray"), index (row)=w1817, index (col)=3 ("disabled index (col)")) -> (w1818:dbl[][])
                      }
                    }
                  }
                  n1249 = Index Array(array=w1730, index (col) #1=2 ("disabled index (col)")) -> (element #1=w1731:dbl[], element #2=w1732:dbl[])  [unwired: 3 in]
                  n1250 = Add(x=w1731, y=w1732) -> (x+y=w1729:dbl[])
                  n1251 = Replace Array Subset(array=w1730, new element=w1729, index (col)=2 ("disabled index (col)")) -> (w1727:dbl[][])  [unwired: 1 in]
                  "output array" <- w1727
                  n1252 = for {
                    tunnel: w1727 -> [w1781] mode=indexing
                    shift-right: [w1780] -> w1725
                    shift-left: dbl[][] [] -> [w1779]
                    n1253 = Index Array(array=w1781, index=2) -> (element=w1784:dbl)
                    n1254 = Greater Or Equal?(x=w1784, y=2.0) -> (x >= y?=w1782:bool)
                    n1255 = case shown="False" w1782 {
                      tunnel: w1781 -> [_ w1789]
                      tunnel: [w1786 w1788] -> w1780
                      tunnel: w1779 -> [w1786 w1787]
                      frame False {
                      }
                      frame True {
                        n1256 = Build Array (concatenate)(w1787, w1789) -> (w1788:dbl[][])
                      }
                    }
                  }
                  n1257 = Array Subset(array=w1725, index (col)=0 ("index"), length (col)=3 ("length")) -> (w1717:dbl[][])  [unwired: 2 in]
                  n1258 = Index Array(array=w1717, index (col)=2 ("disabled index (col)")) -> (element=w1721:dbl[])  [unwired: 1 in]
                  n1259 = Equal?(x=w1721, y=4.0) -> (x = y?=w1719:bool[])
                  n1260 = Boolean To (0,1)(Boolean=w1719) -> (0, 1=w1718:i16[])
                  n1261 = To Double Precision Float(number=w1718) -> (double precision float=w1715:dbl[])
                  n1262 = Replace Array Subset(array=w1717, new element=w1715, index (col)=2 ("disabled index (col)")) -> (w1714:dbl[][])  [unwired: 1 in]
                }
              }
              "lineseed2" <- w1706
            }
            frame Disabled {
            }
          }
        }
        frame #8 {
          n1263 = disable-structure shown="Enabled" {
            frame Enabled {
              n1264 = local read "fitting?"() -> (w1833:bool)
              n1265 = case shown="True" w1833 {
                frame False {
                }
                frame True {
                  w1839 = 1 ("disabled index (col)")
                  n1266 = local read "lineseed2"() -> (w1854:dbl[][])
                  n1267 = local read "lineseed2"() -> (w1859:dbl[][])
                  n1268 = local read "b"() -> (w1852:dbl)
                  n1269 = Greater Than 0?(x=w1852) -> (x > 0?=w1851:bool)
                  n1270 = disable-structure shown="Enabled" {
                    disable-tunnel: w1859 -> [w1974 _]
                    frame Disabled {
                      n1271 = for {
                        tunnel: w1974 -> [w2052] mode=indexing
                        shift-right: [w2051] -> w1976
                        shift-left: dbl[][] [] -> [w2050]
                        n1272 = Index Array(array=w2052, index=2) -> (element=w2054:dbl)
                        n1273 = Not Equal To 0?(x=w2054) -> (x != 0?=w2053:bool)
                        n1274 = case shown="False" w2053 {
                          tunnel: w2052 -> [_ w2059]
                          tunnel: [w2056 w2058] -> w2051
                          tunnel: w2050 -> [w2056 w2057]
                          frame False {
                          }
                          frame True {
                            n1275 = Build Array (concatenate)(w2057, w2059) -> (w2058:dbl[][])
                          }
                        }
                      }
                      n1276 = Array Size(array=w1976) -> (size(s)=w1984:i32[])
                      n1277 = Index Array(array=w1984, index=0) -> (element=w1978:i32)
                      n1278 = Quotient & Remainder(x=w1978, y=2) -> (x-y*floor(x/y)=w1981:i32, floor(x/y)=w1977:i32)
                      n1279 = Index Array(array=w1976, index (row)=w1977) -> (element=w1975:dbl[])  [unwired: 1 in]
                      n1280 = Equal?(x=1, y=w1981) -> (x = y?=w1979:bool)
                      n1281 = case shown="True" w1979 {
                        tunnel: w1975 -> [_ w2031]
                        frame False {
                        }
                        frame True {
                          n1282 = Index Array(array=w2031, index=0) -> (element=w1989:dbl)
                          n1283 = local read "lane_resol"() -> (w2024:dbl)
                          n1284 = local read "lineseed2"() -> (w1992:dbl[][])
                          n1285 = local read "t2x"() -> (w2023:dbl)
                          n1286 = local read "xt"() -> (w2022:dbl[])
                          n1287 = local read "rdi"() -> (w2029:dbl[])
                          n1288 = Multiply(x=w2023, y=w2022) -> (x*y=w2020:dbl[])
                          n1289 = local read "min lane length"() -> (w1998:dbl)
                          n1290 = Subtract(x=w2029, y=w1989) -> (x-y=w2028:dbl[])
                          n1291 = Index Array(array=w1992, index (col)=0 ("disabled index (col)")) -> (element=w1990:dbl[])  [unwired: 1 in]
                          n1292 = Equal?(x=w1989, y=w1990) -> (x = y?=w1988:bool[])
                          n1293 = Absolute Value(x=w2028) -> (abs(x)=w2026:dbl[])
                          n1294 = Multiply(x=w1998, y=2.0) -> (x*y=w1994:dbl)
                          n1295 = local read "cta"() -> (w2027:dbl)
                          n1296 = Boolean To (0,1)(Boolean=w1988) -> (0, 1=w1987:i16[])
                          n1297 = Multiply(x=w2027, y=w2026) -> (x*y=w2025:dbl[])
                          n1298 = Array Max & Min(array=w1987) -> (max index (indices)=w1986:i32)  [unwired: 3 out]
                          n1299 = Less?(x=w2025, y=w2024) -> (x < y?=w2021:bool[])
                          n1300 = Boolean To (0,1)(Boolean=w2021) -> (0, 1=w2015:i16[])
                          n1301 = Add Array Elements(numeric array=w2015) -> (sum=w2014:i16)
                          n1302 = Build Cluster Array(w2015, w2020) -> (w2019:cluster{i16, dbl}[])
                          n1303 = Sort 1D Array(array=w2019) -> (sorted array=w2018:cluster{i16, dbl}[])
                          n1304 = Reverse 1D Array(array=w2018) -> (reversed array=w2017:cluster{i16, dbl}[])
                          n1305 = for {
                            tunnel: w2017 -> [w2049] mode=indexing
                            tunnel: [w2048] -> w2016 mode=indexing
                            n1306 = Unbundle(w2049) -> (w2048:dbl)  [unwired: 1 out]
                          }
                          n1307 = Array Subset(array=w2016, index=0, length=w2014) -> (w2012:dbl[])
                          n1308 = Multiply(x=w2012, y=2.0) -> (x*y=w2010:dbl[])
                          n1309 = Round To Nearest(number=w2010) -> (nearest integer value=w2009:dbl[])
                          n1310 = Sort 1D Array(array=w2009) -> (sorted array=w2008:dbl[])
                          n1311 = for {
                            tunnel: w2008 -> [w2039] mode=indexing
                            shift-right: [w2040] -> _
                            shift-left: -inf -> [w2042]
                            shift-right: [w2038] -> w2001
                            shift-left: dbl[] [] -> [w2037]
                            n1312 = Not Equal?(x=w2042, y=w2039) -> (x != y?=w2041:bool)
                            n1313 = case shown="True" w2041 {
                              tunnel: [w2044 w2047] -> w2040
                              tunnel: w2039 -> [w2044 w2047]
                              tunnel: [w2043 w2046] -> w2038
                              tunnel: w2037 -> [w2043 w2045]
                              frame False {
                              }
                              frame True {
                                n1314 = Build Array (concatenate)(w2045, w2047) -> (w2046:dbl[])
                              }
                            }
                          }
                          n1315 = Array Size(array=w2001) -> (size(s)=w2003:i32)
                          n1316 = Array Subset(array=w2001, index=1) -> (w2000:dbl[])  [unwired: 1 in]
                          n1317 = Decrement(x=w2003) -> (x-1=w2002:i32)
                          n1318 = Array Subset(array=w2001, index=0, length=w2002) -> (w1999:dbl[])
                          n1319 = Subtract(x=w2000, y=w1999) -> (x-y=w1996:dbl[])
                          n1320 = Array Max & Min(array=w1996) -> (max value=w1995:dbl)  [unwired: 3 out]
                          n1321 = Less?(x=w1995, y=w1994) -> (x < y?=w1993:bool)
                          n1322 = case shown="True" w1993 {
                            tunnel: w1986 -> [_ w2035]
                            frame False {
                            }
                            frame True {
                              n1323 = local read "lineseed2"() -> (w2036:dbl[][])
                              n1324 = Replace Array Subset(array=w2036, new element=2.0 ("new element/subarray"), index (row)=w2035, index (col)=2 ("disabled index (col)")) -> (w2032:dbl[][])
                              n1325 = local write "lineseed2"(w2032) -> ()
                            }
                          }
                        }
                      }
                    }
                    frame Enabled {
                    }
                  }
                  n1326 = Index Array(array=w1859, index (col)=0 ("disabled index (col)")) -> (element=w1844:dbl[])  [unwired: 1 in]
                  n1327 = Array Size(array=w1844) -> (size(s)=w1843:i32)
                  n1328 = Less Than 0?(x=w1844) -> (x < 0?=w1857:bool[])
                  n1329 = Boolean To (0,1)(Boolean=w1857) -> (0, 1=w1856:i16[])
                  n1330 = Subtract(x=w1843, y=1) -> (x-y=w1840:i32)
                  n1331 = Add Array Elements(numeric array=w1856) -> (sum=w1846:i16)
                  n1332 = Max & Min(x=i16 1, y=w1846) -> (max(x,y)=w1841:i16)  [unwired: 1 out]
                  n1333 = Max & Min(x=w1841, y=w1840) -> (min(x,y)=w1837:i32)  [unwired: 1 out]
                  "mylane" <- w1837
                  n1334 = Decrement(x=w1837) -> (x-1=w1838:i32)
                  n1335 = Index Array(array=w1854, index (row) #1=w1838, index (col) #1=0 ("disabled index (col)"), index (row) #2=w1837, index (col) #2=0 ("index (col)"), index (row) #3=w1838, index (col) #3=w1839, index (row) #4=w1837, index (col) #4=w1839) -> (element #1=w1850:dbl, element #2=w1849:dbl, element #3=w1836:dbl, element #4=w1835:dbl)
                  n1336 = case shown="True" w1851 {
                    tunnel: [w1969 w1970] -> w1847
                    tunnel: w1850 -> [w1969 w1973]
                    tunnel: [w1968 w1972] -> w1848
                    tunnel: w1849 -> [w1968 w1971]
                    frame False {
                    }
                    frame True {
                      n1337 = Negate(x=w1973) -> (-x=w1972:dbl)
                      n1338 = Negate(x=w1971) -> (-x=w1970:dbl)
                    }
                  }
                  n1339 = Add(x=w1836, y=w1835) -> (x+y=→"cost":dbl)
                  n1340 = flat-sequence {
                    tunnel: w1848 -> [w1861]
                    tunnel: w1847 -> [w1860]
                    frame #0 {
                      n1341 = Add(x=w1861, y=w1860) -> (x+y=w1864:dbl)
                      n1342 = Multiply(x=w1864, y=0.5) -> (x*y=→"lane shift":dbl)
                      "lane right" <- w1860
                      "lane left" <- w1861
                    }
                    frame #1 {
                      n1343 = disable-structure shown="Enabled" {
                        frame Enabled {
                          n1344 = local read "D_threshold"() -> (w1875:dbl)
                          n1345 = local read "lane right"() -> (w1877:dbl)
                          n1346 = local read "lane left"() -> (w1878:dbl)
                          n1347 = local read "min lane width"() -> (w1876:dbl)
                          n1348 = Subtract(x=w1878, y=w1877) -> (x-y=w1870:dbl)
                          n1349 = Add(x=w1876, y=w1875) -> (x+y=w1874:dbl)
                          n1350 = Greater?(x=8.0 ("y"), y=w1870) -> (0:w1865:bool)
                          n1351 = Multiply(x=w1874, y=2.0) -> (x*y=w1872:dbl)
                          n1352 = Greater?(x=w1870, y=w1872) -> (0:w1866:bool)
                          n1353 = And(x=w1866, y=w1865) -> (x .and. y?=w1869:bool)
                          n1354 = And(x=w1869, y="predict") -> (x .and. y?=w1867:bool)
                          n1355 = case shown="True" w1867 {
                            tunnel: w1870 -> [_ w1895]
                            frame False {
                              n1356 = disable-structure shown="Enabled" {
                                frame Disabled {
                                n1357 = local read "lane right"() -> (w1884:dbl)
                                n1358 = local read "lane left"() -> (w1883:dbl)
                                n1359 = Absolute Value(x=w1883) -> (abs(x)=w1882:dbl)
                                n1360 = Absolute Value(x=w1884) -> (abs(x)=w1880:dbl)
                                n1361 = Max & Min(x=w1882, y=w1880) -> (min(x,y)=w1881:dbl)  [unwired: 1 out]
                                n1362 = Equal?(x=w1881, y=w1880) -> (x = y?=w1879:bool)
                                n1363 = case shown="True" w1879 {
                                frame False {
                                }
                                frame True {
                                n1364 = global read "G_PATH.vi" "lane_width"() -> (w1885:dbl)
                                n1365 = local read "lane right"() -> (w1888:dbl)
                                n1366 = Add(x=w1888, y=0.1) -> (x+y=w1886:dbl)
                                n1367 = local write "lane right"(w1886) -> ()
                                n1368 = Add(x=w1886, y=w1885) -> (x+y=w1892:dbl)
                                n1369 = Subtract(x=w1892, y=-0.1) -> (x-y=w1894:dbl)
                                n1370 = local write "lane left"(w1894) -> ()
                                n1371 = Add(x=w1886, y=w1894) -> (x+y=w1890:dbl)
                                n1372 = Multiply(x=w1890, y=0.5) -> (x*y=w1891:dbl)
                                n1373 = local write "lane shift"(w1891) -> ()
                                }
                                }
                                }
                                frame Enabled {
                                }
                              }
                            }
                            frame True {
                              n1374 = disable-structure shown="Enabled" {
                                disable-tunnel: w1895 -> [w1907 w1920]
                                frame Disabled {
                                n1375 = Multiply(x=w1907, y=0.5) -> (x*y=w1905:dbl)
                                n1376 = global read "G_PATH.vi" "lanewidth"() -> (w1903)
                                n1377 = local read "lane right"() -> (w1898:dbl)
                                n1378 = Max & Min(x=w1903, y=3.0) -> (max(x,y)=w1902:dbl)  [unwired: 1 out]
                                n1379 = Max & Min(x=w1905, y=w1902) -> (min(x,y)=w1904:dbl)  [unwired: 1 out]
                                n1380 = Add(x=w1898, y=w1904) -> (x+y=w1897:dbl)
                                n1381 = local write "lane left"(w1897) -> ()
                                n1382 = Add(x=w1898, y=w1897) -> (x+y=w1899:dbl)
                                n1383 = Multiply(x=w1899, y=0.5) -> (x*y=w1896:dbl)
                                n1384 = local write "lane shift"(w1896) -> ()
                                }
                                frame Enabled {
                                n1385 = Multiply(x=w1920, y=0.5) -> (x*y=w1910:dbl)
                                n1386 = local read "D_threshold"() -> (w1940:dbl)
                                n1387 = global read "G_PATH.vi" "lane_width"() -> (w1948:dbl)
                                n1388 = local read "lane right"() -> (w1913:dbl)
                                n1389 = local read "lineseed0"() -> (w1937:dbl[][])
                                n1390 = local read "b"() -> (w1926:dbl)
                                n1391 = local read "b"() -> (w1949:dbl)
                                n1392 = Greater Than 0?(x=w1926) -> (x > 0?=w1925:bool)
                                n1393 = Greater Than 0?(x=w1949) -> (x > 0?=w1918:bool)
                                n1394 = Max & Min(x=3.2, y=w1910) -> (min(x,y)=w1909:dbl)  [unwired: 1 out]
                                n1395 = case shown="True" w1918 {
                                tunnel: [w1950 w1959] -> w1917
                                frame True {
                                n1396 = local read "lineseed0"() -> (w1957:dbl[][])
                                n1397 = Index Array(array=w1957, index (col)=0 ("index (row)")) -> (element=w1951:dbl[])  [unwired: 1 in]
                                n1398 = Less Than 0?(x=w1951) -> (x < 0?=w1956:bool[])
                                n1399 = Boolean To (0,1)(Boolean=w1956) -> (0, 1=w1955:i16[])
                                n1400 = To Double Precision Float(number=w1955) -> (double precision float=w1954:dbl[])
                                n1401 = Multiply(x=w1954, y=-100.0) -> (x*y=w1952:dbl[])
                                n1402 = Add(x=w1952, y=w1951) -> (x+y=w1950:dbl[])
                                }
                                frame False {
                                n1403 = local read "lineseed0"() -> (w1966:dbl[][])
                                n1404 = Index Array(array=w1966, index (col)=0 ("index (row)")) -> (element=w1960:dbl[])  [unwired: 1 in]
                                n1405 = Greater Than 0?(x=w1960) -> (x > 0?=w1965:bool[])
                                n1406 = Boolean To (0,1)(Boolean=w1965) -> (0, 1=w1964:i16[])
                                n1407 = To Double Precision Float(number=w1964) -> (double precision float=w1963:dbl[])
                                n1408 = Multiply(x=w1963, y=100.0) -> (x*y=w1961:dbl[])
                                n1409 = Add(x=w1961, y=w1960) -> (x+y=w1959:dbl[])
                                }
                                }
                                n1410 = Multiply(x=w1940, y=2.0) -> (x*y=w1939:dbl)
                                n1411 = Multiply(x=w1948, y=-0.5) -> (x*y=w1945:dbl)
                                n1412 = Negate(x=w1945) -> (-x=w1946:dbl)
                                n1413 = Select(t=w1946, s=w1918, f=w1945) -> (s? t:f=w1944:dbl)
                                n1414 = Subtract(x=w1917, y=w1944) -> (x-y=w1943:dbl[])
                                n1415 = Absolute Value(x=w1943) -> (abs(x)=w1942:dbl[])
                                n1416 = Array Max & Min(array=w1942) -> (min value=w1938:dbl, min index (indices)=w1936:i32)  [unwired: 2 out]
                                n1417 = Less?(x=w1938, y=w1939) -> (x < y?=w1933:bool)
                                n1418 = Index Array(array=w1937, index (row)=w1936) -> (element=w1932:dbl[])  [unwired: 1 in]
                                n1419 = Index Array(array=w1932, index #1=0 ("index")) -> (element #1=w1923:dbl, element #2=w1930:dbl)  [unwired: 1 in]
                                n1420 = Negate(x=w1923) -> (-x=w1924:dbl)
                                n1421 = Greater?(x=w1930, y=0.15) -> (0:w1934:bool)
                                n1422 = And(x=w1934, y=w1933) -> ()  [unwired: 1 out]
                                n1423 = Select(t=w1924, s=w1925, f=w1923) -> (s? t:f=w1912:dbl)
                                n1424 = Max & Min(x=w1912, y=w1913) -> (max(x,y)=w1911:dbl)  [unwired: 1 out]
                                n1425 = Add(x=w1911, y=0.1) -> (x+y=w1922:dbl)
                                n1426 = local write "lane right"(w1922) -> ()
                                n1427 = Add(x=w1922, y=w1909) -> (x+y=w1916:dbl)
                                n1428 = Subtract(x=w1916, y=-0.1) -> (x-y=w1914:dbl)
                                n1429 = local write "lane left"(w1914) -> ()
                                n1430 = Add(x=w1922, y=w1914) -> (x+y=w1928:dbl)
                                n1431 = Multiply(x=w1928, y=0.5) -> (x*y=w1927:dbl)
                                n1432 = local write "lane shift"(w1927) -> ()
                                }
                              }
                            }
                          }
                        }
                        frame Disabled {
                        }
                      }
                    }
                  }
                }
              }
            }
            frame Disabled {
            }
          }
        }
        frame #9 {
          n1433 = disable-structure shown="Enabled" {
            disable-tunnel: [w2072 w2120] -> w2068
            disable-tunnel: [w2081 w2120] -> w2067
            frame Enabled {
              n1434 = disable-structure shown="Enabled" {
                disable-tunnel: [w2092 _] -> w2076
                frame Disabled {
                  n1435 = global read "G_VEH.vi" "xyhc_lane"() -> (w2108:T3)
                  n1436 = local read item#-1() -> (w2105)
                  n1437 = Unbundle By Name(w2105) -> ("lcc[1]"=w2104, "lcc[0]"=w2102)
                  n1438 = Unbundle By Name(w2108) -> ("idx"=w2107:i32, "x"=w2103:dbl, "y"=w2101:dbl)
                  n1439 = Subtract(x=w2103, y=w2104) -> (x-y=w2100:dbl)
                  n1440 = Subtract(x=w2101, y=w2102) -> (x-y=w2099:dbl)
                  n1441 = Square(x=w2100) -> (x^2=w2098:dbl)
                  n1442 = Square(x=w2099) -> (x^2=w2097:dbl)
                  n1443 = Add(x=w2098, y=w2097) -> (x+y=w2096:dbl)
                  n1444 = Equal To 0?(x=w2107) -> (x = 0?=w2106:bool)
                  n1445 = Square Root(x=w2096) -> (sqrt(x)=w2095:dbl)
                  n1446 = Greater?(x=w2095, y=20.0) -> (0:w2093:bool)
                  n1447 = Or(x=w2106, y=w2093) -> (x .or. y?=w2092:bool)
                }
                frame Enabled {
                }
              }
              n1448 = local read "lane right"() -> (w2083:dbl)
              n1449 = local read "lane shift"() -> (w2078:dbl)
              n1450 = local read "lane left"() -> (w2084:dbl)
              n1451 = local read "min lane width"() -> (w2075:dbl)
              n1452 = disable-structure shown="Enabled" {
                disable-tunnel: [w2090 4.0] -> w2080
                disable-tunnel: w2075 -> [w2085 _]
                frame Disabled {
                  n1453 = local read "D_threshold"() -> (w2088:dbl)
                  n1454 = Increment(x=w2085) -> (x+1=w2089:dbl)
                  n1455 = Multiply(x=w2088, y=3.01) -> (x*y=w2086:dbl)
                  n1456 = Add(x=w2089, y=w2086) -> (x+y=w2090:dbl)
                }
                frame Enabled {
                }
              }
              n1457 = Subtract(x=w2084, y=w2083) -> (x-y=w2082:dbl)
              n1458 = Add(x=w2075, y=0.0) -> (x+y=w2074:dbl)
              n1459 = In Range and Coerce(upper limit=w2080, x=w2082, lower limit=w2074) -> (In Range?=w2081:bool)  [unwired: 1 out]
              n1460 = case shown="False" w2076 {
                tunnel: [w2110 w2117] -> w2079
                frame False {
                  n1461 = local read "cost"() -> (w2113:dbl)
                  n1462 = local read "D_threshold"() -> (w2115:dbl)
                  n1463 = global read "G_PATH.vi" "lane_shift"() -> (w2109:dbl)
                  n1464 = Greater?(x=w2113, y=0.2) -> (0:w2112:bool)
                  n1465 = Multiply(x=w2115, y=3.0) -> (x*y=w2111:dbl)
                  n1466 = Select(t=w2109, s=w2112, f=w2111) -> (s? t:f=w2110:dbl)
                }
                frame True {
                  n1467 = local read "min lane width"() -> (w2119:dbl)
                  n1468 = Multiply(x=w2119, y=0.5) -> (x*y=w2117:dbl)
                }
              }
              n1469 = Absolute Value(x=w2078) -> (abs(x)=w2077:dbl)
              n1470 = Less Or Equal?(x=w2077, y=w2079) -> (x <= y?=w2072:bool)
            }
            frame Disabled {
              w2120 = TRUE
            }
          }
          n1471 = local read "rd0"() -> (w2065:dbl)
          n1472 = local read "maxradius"() -> (w2063:dbl)
          n1473 = local read "lineseed2"() -> (w2071:dbl[][])
          n1474 = local read "fitting?"() -> (w2061:bool)
          n1475 = Empty Array?(array=w2071) -> (empty?=w2070:bool)
          n1476 = Greater?(x=w2065, y=w2063) -> (0:w2064:bool)
          n1477 = Equal To 0?(x=w2065) -> (x = 0?=w2066:bool)
          n1478 = Or(x=w2066, y=w2064) -> (x .or. y?=w2062:bool)
          n1479 = Not(x=w2070) -> (.not. x?=w2060:bool)
          n1480 = Compound Arithmetic op=AND(w2060, w2068, w2067, w2062, w2061) -> (w2069:bool)
          n1481 = case shown="True" w2069 {
            frame False {
              n1482 = local read "RXY"() -> (w2125:dbl[])
              n1483 = Index Array(array=w2125, index=0) -> (element=w2121:dbl)
              n1484 = Less?(x=w2121, y=50.0) -> (x < y?=w2122:bool)
              n1485 = case shown="False" w2122 {
                tunnel: w2121 -> [w2127 _]
                frame False {
                  n1486 = Less?(x=w2127, y=500.0) -> (x < y?=w2126:bool)
                  n1487 = case shown="True" w2126 {
                    frame False {
                      n1488 = global read "G_PATH.vi" "lane_shift"() -> (w2131:dbl)
                      n1489 = Less?(x=w2131, y=0.6 ("lane_shift")) -> (x < y?=w2129:bool)
                      n1490 = case shown="True" w2129 {
                        frame False {
                        }
                        frame True {
                          n1491 = global write "G_PATH.vi" "lane_shift"(0.6 ("lane_shift")) -> ()
                        }
                      }
                    }
                    frame True {
                      n1492 = global read "G_VEH.vi" "candata"() -> (w2136:T4)
                      n1493 = Unbundle By Name(w2136) -> ("VS_can"=w2135:dbl)
                      n1494 = Less?(x=w2135, y=5.0) -> (x < y?=w2133:bool)
                      n1495 = case shown="True" w2133 {
                        frame True {
                          n1496 = global read "G_PATH.vi" "lane_shift"() -> (w2139:dbl)
                          n1497 = Less?(x=w2139, y=1.0 ("lane_shift")) -> (x < y?=w2137:bool)
                          n1498 = case shown="True" w2137 {
                            frame False {
                            }
                            frame True {
                              n1499 = global write "G_PATH.vi" "lane_shift"(1.0 ("lane_shift")) -> ()
                            }
                          }
                        }
                        frame False {
                          n1500 = global read "G_PATH.vi" "lane_shift"() -> (w2143:dbl)
                          n1501 = Less?(x=w2143, y=0.625 ("lane_shift")) -> (x < y?=w2141:bool)
                          n1502 = case shown="True" w2141 {
                            frame False {
                            }
                            frame True {
                              n1503 = global write "G_PATH.vi" "lane_shift"(0.625 ("lane_shift")) -> ()
                            }
                          }
                        }
                      }
                    }
                  }
                }
                frame True {
                  n1504 = global write "G_PATH.vi" "lane_shift"(1.75 ("lane_shift")) -> ()
                }
              }
            }
            frame True {
              n1505 = flat-sequence {
                frame #0 {
                  n1506 = local read "lane right"() -> (w2149:dbl)
                  n1507 = local read "lane left"() -> (w2150:dbl)
                  n1508 = Subtract(x=w2150, y=w2149) -> (x-y=w2148:dbl)
                  n1509 = disable-structure shown="Enabled" {
                    disable-tunnel: w2148 -> [w2152 _]
                    disable-tunnel: [w2151 TRUE] -> w2147
                    frame Enabled {
                      n1510 = global read "G_PATH.vi" "lane_width"() -> (w2153:dbl)
                      n1511 = Less Or Equal?(x=w2152, y=w2153) -> (x <= y?=w2151:bool)
                    }
                    frame Disabled {
                    }
                  }
                  n1512 = case shown="False" w2147 {
                    frame False {
                      n1513 = disable-structure shown="Enabled" {
                        frame Disabled {
                          n1514 = flat-sequence {
                            frame #0 {
                              n1515 = global read "G_PATH.vi" "lanewidth"() -> (w2169)
                              n1516 = global read "G_PATH.vi" "lanewidth"() -> (w2180)
                              n1517 = local read "lane right"() -> (w2168:dbl)
                              n1518 = local read "lane shift"() -> (w2167:dbl)
                              n1519 = local read "lane shift"() -> (w2181:dbl)
                              n1520 = local read "lane left"() -> (w2182:dbl)
                              n1521 = Subtract(x=w2167, y=w2168) -> (x-y=w2155:dbl)
                              n1522 = Subtract(x=w2182, y=w2181) -> (x-y=w2163:dbl)
                              n1523 = Multiply(x=w2169, y=0.5) -> (x*y=w2159:dbl)
                              n1524 = Multiply(x=w2180, y=0.5) -> (x*y=w2165:dbl)
                              n1525 = Greater?(x=w2155, y=w2159) -> (0:w2171:bool)
                              n1526 = Greater?(x=w2163, y=w2165) -> (0:w2178:bool)
                              n1527 = Multiply(x=w2155, y=0.01) -> (x*y=w2157:dbl)
                              n1528 = Multiply(x=w2159, y=0.99) -> (x*y=w2158:dbl)
                              n1529 = Multiply(x=w2163, y=0.02) -> (x*y=w2162:dbl)
                              n1530 = Multiply(x=w2165, y=0.98) -> (x*y=w2161:dbl)
                              n1531 = Add(x=w2157, y=w2158) -> (x+y=w2173:dbl)
                              n1532 = Add(x=w2162, y=w2161) -> (x+y=w2176:dbl)
                              n1533 = Multiply(x=w2173, y=1.0) -> (x*y=w2174:dbl)
                              n1534 = Multiply(x=w2176, y=1.0) -> (x*y=w2175:dbl)
                              n1535 = case shown="True" w2171 {
                                tunnel: w2174 -> [_ w2184]
                                frame False {
                                }
                                frame True {
                                n1536 = local read "lane shift"() -> (w2185:dbl)
                                n1537 = Subtract(x=w2185, y=w2184) -> (x-y=w2183:dbl)
                                n1538 = local write "lane right"(w2183) -> ()
                                }
                              }
                              n1539 = case shown="True" w2178 {
                                tunnel: w2175 -> [_ w2187]
                                frame False {
                                }
                                frame True {
                                n1540 = local read "lane shift"() -> (w2188:dbl)
                                n1541 = Add(x=w2187, y=w2188) -> (x+y=w2186:dbl)
                                n1542 = local write "lane left"(w2186) -> ()
                                }
                              }
                            }
                            frame #1 {
                              n1543 = local read "lane right"() -> (w2192:dbl)
                              n1544 = local read "lane left"() -> (w2193:dbl)
                              n1545 = Add(x=w2193, y=w2192) -> (x+y=w2191:dbl)
                              n1546 = Subtract(x=w2193, y=w2192) -> (x-y=w2194:dbl)
                              n1547 = global write "G_PATH.vi" "lanewidth"(w2194) -> ()
                              n1548 = Multiply(x=0.5, y=w2191) -> (x*y=w2189:dbl)
                              n1549 = local write "lane shift"(w2189) -> ()
                            }
                          }
                        }
                        frame Enabled {
                          n1550 = flat-sequence {
                            frame #0 {
                              n1551 = global read "G_PATH.vi" "lane_width"() -> (w2198:dbl)
                              n1552 = global read "G_PATH.vi" "lane_width"() -> (w2205:dbl)
                              n1553 = local read "lane right"() -> (w2196:dbl)
                              n1554 = local read "lane left"() -> (w2202:dbl)
                              n1555 = Absolute Value(x=w2196) -> (abs(x)=w2195:dbl)
                              n1556 = Multiply(x=w2198, y=0.5) -> (x*y=w2200:dbl)
                              n1557 = Multiply(x=w2205, y=0.5) -> (x*y=w2203:dbl)
                              n1558 = Greater?(x=w2195, y=w2200) -> (0:w2197:bool)
                              n1559 = Greater?(x=w2202, y=w2203) -> (0:w2201:bool)
                              n1560 = case shown="True" w2197 {
                                frame False {
                                }
                                frame True {
                                n1561 = global read "G_PATH.vi" "lane_width"() -> (w2254:dbl)
                                n1562 = local read "lineseed0"() -> (w2258:dbl[][])
                                n1563 = local read "b"() -> (w2252:dbl)
                                n1564 = Greater Than 0?(x=w2252) -> (x > 0?=w2255:bool)
                                n1565 = Index Array(array=w2258, index (col) #1=0 ("index (row)")) -> (element #1=w2268:dbl[], element #2=w2263:dbl[])  [unwired: 3 in]
                                n1566 = Multiply(x=w2254, y=-0.5) -> (x*y=w2256:dbl)
                                n1567 = Negate(x=w2256) -> (-x=w2257:dbl)
                                n1568 = Select(t=w2257, s=w2255, f=w2256) -> (s? t:f=w2260:dbl)
                                n1569 = Subtract(x=w2268, y=w2260) -> (x-y=w2261:dbl[])
                                n1570 = Absolute Value(x=w2261) -> (abs(x)=w2262:dbl[])
                                n1571 = Array Max & Min(array=w2262) -> (min index (indices)=w2267:i32)  [unwired: 3 out]
                                n1572 = Index Array(array=w2268, index=w2267) -> (element=w2269:dbl)
                                n1573 = Index Array(array=w2263, index=w2267) -> (element=w2264:dbl)
                                n1574 = Greater?(x=w2264, y=0.11) -> (0:w2266:bool)
                                n1575 = case shown="True" w2266 {
                                tunnel: w2269 -> [_ w2271]
                                frame False {
                                }
                                frame True {
                                n1576 = Negate(x=w2271) -> (-x=w2272:dbl)
                                n1577 = local read "b"() -> (w2274:dbl)
                                n1578 = Greater Than 0?(x=w2274) -> (x > 0?=w2273:bool)
                                n1579 = Select(t=w2272, s=w2273, f=w2271) -> (s? t:f=w2270:dbl)
                                n1580 = local write "lane right"(w2270) -> ()
                                }
                                }
                                }
                              }
                              n1581 = case shown="True" w2201 {
                                frame False {
                                }
                                frame True {
                                n1582 = global read "G_PATH.vi" "lane_width"() -> (w2222:dbl)
                                n1583 = local read "b"() -> (w2224:dbl)
                                n1584 = Greater Than 0?(x=w2224) -> (x > 0?=w2206:bool)
                                n1585 = case shown="False" w2206 {
                                tunnel: [w2232 w2243] -> w2219
                                frame True {
                                n1586 = local read "lineseed0"() -> (w2234:dbl[][])
                                n1587 = Index Array(array=w2234, index (col)=0 ("index (row)")) -> (element=w2226:dbl[])  [unwired: 1 in]
                                n1588 = Greater Than 0?(x=w2226) -> (x > 0?=w2231:bool[])
                                n1589 = Boolean To (0,1)(Boolean=w2231) -> (0, 1=w2230:i16[])
                                n1590 = To Double Precision Float(number=w2230) -> (double precision float=w2229:dbl[])
                                n1591 = Multiply(x=w2229, y=100.0) -> (x*y=w2227:dbl[])
                                n1592 = Add(x=w2227, y=w2226) -> (x+y=w2225:dbl[])
                                n1593 = Replace Array Subset(array=w2234, new element=w2225, index (col)=0 ("disabled index (col)")) -> (w2232:dbl[][])  [unwired: 1 in]
                                }
                                frame False {
                                n1594 = local read "lineseed0"() -> (w2245:dbl[][])
                                n1595 = Index Array(array=w2245, index (col)=0 ("index (row)")) -> (element=w2237:dbl[])  [unwired: 1 in]
                                n1596 = Less Than 0?(x=w2237) -> (x < 0?=w2242:bool[])
                                n1597 = Boolean To (0,1)(Boolean=w2242) -> (0, 1=w2241:i16[])
                                n1598 = To Double Precision Float(number=w2241) -> (double precision float=w2240:dbl[])
                                n1599 = Multiply(x=w2240, y=-100.0) -> (x*y=w2238:dbl[])
                                n1600 = Add(x=w2238, y=w2237) -> (x+y=w2236:dbl[])
                                n1601 = Replace Array Subset(array=w2245, new element=w2236, index (col)=0 ("disabled index (col)")) -> (w2243:dbl[][])  [unwired: 1 in]
                                }
                                }
                                n1602 = Multiply(x=w2222, y=0.5) -> (x*y=w2221:dbl)
                                n1603 = Negate(x=w2221) -> (-x=w2220:dbl)
                                n1604 = Select(t=w2220, s=w2206, f=w2221) -> (s? t:f=w2217:dbl)
                                n1605 = Index Array(array=w2219, index (col) #1=0 ("index (row)")) -> (element #1=w2209:dbl[], element #2=w2214:dbl[])  [unwired: 3 in]
                                n1606 = Subtract(x=w2209, y=w2217) -> (x-y=w2216:dbl[])
                                n1607 = Absolute Value(x=w2216) -> (abs(x)=w2215:dbl[])
                                n1608 = Array Max & Min(array=w2215) -> (min value=→"min value":dbl, min index (indices)=w2210:i32)  [unwired: 2 out]
                                n1609 = Index Array(array=w2209, index=w2210) -> (element=w2208:dbl)
                                n1610 = Index Array(array=w2214, index=w2210) -> (element=w2213:dbl)
                                n1611 = Greater?(x=w2213, y=0.11) -> (0:w2211:bool)
                                n1612 = case shown="True" w2211 {
                                tunnel: w2208 -> [_ w2248]
                                frame False {
                                }
                                frame True {
                                n1613 = Negate(x=w2248) -> (-x=w2249:dbl)
                                n1614 = local read "b"() -> (w2251:dbl)
                                n1615 = Greater Than 0?(x=w2251) -> (x > 0?=w2250:bool)
                                n1616 = Select(t=w2249, s=w2250, f=w2248) -> (s? t:f=w2247:dbl)
                                n1617 = local write "lane left"(w2247) -> ()
                                }
                                }
                                }
                              }
                            }
                            frame #1 {
                              n1618 = global read "G_PATH.vi" "lane_width"() -> (w2277:dbl)
                              n1619 = local read "lane left"() -> (w2281:dbl)
                              n1620 = local read "min lane width"() -> (w2279:dbl)
                              n1621 = Multiply(x=w2277, y=0.5) -> (x*y=w2275:dbl)
                              n1622 = Subtract(x=w2281, y=w2275) -> (x-y=w2278:dbl)
                              n1623 = Greater?(x=w2278, y=w2279) -> (0:w2280:bool)
                              n1624 = case shown="True" w2280 {
                                frame False {
                                }
                                frame True {
                                n1625 = local read "lane right"() -> (w2285:dbl)
                                n1626 = local read "lane left"() -> (w2286:dbl)
                                n1627 = Add(x=w2286, y=w2285) -> (x+y=w2284:dbl)
                                n1628 = Multiply(x=w2284, y=0.5) -> (x*y=w2282:dbl)
                                n1629 = local write "lane left"(w2282) -> ()
                                }
                              }
                            }
                            frame #2 {
                              n1630 = disable-structure shown="Enabled" {
                                frame Enabled {
                                n1631 = local read "lane right"() -> (w2291:dbl)
                                n1632 = local read "lane left"() -> (w2287:dbl)
                                n1633 = Add(x=w2287, y=w2291) -> (x+y=w2290:dbl)
                                n1634 = Subtract(x=w2287, y=w2291) -> (x-y=w2292:dbl)
                                n1635 = global write "G_PATH.vi" "lane_width"(w2292) -> ()
                                n1636 = Multiply(x=0.5, y=w2290) -> (x*y=w2288:dbl)
                                n1637 = local write "lane shift"(w2288) -> ()
                                }
                                frame Disabled {
                                }
                              }
                            }
                          }
                        }
                        frame Disabled {
                        }
                      }
                    }
                    frame True {
                    }
                  }
                }
                frame #1 {
                  n1638 = local read "rd0"() -> (→"rd0 2":dbl)
                  n1639 = local read "lane right"() -> (w2299:dbl)
                  n1640 = local read "lane shift"() -> (w2310:dbl)
                  n1641 = local read "lane left"() -> (w2297:dbl)
                  n1642 = local read "b"() -> (w2302:dbl)
                  n1643 = local read "b"() -> (w2294:dbl)
                  n1644 = Greater Than 0?(x=w2302) -> (x > 0?=w2301:bool)
                  n1645 = Greater Than 0?(x=w2294) -> (x > 0?=w2295:bool)
                  n1646 = Negate(x=w2299) -> (-x=w2300:dbl)
                  n1647 = Negate(x=w2297) -> (-x=w2296:dbl)
                  n1648 = local read "rd0"() -> (w2309:dbl)
                  n1649 = Add(x=w2310, y=w2309) -> (x+y=→"center":dbl)
                  n1650 = Select(t=w2300, s=w2301, f=w2299) -> (s? t:f=w2298:dbl)
                  n1651 = Select(t=w2296, s=w2295, f=w2297) -> (s? t:f=w2293:dbl)
                  n1652 = local read "rd0"() -> (w2307:dbl)
                  n1653 = local read "rd0"() -> (w2304:dbl)
                  n1654 = Add(x=w2298, y=w2307) -> (x+y=→"right":dbl)
                  n1655 = Add(x=w2293, y=w2304) -> (x+y=→"left":dbl)
                }
                frame #2 {
                  n1656 = local read "lane right"() -> (w2317:dbl)
                  n1657 = local read "lane left"() -> (w2318:dbl)
                  n1658 = local read "min lane width"() -> (w2313:dbl)
                  n1659 = local read "min lane width"() -> (w2315:dbl)
                  n1660 = Subtract(x=w2318, y=w2317) -> (x-y=w2316:dbl)
                  n1661 = Add(x=1.5, y=w2313) -> (x+y=w2311:dbl)
                  n1662 = In Range and Coerce(upper limit=w2311, x=w2316, lower limit=w2315) -> (In Range?=w2314:bool)  [unwired: 1 out]
                  n1663 = case shown="True" w2314 {
                    frame False {
                    }
                    frame True {
                      n1664 = flat-sequence {
                        frame #0 {
                          n1665 = disable-structure shown="Enabled" {
                            disable-tunnel: [0.2 ("lane_shift") w2352] -> w2321
                            frame Enabled {
                            }
                            frame Disabled {
                              n1666 = local read "lane shift"() -> (w2352:dbl)
                            }
                          }
                          n1667 = local read "M6006"() -> (w2322:T1)
                          n1668 = global read "G_VEH.vi" "xyhc_shift"() -> (w2333:T3)
                          n1669 = Unbundle By Name(w2322) -> ("lcc[1]"=w2324:dbl, "lcc[0]"=w2325:dbl, "attitude[2]"=w2326:dbl)
                          n1670 = local read "lane right"() -> (w2338:dbl)
                          n1671 = local read "lane shift"() -> (w2320:dbl)
                          n1672 = local read "lane left"() -> (w2339:dbl)
                          n1673 = disable-structure shown="Enabled" {
                            disable-tunnel: w2320 -> [w2342 w2350]
                            disable-tunnel: [w2341 w2349] -> w2319
                            frame Disabled {
                              w2346 = 0.75 ("x")
                              n1674 = feedback #1(0.0 ("lane shift")) -> (w2347:dbl)
                              n1675 = feedback-in #1(w2342) -> ()
                              n1676 = Multiply(x=w2346, y=w2347) -> (x*y=w2345:dbl)
                              n1677 = Decrement(x=w2346) -> (x-1=w2343:dbl)
                              n1678 = Multiply(x=w2342, y=w2343) -> (x*y=w2344:dbl)
                              n1679 = Subtract(x=w2344, y=w2345) -> (x-y=w2341:dbl)
                            }
                            frame Enabled {
                              n1680 = Negate(x=w2350) -> (-x=w2349:dbl)
                            }
                          }
                          n1681 = Unbundle By Name(w2333) -> ("idx"=w2334:i32)
                          n1682 = Subtract(x=w2339, y=w2338) -> (x-y=w2340:dbl)
                          n1683 = Negate(x=w2326) -> (-x=w2327:dbl)
                          n1684 = global write "G_PATH.vi" "lane_width"(w2340) -> ()
                          n1685 = Increment(x=w2334) -> (x+1=w2336:i32)
                          n1686 = local read "xyhc"() -> (w2335:T2)
                          n1687 = Bundle By Name(cluster=w2335, "c_idx"=w2336) -> (w2337:T2)
                          n1688 = global write "G_PATH.vi" "lane_shift"(w2321) -> ()
                          n1689 = global write "G_VEH.vi" "xyhc_shift"(w2337) -> ()
                          n1690 = call "rotm_siso.vi"("angle[rad]"=w2327, "reverse"=TRUE, "y0"=w2325, "x0"=w2324, "y"=0.0, "x"=w2319) -> ("y'"=w2331:dbl, "x'"=w2330:dbl)  [unwired: 4 in]
                          n1691 = local read "xyhc"() -> (w2329:T2)
                          n1692 = Bundle By Name(cluster=w2329, "xc"=w2330, "yc"=w2331) -> (w2332:T2)
                          n1693 = global write "G_VEH.vi" "xyhc_lane"(w2332) -> ()
                        }
                        frame #1 {
                          n1694 = local read "mode"() -> (w2353:dbl)
                          n1695 = Equal To 0?(x=w2353) -> (x = 0?=w2354:bool)
                          n1696 = case shown="True" w2354 {
                            frame False {
                              n1697 = local read "M6006"() -> (w2397:T1)
                              n1698 = local read "M6006"() -> (w2372:T1)
                              n1699 = local read "map_track"() -> (w2412:dbl[][])
                              n1700 = Unbundle By Name(w2397) -> ("lcc[1]"=w2401:dbl, "lcc[0]"=w2400:dbl, "attitude[2]"=w2399:dbl)
                              n1701 = local read "map_track"() -> (w2357:dbl[][])
                              n1702 = Unbundle By Name(w2372) -> ("lcc[1]"=w2368:dbl, "lcc[0]"=w2369:dbl, "attitude[2]"=w2370:dbl)
                              n1703 = Negate(x=w2399) -> (-x=w2398:dbl)
                              n1704 = Negate(x=w2370) -> (-x=w2371:dbl)
                              n1705 = Index Array(array=w2412, index (col) #1=0 ("disabled index (col)"), index (col) #2=1 ("index (col)")) -> (element #1=w2410:dbl[], element #2=w2408:dbl[])  [unwired: 2 in]
                              n1706 = Index Array(array=w2357, index (col) #1=0 ("disabled index (col)"), index (col) #2=1 ("index (col)")) -> (element #1=w2359:dbl[], element #2=w2361:dbl[])  [unwired: 2 in]
                              n1707 = local read "b"() -> (w2411:dbl)
                              n1708 = local read "a"() -> (w2409:dbl)
                              n1709 = local read "b"() -> (w2358:dbl)
                              n1710 = local read "a"() -> (w2360:dbl)
                              n1711 = Subtract(x=w2408, y=w2409) -> (x-y=w2406:dbl[])
                              n1712 = Subtract(x=w2361, y=w2360) -> (x-y=w2363:dbl[])
                              n1713 = Subtract(x=w2410, y=w2411) -> (x-y=w2407:dbl[])
                              n1714 = Subtract(x=w2359, y=w2358) -> (x-y=w2362:dbl[])
                              n1715 = Inverse Tangent (2 Input)(1:w2406, 2:w2407) -> (0:w2405:dbl[])
                              n1716 = Inverse Tangent (2 Input)(1:w2363, 2:w2362) -> (0:w2364:dbl[])
                              n1717 = local read "right"() -> (w2403:dbl)
                              n1718 = local read "left"() -> (w2366:dbl)
                              n1719 = Sine & Cosine(0:w2405) -> (1:w2404:dbl[], 2:w2402:dbl[])
                              n1720 = Sine & Cosine(0:w2364) -> (1:w2365:dbl[], 2:w2367:dbl[])
                              n1721 = Multiply(x=w2403, y=w2404) -> (x*y=w2387:dbl[])
                              n1722 = Multiply(x=w2403, y=w2402) -> (x*y=w2390:dbl[])
                              n1723 = Multiply(x=w2366, y=w2365) -> (x*y=w2382:dbl[])
                              n1724 = Multiply(x=w2366, y=w2367) -> (x*y=w2379:dbl[])
                              n1725 = local read "b"() -> (w2388:dbl)
                              n1726 = local read "a"() -> (w2391:dbl)
                              n1727 = local read "b"() -> (w2381:dbl)
                              n1728 = local read "a"() -> (w2378:dbl)
                              n1729 = Add(x=w2390, y=w2391) -> (x+y=w2389:dbl[])
                              n1730 = Add(x=w2379, y=w2378) -> (x+y=w2380:dbl[])
                              n1731 = Add(x=w2388, y=w2387) -> (x+y=w2386:dbl[])
                              n1732 = Add(x=w2381, y=w2382) -> (x+y=w2383:dbl[])
                              n1733 = Negate(x=w2386) -> (-x=w2396:dbl[])
                              n1734 = Negate(x=w2383) -> (-x=w2373:dbl[])
                              n1735 = call "rotm_obs_new.vi"("angle[rad]"=w2398, "reverse"=TRUE, "y0"=w2400, "x0"=w2401, "y"=w2389, "x"=w2396) -> ("rot*(y-y0) 2"=w2394:dbl[], "rot*(x-x0)"=w2395:dbl[])  [unwired: 2 in, 2 out]
                              n1736 = call "rotm_obs_new.vi"("angle[rad]"=w2371, "reverse"=TRUE, "y0"=w2369, "x0"=w2368, "y"=w2380, "x"=w2373) -> ("rot*(y-y0) 2"=w2375:dbl[], "rot*(x-x0)"=w2374:dbl[])  [unwired: 2 in, 2 out]
                              n1737 = Build Array(w2395, w2394) -> (w2393:dbl[][])
                              n1738 = Build Array(w2374, w2375) -> (w2376:dbl[][])
                              n1739 = Transpose 2D Array(2D array=w2393) -> (transposed array=w2385:dbl[][])
                              n1740 = Transpose 2D Array(2D array=w2376) -> (transposed array=w2384:dbl[][])
                              n1741 = global write "G_PATH.vi" "lane_right"(w2385) -> ()
                              n1742 = global write "G_PATH.vi" "lane_left"(w2384) -> ()
                            }
                            frame True {
                              n1743 = local read "M6006"() -> (w2440:T1)
                              n1744 = local read "M6006"() -> (w2425:T1)
                              n1745 = local read "map_track"() -> (w2450:dbl[][])
                              n1746 = Unbundle By Name(w2440) -> ("lcc[1]"=w2444:dbl, "lcc[0]"=w2443:dbl, "attitude[2]"=w2442:dbl)
                              n1747 = local read "map_track"() -> (w2415:dbl[][])
                              n1748 = Unbundle By Name(w2425) -> ("lcc[1]"=w2421:dbl, "lcc[0]"=w2422:dbl, "attitude[2]"=w2423:dbl)
                              n1749 = Negate(x=w2442) -> (-x=w2441:dbl)
                              n1750 = Negate(x=w2423) -> (-x=w2424:dbl)
                              n1751 = Index Array(array=w2450, index (col)=1 ("disabled index (col)")) -> (element=w2434:dbl[])  [unwired: 1 in]
                              n1752 = Index Array(array=w2415, index (col)=1 ("disabled index (col)")) -> (element=w2431:dbl[])  [unwired: 1 in]
                              n1753 = local read "a"() -> (w2448:dbl)
                              n1754 = local read "a"() -> (w2417:dbl)
                              n1755 = Multiply(x=w2434, y=w2448) -> (x*y=w2447:dbl[])
                              n1756 = Multiply(x=w2431, y=w2417) -> (x*y=w2418:dbl[])
                              n1757 = local read "right"() -> (w2446:dbl)
                              n1758 = local read "left"() -> (w2419:dbl)
                              n1759 = Add(x=w2447, y=w2446) -> (x+y=w2445:dbl[])
                              n1760 = Add(x=w2418, y=w2419) -> (x+y=w2420:dbl[])
                              n1761 = Negate(x=w2445) -> (-x=w2439:dbl[])
                              n1762 = Negate(x=w2420) -> (-x=w2426:dbl[])
                              n1763 = call "rotm_obs_new.vi"("angle[rad]"=w2441, "reverse"=TRUE, "y0"=w2443, "x0"=w2444, "y"=w2434, "x"=w2439) -> ("rot*(y-y0) 2"=w2437:dbl[], "rot*(x-x0)"=w2438:dbl[])  [unwired: 2 in, 2 out]
                              n1764 = call "rotm_obs_new.vi"("angle[rad]"=w2424, "reverse"=TRUE, "y0"=w2422, "x0"=w2421, "y"=w2431, "x"=w2426) -> ("rot*(y-y0) 2"=w2428:dbl[], "rot*(x-x0)"=w2427:dbl[])  [unwired: 2 in, 2 out]
                              n1765 = Build Array(w2438, w2437) -> (w2436:dbl[][])
                              n1766 = Build Array(w2427, w2428) -> (w2429:dbl[][])
                              n1767 = Transpose 2D Array(2D array=w2436) -> (transposed array=w2433:dbl[][])
                              n1768 = Transpose 2D Array(2D array=w2429) -> (transposed array=w2432:dbl[][])
                              n1769 = global write "G_PATH.vi" "lane_right"(w2433) -> ()
                              n1770 = global write "G_PATH.vi" "lane_left"(w2432) -> ()
                            }
                          }
                        }
                      }
                    }
                  }
                }
              }
              n1771 = local read "cost"() -> (→"Waveform Chart":dbl)
            }
          }
        }
      }
    }
    frame #3 {
      n1772 = Tick Count (ms)() -> (millisecond timer value=w2456:u32)
      n1773 = Subtract(x=w2456, y=w2451) -> (x-y=w2455:u32)
      n1774 = To Double Precision Float(number=w2455) -> (double precision float=w2454:dbl)
      n1775 = Multiply(x=0.001, y=w2454) -> (x*y=→"time[sec]":dbl)
    }
  }
